vi "gyro-V4.vi"() -> ()   [LabVIEW 2017]
uses:
  plot refs -- filter related.ctl
  cursor winow.ctl
  cursor window action.ctl
  KM_file -- read-write control.ctl
  MFLI controller action.ctl
  sweep parameters.ctl
  cursor action.ctl
  four-corner circle transformation.ctl
  agregator -- action.ctl
  circle corners.ctl
  lorentzian.ctl
  filename-action.ctl
  file -- read-write control.ctl
  publisher action.ctl
  <vilib>/event_ctls.llb/eventvkey.ctl
  wavepacket.ctl
  filter method control.ctl
  peak -- parameters -- complex fit.ctl
  parameters -- scan monitor control.ctl
  pid -- parameters.ctl
panel:
  out "read freq (Hz)":dbl=43834.543279430705 format="%-#11_11f"
  in  "all":enum32{"all", "other"}(tab)
  in  "subtract bgnd !":bool=TRUE
  out "Plot: circle sweep window":cluster{"all rows":dbl[], "all rows":dbl[]}[](graph)
  in  "MFLI mode":T1(tab)=enum."read from disk"
  out "fit is fine":bool=TRUE
  in  "gamma factor":dbl=1.6
  in  "Auto-update sweep window!":bool
  in  "scan type":enum16{"linear", "arctan"}(ring)
  in  "N":i64=2357
  out "sweep time (sec)":dbl=0.07489956999779679
  in  "control sweep!":bool
  out "circle frequency (Hz)":dbl format="%#11_11f"
  out "circle gamma (Hz)":dbl format="%#11_11f"
  out "circle phase (rad)":dbl=nan format="%#11_11f"
  out "circle Q":dbl=nan format="%#11_11f"
  in  "history length":i32=5
  in  "delay-circle(msec)":i64
  out "read Voltage (V)":cdb=8.437092120710226e-06+0.006122499694529841i format="%#10_10f"
  in  "read !":bool
  out "read Voltage X (V)":dbl=8.437092120710226e-06 format="%#11_11f"
  out "read Voltage Y (V)":dbl=0.006122499694529841 format="%#11_11f"
  in  "delay-read (msec)":i64=300
  in  "reqested size":i64=30
  in  "refresh":bool=TRUE
  in  "PID parameters":T2={"P (sec)"=60.0, "I (sec)"=10.0}
  out "left freq (Hz)":dbl=1094842.7980648028
  out "right freq (Hz)":dbl=1109968.9974186728
  out "center freq (Hz)":dbl=1102405.8977417378
  out "window  (Hz)":dbl=15126.199353870004
  in  "talk to MFLI !":bool=TRUE
  in  "aggregator action":T3
  in  "Tab : everything":T4(tab)
  in  "Tab :  Fit controls":enum32{"complex plane", "complex plane 2"}(tab)
  in  "some":dbl=3225.0
  in  "Plot: fragment - filter":cluster{dbl[], dbl[]}[](graph)=[{[], []}, {[], []}, {[], []}, {[], []}]
  in  "scale gauge: Plot: complex plane - filter":dbl(slide)=0.00015000000000000001 min=0.0 max=0.3 step=1e-05 scale=0.0001..0.3 scale format="%#_5g"
  in  "Plot: complex plane - filter":cluster{dbl[], dbl[]}[](graph)=[{[], []}, {[], []}, {[0.0, 0.0, 0.0, 0.0, 0.0, 0.0, 0.0, 0.0, 0.0, 0.0, 0.0, 0.0, 0.0, 0.0, 0.0, 0.0, 0.0, 0.0, 0.0, 0.0, 0.0, 0.0, 0.0, 0.0, 0.0, 0.0, 0.0, 0.0, 0.0, 0.0, 0.0, 0.0, 0.0, 0.0, 0.0, 0.0, 0.0, 0.0, 0.0, 0.0, 0.0, 0.0, 0.0, 0.0, 0.0, 0.0, 0.0, 0.0, 0.0, 0.0, 0.0, 0.0, 0.0, 0.0, 0.0, 0.0, 0.0, 0.0, 0.0, 0.0, 0.0, 0.0, 0.0, 0.0, 0.0, 0.0, 0.0, 0.0, 0.0, 0.0, 0.0, 0.0, 0.0, 0.0, 0.0, 0.0, 0.0, 0.0, 0.0, 0.0, 0.0, 0.0, 0.0, 0.0, 0.0, 0.0, 0.0, 0.0, 0.0, 0.0, 0.0, 0.0, 0.0, 0.0, 0.0, 0.0, 0.0, 0.0, 0.0, 0.0], [0.0, 0.0, 0.0, 0.0, 0.0, 0.0, 0.0, 0.0, 0.0, 0.0, 0.0, 0.0, 0.0, 0.0, 0.0, 0.0, 0.0, 0.0, 0.0, 0.0, 0.0, 0.0, 0.0, 0.0, 0.0, 0.0, 0.0, 0.0, 0.0, 0.0, 0.0, 0.0, 0.0, 0.0, 0.0, 0.0, 0.0, 0.0, 0.0, 0.0, 0.0, 0.0, 0.0, 0.0, 0.0, 0.0, 0.0, 0.0, 0.0, 0.0, 0.0, 0.0, 0.0, 0.0, 0.0, 0.0, 0.0, 0.0, 0.0, 0.0, 0.0, 0.0, 0.0, 0.0, 0.0, 0.0, 0.0, 0.0, 0.0, 0.0, 0.0, 0.0, 0.0, 0.0, 0.0, 0.0, 0.0, 0.0, 0.0, 0.0, 0.0, 0.0, 0.0, 0.0, 0.0, 0.0, 0.0, 0.0, 0.0, 0.0, 0.0, 0.0, 0.0, 0.0, 0.0, 0.0, 0.0, 0.0, 0.0, 0.0]}, {[0.0, 0.0, 0.0], [0.0, 0.0, 0.0]}, {[nan, nan, nan, nan, nan, nan, nan, nan, nan, nan, nan, nan, nan, nan, nan, nan, nan, nan, nan, nan], [nan, nan, nan, nan, nan, nan, nan, nan, nan, nan, nan, nan, nan, nan, nan, nan, nan, nan, nan, nan]}, {[0.0, 0.0, 0.0, 0.0, 0.0, 0.0, 0.0, 0.0, 0.0, 0.0, 0.0, 0.0, 0.0, 0.0, 0.0, 0.0, 0.0, 0.0, 0.0, 0.0], [0.0, 0.0, 0.0, 0.0, 0.0, 0.0, 0.0, 0.0, 0.0, 0.0, 0.0, 0.0, 0.0, 0.0, 0.0, 0.0, 0.0, 0.0, 0.0, 0.0]}]
  out "Plot: dz/domega":cluster{"omega out":dbl[], dbl[]}(graph)
  out "Plot: win omega":T5(graph)
  out "Plot: phase":cluster{"omega out":dbl[], dbl[]}(graph)
  out "Plot: phase around center":cluster{dbl[], dbl[]}[](graph)
  out "Plot: fragment":cluster{dbl[], dbl[]}[](graph)
  out "Plot: complex plane":cluster{dbl[], dbl[]}[](graph)=[{[], []}, {[nan, nan, nan, nan, nan, nan, nan, nan, nan, nan, nan, nan, nan, nan, nan, nan, nan, nan, nan, nan, nan, nan, nan, nan, nan, nan, nan, nan, nan, nan, nan, nan, nan, nan, nan, nan, nan, nan, nan, nan, nan, nan, nan, nan, nan, nan, nan, nan, nan, nan], [nan, nan, nan, nan, nan, nan, nan, nan, nan, nan, nan, nan, nan, nan, nan, nan, nan, nan, nan, nan, nan, nan, nan, nan, nan, nan, nan, nan, nan, nan, nan, nan, nan, nan, nan, nan, nan, nan, nan, nan, nan, nan, nan, nan, nan, nan, nan, nan, nan, nan]}, {[nan, nan, nan, nan, nan, nan, nan, nan, nan, nan, nan, nan, nan, nan, nan, nan, nan, nan, nan, nan], [nan, nan, nan, nan, nan, nan, nan, nan, nan, nan, nan, nan, nan, nan, nan, nan, nan, nan, nan, nan]}, {[nan, nan, nan, nan, nan, nan, nan, nan, nan, nan, nan, nan, nan, nan, nan, nan, nan, nan, nan, nan], [nan, nan, nan, nan, nan, nan, nan, nan, nan, nan, nan, nan, nan, nan, nan, nan, nan, nan, nan, nan]}, {[nan, nan, nan, nan, nan, nan, nan, nan, nan, nan, nan, nan, nan, nan, nan, nan, nan, nan, nan, nan], [nan, nan, nan, nan, nan, nan, nan, nan, nan, nan, nan, nan, nan, nan, nan, nan, nan, nan, nan, nan]}, {[nan, nan, nan, nan, nan, nan, nan, nan, nan, nan, nan, nan, nan, nan, nan, nan, nan, nan, nan, nan], [nan, nan, nan, nan, nan, nan, nan, nan, nan, nan, nan, nan, nan, nan, nan, nan, nan, nan, nan, nan]}, {[], []}]
  in  "scale gauge: Plot: complex plane":dbl(slide)=0.00025 min=0.0 max=0.3 step=1e-05 scale=0.0001..1.0 scale format="%#_2g"
  out "window width (kHz)":dbl=76.27809365793496
  out "window center (kHz)":dbl=3399.029286744401
  out "# of points in window":dbl=953.475933538175
  in  "use fast fit?":bool
  out "pm lorentzian":T6={"Amplitude"=nan, "omega(0)"=0.0, "Gamma"=0.0, "phase"=nan, "Q"=nan, "Norm  Ampl"=nan, "z (inf)"=nan+nani, "4corners"={"z (-pi/2)"=nan+nani, "z(inf)"=nan+nani, "z (pi/2)"=nan+nani, "z center"=nan+nani, "z(0)"=nan+nani, "radius"=nan}} {"z (inf)" format="%#9_9f"; "Q" format="%#9_9f"; "phase" format="%#9_9f"; "Gamma" format="%#9_9f"; "omega(0)" format="%#9_9f"}
  in  "plot staff":enum16{"plot", "do not plot", "a"}(ring)
  in  "fit?":bool=TRUE
  out "Freq out":dbl[](array[numeric])=[17015.929848298583, 17103.637448201425, 17191.34504831743, 17279.052648433433, 17366.76024833628, 17454.46784845228, 17542.175448355123, 17629.88304847113, 17717.590648587135, 17805.298248489977, 17893.00584860598, 17980.713448721985, 18068.421048624827, 18156.128648740832, 18243.83624885684, 18331.54384875968, 18419.251448875686, 18506.959048991688, 18594.66664889453, 18682.374249010536, 18770.08184912654, 18857.789449029384, 18945.497049145386, 19033.20464926139, 19120.912249164234, 19208.61984928024, 19296.32744918308, 19384.035049299087, 19471.742649415093, 19559.45024931793, 19647.157849433937, 19734.865449549943, 19822.573049452785, 19910.28064956879, 19997.988249684793, 20085.69584958764, 20173.40344970364, 20261.111049819647, 20348.81864972249, 20436.526249838495, 20524.2338499545, 20611.94144985734, 20699.649049973345, 20787.356649876187, 20875.064249992192, 20962.771850108198, 21050.47945001104, 21138.187050127046, 21225.894650243048, 21313.60225014589, 21401.309850261896, 21489.0174503779, 21576.725050280744, 21664.432650396746, 21752.14025051275, 21839.847850415594, 21927.5554505316, 22015.263050647605, 22102.970650550447, 22190.678250666453, 22278.38585056929, 22366.093450685297, 22453.801050801303, 22541.508650704145, 22629.21625082015, 22716.923850936153, 22804.631450839, 22892.339050955, 22980.046651071007, 23067.75425097385, 23155.461851089854, 23243.16945120586, 23330.8770511087, 23418.584651224704, 23506.29225134071, 23593.999851243552, 23681.707451359558, 23769.4150512624, 23857.122651378406, 23944.830251494408, 24032.53785139725, 24120.245451513256, 24207.95305162926, 24295.660651532104, 24383.368251648106, 24471.07585176411, 24558.783451666954, 24646.49105178296, 24734.198651898965, 24821.906251801807, 24909.613851917813, 24997.321452033815, 25085.029051936657, 25172.736652052663, 25260.444251955505, 25348.15185207151, 25435.859452187513, 25523.56705209036, 25611.27465220636, 25698.982252322367, 25786.68985222521, 25874.397452341214, 25962.10505245722, 26049.81265236006, 26137.520252476064, 26225.22785259207, 26312.935452494912, 26400.643052610918, 26488.35065272692, 26576.058252629766, 26663.765852745768, 26751.473452861774, 26839.181052764616, 26926.88865288062, 27014.596252783464, 27102.303852899466, 27190.01145301547, 27277.719052918314, 27365.42665303432, 27453.134253150325, 27540.841853053167, 27628.549453169173, 27716.257053285175, 27803.964653188017, 27891.672253304023, 27979.37985342003, 28067.08745332287, 28154.795053438873, 28242.50265355488, 28330.21025345772, 28417.917853573726, 28505.62545347657, 28593.333053592574, 28681.04065370858, 28768.74825361142, 28856.455853727424, 28944.16345384343, 29031.871053746272, 29119.578653862278, 29207.28625397828, 29294.993853881126, 29382.701453997128, 29470.409054113134, 29558.116654015976, 29645.82425413198, 29733.531854247987, 29821.239454150826, 29908.94705426683, 29996.654654169673, 30084.36225428568, 30172.069854401685, 30259.777454304527, 30347.485054420533, 30435.192654536535, 30522.900254439377, 30610.607854555383, 30698.31545467139, 30786.02305457423, 30873.730654690233, 30961.43825480624, 31049.14585470908, 31136.853454825086, 31224.561054941092, 31312.268654843934, 31399.97625495994, 31487.68385486278, 31575.391454978784, 31663.09905509479, 31750.806654997632, 31838.514255113638, 31926.22185522964, 32013.929455132486, 32101.637055248488, 32189.344655364494, 32277.052255267336, 32364.75985538334, 32452.467455499347, 32540.175055402186, 32627.88265551819, 32715.590255634197, 32803.297855537036, 32891.005455653045, 32978.71305555588, 33066.42065567189, 33154.128255787895, 33241.83585569074, 33329.54345580674, 33417.251055922745, 33504.95865582559, 33592.66625594159, 33680.3738560576, 33768.08145596044, 33855.78905607645, 33943.49665619245, 34031.20425609529, 34118.9118562113, 34206.6194563273, 34294.32705623015, 34382.03465634615, 34469.74225646215, 34557.449856365, 34645.157456481, 34732.865056383846, 34820.57265649985, 34908.28025661585, 34995.987856518695, 35083.6954566347, 35171.40305675071, 35259.110656653545, 35346.818256769555, 35434.52585688556, 35522.233456788395, 35609.941056904405, 35697.64865702041, 35785.35625692325, 35873.063857039255, 35960.771457155264, 36048.4790570581, 36136.186657174105, 36223.89425707695, 36311.60185719295, 36399.30945730896, 36487.0170572118, 36574.72465732781, 36662.43225744381, 36750.13985734665, 36837.84745746266, 36925.55505757866, 37013.26265748151, 37100.97025759751, 37188.67785771351, 37276.38545761636, 37364.09305773236, 37451.80065784837, 37539.50825775121, 37627.21585786721, 37714.923457770055, 37802.63105788606, 37890.33865800207, 37978.046257904905, 38065.753858020915, 38153.46145813692, 38241.169058039755, 38328.876658155765, 38416.58425827177, 38504.29185817461, 38591.999458290615, 38679.707058406624, 38767.41465830946, 38855.122258425465, 38942.829858541474, 39030.53745844431, 39118.24505856032, 39205.95265846316, 39293.66025857917, 39381.36785869517, 39469.07545859801, 39556.78305871402, 39644.49065883002, 39732.19825873287, 39819.90585884887, 39907.61345896487, 39995.32105886772, 40083.02865898372, 40170.73625909973, 40258.44385900257, 40346.15145911857, 40433.85905923458, 40521.56665913742, 40609.27425925343, 40696.981859156265, 40784.689459272275, 40872.39705938828, 40960.104659291115, 41047.812259407125, 41135.51985952313, 41223.22745942597, 41310.935059541975, 41398.642659657984, 41486.35025956082, 41574.057859676825, 41661.765459792834, 41749.47305969567, 41837.18065981168, 41924.888259927684, 42012.59585983053, 42100.30345994653, 42188.01105984937, 42275.71865996538, 42363.42626008138, 42451.13385998423, 42538.84146010023, 42626.54906021623, 42714.25666011908, 42801.96426023508, 42889.67186035109, 42977.37946025393, 43065.08706036993, 43152.79466048594, 43240.50226038878, 43328.20986050479, 43415.91746062079, 43503.625060523635, 43591.33266063964, 43679.04026075564, 43766.747860658485, 43854.45546077449, 43942.16306067733, 44029.870660793335, 44117.578260909344, 44205.28586081218, 44292.993460928185, 44380.701061044194, 44468.40866094703, 44556.11626106304, 44643.823861179044, 44731.53146108189, 44819.23906119789, 44906.946661313894, 44994.65426121674, 45082.36186133274, 45170.069461448744, 45257.77706135159, 45345.48466146759, 45433.19226137044, 45520.89986148644, 45608.60746160245, 45696.31506150529, 45784.02266162129, 45871.7302617373, 45959.43786164014, 46047.14546175615, 46134.85306187215, 46222.560661774995, 46310.268261891, 46397.975862007, 46485.683461909844, 46573.39106202585, 46661.098662141856, 46748.806262044694, 46836.513862160704, 46924.22146206354, 47011.929062179544, 47099.636662295554, 47187.34426219839, 47275.0518623144, 47362.759462430404, 47450.46706233325, 47538.17466244925, 47625.882262565254, 47713.5898624681, 47801.2974625841, 47889.005062700104, 47976.71266260295, 48064.42026271895, 48152.12786283496, 48239.8354627378, 48327.54306285381, 48415.25066275665, 48502.95826287265, 48590.66586298866, 48678.3734628915, 48766.08106300751, 48853.78866312351, 48941.496263026354, 49029.20386314236, 49116.91146325836, 49204.619063161204, 49292.32666327721, 49380.034263393216, 49467.741863296054, 49555.449463412064, 49643.157063528066, 49730.864663430904, 49818.572263546914, 49906.27986344975, 49993.98746356576, 50081.695063681764, 50169.40266358461, 50257.11026370061, 50344.817863816614, 50432.52546371946, 50520.23306383546, 50607.940663951464, 50695.64826385431, 50783.35586397031, 50871.06346408632, 50958.77106398916, 51046.47866410517, 51134.18626422117, 51221.89386412401, 51309.60146424002, 51397.30906435602, 51485.01666425887, 51572.72426437487, 51660.431864277714, 51748.13946439372, 51835.84706450972, 51923.554664412564, 52011.26226452857, 52098.969864644576, 52186.677464547414, 52274.385064663424, 52362.092664779426, 52449.800264682264, 52537.507864798274, 52625.215464914276, 52712.92306481712, 52800.63066493312, 52888.338265049126, 52976.04586495197, 53063.75346506797, 53151.46106497082, 53239.16866508682, 53326.87626520282, 53414.58386510567, 53502.29146522167, 53589.99906533768, 53677.70666524052, 53765.41426535653, 53853.12186547253, 53940.82946537537, 54028.53706549138, 54116.24466560738, 54203.95226551023, 54291.65986562623, 54379.36746574224, 54467.07506564508, 54554.78266576108, 54642.490265663924, 54730.197865779926, 54817.905465895936, 54905.613065798774, 54993.32066591478, 55081.028266030786, 55168.735865933624, 55256.44346604963, 55344.151066165636, 55431.85866606848, 55519.56626618448, 55607.273866300486, 55694.98146620333, 55782.68906631933, 55870.39666643534, 55958.10426633818, 56045.81186645418, 56133.51946635703, 56221.22706647303, 56308.93466658904, 56396.64226649188, 56484.34986660789, 56572.05746672389, 56659.76506662673, 56747.47266674274, 56835.18026685874, 56922.887866761586, 57010.59546687759, 57098.3030669936, 57186.010666896436, 57273.71826701244, 57361.42586712845, 57449.133467031286, 57536.841067147296, 57624.548667050134, 57712.25626716614, 57799.963867282146, 57887.671467184984, 57975.37906730099, 58063.086667416996, 58150.79426731984, 58238.50186743584, 58326.209467551846, 58413.91706745469, 58501.62466757069, 58589.3322676867, 58677.03986758954, 58764.74746770554, 58852.45506782155, 58940.16266772439, 59027.8702678404, 59115.5778679564, 59203.28546785925, 59290.99306797525, 59378.70066787809, 59466.4082679941, 59554.1158681101, 59641.823468012946, 59729.53106812895, 59817.23866824496, 59904.946268147796, 59992.6538682638, 60080.36146837981, 60168.069068282646, 60255.776668398656, 60343.48426851466, 60431.1918684175, 60518.899468533506, 60606.60706864951, 60694.31466855235, 60782.022268668356, 60869.7298685712, 60957.4374686872, 61045.145068803206, 61132.85266870605, 61220.56026882205, 61308.26786893806, 61395.9754688409, 61483.6830689569, 61571.39066907291, 61659.09826897575, 61746.80586909176, 61834.51346920776, 61922.22106911061, 62009.92866922661, 62097.63626934261, 62185.34386924546, 62273.05146936146, 62360.759069264306, 62448.46666938031, 62536.17426949632, 62623.881869399156, 62711.58946951516, 62799.29706963117, 62887.004669534006, 62974.712269650016, 63062.41986976602, 63150.12746966886, 63237.835069784865, 63325.54266990087, 63413.25026980371, 63500.957869919715, 63588.66547003572, 63676.37306993856, 63764.080670054565, 63851.78826995741, 63939.49587007341, 64027.20347018942, 64114.91107009226, 64202.61867020826, 64290.32627032427, 64378.03387022711, 64465.74147034312, 64553.44907045912, 64641.15667036197, 64728.86427047797, 64816.57187059397, 64904.27947049682, 64991.98707061282, 65079.69467072883, 65167.40227063167, 65255.10987074768, 65342.817470650516, 65430.52507076652, 65518.23267088253, 65605.94027078537, 65693.64787090138, 65781.35547101738, 65869.06307092022, 65956.77067103623, 66044.47827115223, 66132.18587105507, 66219.89347117108, 66307.60107128708, 66395.30867118992, 66483.01627130593, 66570.72387142193, 66658.43147132477, 66746.13907144078, 66833.84667155679, 66921.55427145962, 67009.26187157563, 67096.96947147847, 67184.67707159447, 67272.38467171049, 67360.09227161332, 67447.79987172934, 67535.50747184534, 67623.21507174817, 67710.92267186419, 67798.63027198019, 67886.33787188304, 67974.04547199904, 68061.75307211504, 68149.46067201789, 68237.16827213389, 68324.87587224989, 68412.58347215274, 68500.29107226874, 68587.99867217158, 68675.70627228759, 68763.41387240359, 68851.12147230643, 68938.82907242244, 69026.53667253844, 69114.24427244128, 69201.95187255729, 69289.65947267329, 69377.36707257613, 69465.07467269214, 69552.78227280814, 69640.48987271098, 69728.19747282699, 69815.905072943, 69903.61267284583, 69991.32027296185, 70079.02787286468, 70166.73547298068, 70254.4430730967, 70342.15067299953, 70429.85827311555, 70517.56587323155, 70605.2734731344, 70692.9810732504, 70780.6886733664, 70868.39627326925, 70956.10387338525, 71043.81147350125, 71131.5190734041, 71219.2266735201, 71306.9342736361, 71394.64187353895, 71482.34947365495, 71570.0570735578, 71657.7646736738, 71745.4722737898, 71833.17987369264, 71920.88747380865, 72008.59507392465, 72096.3026738275, 72184.0102739435, 72271.71787405951, 72359.42547396234, 72447.13307407835, 72534.84067419436, 72622.5482740972, 72710.25587421321, 72797.96347432921, 72885.67107423206, 72973.37867434806, 73061.08627425089, 73148.79387436691, 73236.50147448291, 73324.20907438576, 73411.91667450176, 73499.62427461776, 73587.3318745206, 73675.03947463661, 73762.74707475261, 73850.45467465546, 73938.16227477146, 74025.86987488746, 74113.5774747903, 74201.2850749063, 74288.99267502231, 74376.70027492516, 74464.40787504116, 74552.11547515716, 74639.82307506, 74727.530675176, 74815.23827507885, 74902.94587519486, 74990.65347531086, 75078.3610752137, 75166.0686753297, 75253.77627544572, 75341.48387534855, 75429.19147546457, 75516.89907558057, 75604.6066754834, 75692.31427559942, 75780.02187571542, 75867.72947561827, 75955.43707573427, 76043.14467585027, 76130.85227575312, 76218.55987586912, 76306.26747577197, 76393.97507588797, 76481.68267600397, 76569.39027590682, 76657.09787602282, 76744.80547613882, 76832.51307604167, 76920.22067615767, 77007.92827627367, 77095.63587617652, 77183.34347629252, 77271.05107640852, 77358.75867631136, 77446.46627642737, 77534.17387654338, 77621.88147644621, 77709.58907656223, 77797.29667646506, 77885.00427658106, 77972.71187669708, 78060.41947659991, 78148.12707671593, 78235.83467683193, 78323.54227673478, 78411.24987685078, 78498.95747696678, 78586.66507686963, 78674.37267698563, 78762.08027710163, 78849.78787700448, 78937.49547712048, 79025.20307723648, 79112.91067713933, 79200.61827725533, 79288.32587715817, 79376.03347727418, 79463.74107739018, 79551.44867729302, 79639.15627740903, 79726.86387752503, 79814.57147742787, 79902.27907754388, 79989.98667765988, 80077.69427756272, 80165.40187767873, 80253.10947779474, 80340.81707769757, 80428.52467781358, 80516.2322779296, 80603.93987783242, 80691.64747794844, 80779.35507785127, 80867.06267796729, 80954.77027808329, 81042.47787798612, 81130.18547810214, 81217.89307821814, 81305.60067812099, 81393.30827823699, 81481.01587835299, 81568.72347825584, 81656.43107837184, 81744.13867848784, 81831.84627839069, 81919.55387850669, 82007.26147862269, 82094.96907852554, 82182.67667864154, 82270.38427854438, 82358.09187866039, 82445.79947877639, 82533.50707867923, 82621.21467879524, 82708.92227891124, 82796.62987881408, 82884.33747893009, 82972.0450790461, 83059.75267894893, 83147.46027906495, 83235.16787918095, 83322.87547908378, 83410.5830791998, 83498.2906793158, 83585.99827921865, 83673.70587933465, 83761.41347945065, 83849.1210793535, 83936.8286794695, 84024.53627937235, 84112.24387948835, 84199.95147960435, 84287.6590795072, 84375.3666796232, 84463.0742797392, 84550.78187964205, 84638.48947975805, 84726.19707987405, 84813.9046797769, 84901.6122798929, 84989.3198800089, 85077.02747991175, 85164.73508002775, 85252.44268014375, 85340.1502800466, 85427.8578801626, 85515.56548006544, 85603.27308018145, 85690.98068029746, 85778.6882802003, 85866.3958803163, 85954.10348043231, 86041.81108033514, 86129.51868045116, 86217.22628056716, 86304.93388047001, 86392.64148058601, 86480.34908070201, 86568.05668060486, 86655.76428072086, 86743.47188083686, 86831.17948073971, 86918.88708085571, 87006.59468075856, 87094.30228087456, 87182.00988099056, 87269.7174808934, 87357.42508100941, 87445.13268112541, 87532.84028102826, 87620.54788114426, 87708.25548126026, 87795.9630811631, 87883.67068127911, 87971.37828139513, 88059.08588129796, 88146.79348141396, 88234.50108152998, 88322.2086814328, 88409.91628154882, 88497.62388145165, 88585.33148156767, 88673.03908168367, 88760.7466815865, 88848.45428170252, 88936.16188181852, 89023.86948172137, 89111.57708183737, 89199.28468195337, 89286.99228185622, 89374.69988197222, 89462.40748208822, 89550.11508199107, 89637.82268210707, 89725.53028222307, 89813.23788212592, 89900.94548224192, 89988.65308214477, 90076.36068226077, 90164.06828237677, 90251.77588227962, 90339.48348239562, 90427.19108251162, 90514.89868241447, 90602.60628253047, 90690.31388264647, 90778.02148254932, 90865.72908266532, 90953.43668278134, 91041.14428268417, 91128.85188280018, 91216.55948291619, 91304.26708281902, 91391.97468293503, 91479.68228305104, 91567.38988295388, 91655.09748306988, 91742.80508297273, 91830.51268308873, 91918.22028320473, 92005.92788310758, 92093.63548322358, 92181.34308333958, 92269.05068324243, 92356.75828335843, 92444.46588347443, 92532.17348337728, 92619.88108349328, 92707.58868360928, 92795.29628351213, 92883.00388362813, 92970.71148374413, 93058.41908364698, 93146.12668376298, 93233.83428366583, 93321.54188378183, 93409.24948389785, 93496.95708380068, 93584.66468391668, 93672.3722840327, 93760.07988393553, 93847.78748405154, 93935.49508416755, 94023.20268407039, 94110.9102841864, 94198.6178843024, 94286.32548420524, 94374.03308432124, 94461.74068443725, 94549.44828434009, 94637.1558844561, 94724.86348435894, 94812.57108447494, 94900.27868459094, 94987.98628449379, 95075.69388460979, 95163.4014847258, 95251.10908462864, 95338.81668474464, 95426.52428486064, 95514.23188476349, 95601.93948487949, 95689.6470849955, 95777.35468489834, 95865.06228501434, 95952.76988513036, 96040.47748503319, 96128.18508514919, 96215.89268505204, 96303.60028516804, 96391.30788528406, 96479.01548518689, 96566.7230853029, 96654.4306854189, 96742.13828532174, 96829.84588543775, 96917.55348555376, 97005.2610854566, 97092.9686855726, 97180.6762856886, 97268.38388559145, 97356.09148570745, 97443.79908582346, 97531.5066857263, 97619.2142858423, 97706.92188574515, 97794.62948586115, 97882.33708597715, 97970.04468588, 98057.752285996, 98145.459886112, 98233.16748601485, 98320.87508613085, 98408.58268624685, 98496.2902861497, 98583.9978862657, 98671.70548638172, 98759.41308628455, 98847.12068640057, 98934.82828651657, 99022.5358864194, 99110.24348653542, 99197.95108665142, 99285.65868655426, 99373.36628667027, 99461.07388657311, 99548.78148668911, 99636.48908680512, 99724.19668670796, 99811.90428682396, 99899.61188693997, 99987.31948684281, 100075.02708695881, 100162.73468707482, 100250.44228697766, 100338.14988709366, 100425.85748720967, 100513.56508711251, 100601.27268722851, 100688.98028734452, 100776.68788724736, 100864.39548736336, 100952.10308726621, 101039.81068738221, 101127.51828749821, 101215.22588740106, 101302.93348751706, 101390.64108763308, 101478.34868753591, 101566.05628765191, 101653.76388776793, 101741.47148767076, 101829.17908778678, 101916.88668790278, 102004.59428780562, 102092.30188792163, 102180.00948803763, 102267.71708794047, 102355.42468805648, 102443.13228795932, 102530.83988807532, 102618.54748819133, 102706.25508809417, 102793.96268821017, 102881.67028832618, 102969.37788822902, 103057.08548834502, 103144.79308846103, 103232.50068836387, 103320.20828847987, 103407.91588859588, 103495.62348849872, 103583.33108861472, 103671.03868873074, 103758.74628863357, 103846.45388874957, 103934.16148865242, 104021.86908876842, 104109.57668888444, 104197.28428878727, 104284.99188890329, 104372.69948901929, 104460.40708892212, 104548.11468903814, 104635.82228915414, 104723.52988905698, 104811.23748917299, 104898.94508928899, 104986.65268919183, 105074.36028930784, 105162.06788942384, 105249.77548932668, 105337.48308944269, 105425.19068934553, 105512.89828946153, 105600.60588957753, 105688.31348948038, 105776.02108959638, 105863.72868971238, 105951.43628961523, 106039.14388973123, 106126.85148984723, 106214.55908975008, 106302.26668986608, 106389.97428998208, 106477.68188988493, 106565.38949000093, 106653.09709011695, 106740.80469001978, 106828.5122901358, 106916.2198902518, 107003.92749015463, 107091.63509027065, 107179.34269017348, 107267.0502902895, 107354.7578904055, 107442.46549030834, 107530.17309042434, 107617.88069054035, 107705.5882904432, 107793.2958905592, 107881.0034906752, 107968.71109057804, 108056.41869069404, 108144.12629081005, 108231.8338907129, 108319.5414908289, 108407.2490909449, 108494.95669084774, 108582.66429096374, 108670.37189086659, 108758.07949098259, 108845.7870910986, 108933.49469100144, 109021.20229111744, 109108.90989123346, 109196.61749113629, 109284.32509125229, 109372.03269136831, 109459.74029127114, 109547.44789138716, 109635.15549150316, 109722.863091406, 109810.570691522, 109898.27829163801, 109985.98589154085, 110073.69349165686, 110161.4010915597, 110249.1086916757, 110336.8162917917, 110424.52389169455, 110512.23149181055, 110599.93909192656, 110687.6466918294, 110775.3542919454, 110863.0618920614, 110950.76949196425, 111038.47709208025, 111126.18469219626, 111213.8922920991, 111301.5998922151, 111389.3074923311, 111477.01509223395, 111564.72269234995, 111652.4302922528, 111740.1378923688, 111827.8454924848, 111915.55309238765, 112003.26069250365, 112090.96829261967, 112178.6758925225, 112266.38349263852, 112354.09109275452, 112441.79869265735, 112529.50629277337, 112617.21389288937, 112704.92149279221, 112792.62909290822, 112880.33669302422, 112968.04429292706, 113055.75189304307, 113143.45949294591, 113231.16709306191, 113318.87469317792, 113406.58229308076, 113494.28989319676, 113581.99749331277, 113669.70509321561, 113757.41269333161, 113845.12029344762, 113932.82789335046, 114020.53549346646, 114108.24309358247, 114195.95069348531, 114283.65829360131, 114371.36589371733, 114459.07349362016, 114546.78109373618, 114634.48869385218, 114722.19629375501, 114809.90389387103, 114897.61149377386, 114985.31909388988, 115073.02669400588, 115160.73429390872, 115248.44189402473, 115336.14949414073, 115423.85709404357, 115511.56469415958, 115599.27229427558, 115686.97989417842, 115774.68749429443, 115862.39509441043, 115950.10269431327, 116037.81029442928, 116125.51789454528, 116213.22549444812, 116300.93309456413, 116388.64069446697, 116476.34829458297, 116564.05589469898, 116651.76349460182, 116739.47109471782, 116827.17869483383, 116914.88629473667, 117002.59389485267, 117090.30149496869, 117178.00909487152, 117265.71669498752, 117353.42429510354, 117441.13189500637, 117528.83949512239, 117616.54709523839, 117704.25469514124, 117791.96229525724, 117879.66989516007, 117967.37749527609, 118055.08509539209, 118142.79269529493, 118230.50029541094, 118318.20789552694, 118405.91549542978, 118493.62309554579, 118581.33069566179, 118669.03829556463, 118756.74589568064, 118844.45349579664, 118932.16109569948, 119019.86869581549, 119107.57629593149, 119195.28389583433, 119282.99149595034, 119370.69909585318, 119458.40669596918, 119546.11429608519, 119633.82189598803, 119721.52949610403, 119809.23709622005, 119896.94469612288, 119984.6522962389, 120072.3598963549, 120160.06749625773, 120247.77509637375, 120335.48269648975, 120423.1902963926, 120510.8978965086, 120598.6054966246, 120686.31309652745, 120774.02069664345, 120861.7282965463, 120949.4358966623, 121037.1434967783, 121124.85109668114, 121212.55869679715, 121300.26629691315, 121387.973896816, 121475.681496932, 121563.389097048, 121651.09669695084, 121738.80429706685, 121826.51189718285, 121914.2194970857, 122001.9270972017, 122089.6346973177, 122177.34229722054, 122265.04989733655, 122352.75749723939, 122440.4650973554, 122528.17269747141, 122615.88029737424, 122703.58789749024, 122791.29549760626, 122879.00309750909, 122966.71069762511, 123054.41829774111, 123142.12589764396, 123229.83349775996, 123317.54109787596, 123405.2486977788, 123492.95629789481, 123580.66389801081, 123668.37149791366, 123756.07909802966, 123843.78669814566, 123931.4942980485, 124019.20189816451, 124106.90949806735, 124194.61709818336, 124282.32469829936, 124370.0322982022, 124457.7398983182, 124545.44749843421, 124633.15509833705, 124720.86269845306, 124808.57029856907, 124896.2778984719, 124983.9854985879, 125071.69309870392, 125159.40069860675, 125247.10829872277, 125334.81589883877, 125422.52349874162, 125510.23109885762, 125597.93869876045, 125685.64629887647, 125773.35389899247, 125861.06149889532, 125948.76909901132, 126036.47669912732, 126124.18429903017, 126211.89189914617, 126299.59949926217, 126387.30709916502, 126475.01469928102, 126562.72229939702, 126650.42989929987, 126738.13749941587, 126825.84509953187, 126913.55269943472, 127001.26029955072, 127088.96789945356, 127176.67549956957, 127264.38309968557, 127352.09069958841, 127439.79829970442, 127527.50589982042, 127615.21349972326, 127702.92109983927, 127790.62869995528, 127878.33629985811, 127966.04389997413, 128053.75150009013, 128141.45909999296, 128229.16670010898, 128316.87430022498, 128404.58190012783, 128492.28950024383, 128579.99710014668, 128667.70470026268, 128755.41230037868, 128843.11990028153, 128930.82750039753, 129018.53510051353, 129106.24270041638, 129193.95030053238, 129281.65790064838, 129369.36550055123, 129457.07310066723, 129544.78070078323, 129632.48830068608, 129720.19590080208, 129807.90350091808, 129895.61110082093, 129983.31870093693, 130071.02630083977, 130158.73390095578, 130246.4415010718, 130334.14910097462, 130421.85670109063, 130509.56430120664, 130597.27190110947, 130684.97950122549, 130772.6871013415, 130860.39470124434, 130948.10230136034, 131035.80990147634, 131123.5175013792, 131211.2251014952, 131298.9327016112, 131386.64030151404, 131474.34790163004, 131562.05550174604, 131649.7631016489, 131737.4707017649, 131825.17830166774, 131912.88590178374, 132000.59350189974, 132088.3011018026, 132176.0087019186, 132263.7163020346, 132351.42390193744, 132439.13150205344, 132526.83910216944, 132614.5467020723, 132702.2543021883, 132789.9619023043, 132877.66950220714, 132965.37710232314, 133053.08470243914, 133140.792302342, 133228.499902458, 133316.20750236083, 133403.91510247684, 133491.62270259284, 133579.33030249568, 133667.0379026117, 133754.7455027277, 133842.45310263053, 133930.16070274654, 134017.86830286257, 134105.57590276538, 134193.2835028814, 134280.99110299742, 134368.69870290023, 134456.40630301627, 134544.11390313227, 134631.82150303508, 134719.52910315112, 134807.23670305393, 134894.94430316996, 134982.65190328597, 135070.3595031888, 135158.0671033048, 135245.77470342082, 135333.48230332366, 135421.18990343966, 135508.89750355567, 135596.6051034585, 135684.3127035745, 135772.02030369051, 135859.72790359336, 135947.43550370936, 136035.14310382536, 136122.8507037282, 136210.5583038442, 136298.26590374706, 136385.97350386306, 136473.68110397906, 136561.3887038819, 136649.0963039979, 136736.8039041139, 136824.51150401676, 136912.21910413276, 136999.92670424876, 137087.6343041516, 137175.3419042676, 137263.0495043836, 137350.75710428646, 137438.46470440246, 137526.17230451846, 137613.8799044213, 137701.5875045373, 137789.29510444016, 137877.00270455616, 137964.71030467216, 138052.417904575, 138140.125504691, 138227.833104807, 138315.54070470986, 138403.24830482586, 138490.95590494186, 138578.6635048447, 138666.3711049607, 138754.0787050767, 138841.78630497956, 138929.49390509556, 139017.20150521156, 139104.9091051144, 139192.6167052304, 139280.32430534644, 139368.03190524926, 139455.73950536526, 139543.4471052681, 139631.1547053841, 139718.86230550014, 139806.56990540295, 139894.27750551898, 139981.985105635, 140069.69270553783, 140157.40030565383, 140245.10790576984, 140332.81550567268, 140420.52310578868, 140508.2307059047, 140595.93830580753, 140683.64590592353, 140771.35350603954, 140859.06110594238, 140946.76870605838, 141034.47630596123, 141122.18390607723, 141209.89150619323, 141297.59910609608, 141385.30670621208, 141473.01430632808, 141560.72190623093, 141648.42950634693, 141736.13710646293, 141823.84470636578, 141911.55230648178, 141999.25990659778, 142086.96750650063, 142174.67510661663, 142262.38270673263, 142350.09030663548, 142437.79790675148, 142525.50550665433, 142613.21310677033, 142700.92070688633, 142788.62830678918, 142876.33590690518, 142964.04350702118, 143051.75110692403, 143139.45870704003, 143227.16630715603, 143314.87390705888, 143402.58150717488, 143490.28910729088, 143577.99670719373, 143665.70430730973, 143753.41190742573, 143841.11950732858, 143928.82710744458, 144016.53470734743, 144104.24230746343, 144191.94990757943, 144279.65750748228, 144367.36510759828, 144455.07270771428, 144542.78030761713, 144630.48790773313, 144718.19550784916, 144805.90310775198, 144893.610707868, 144981.318307984, 145069.02590788683, 145156.73350800286, 145244.44110811886, 145332.1487080217, 145419.8563081377, 145507.56390804052, 145595.27150815655, 145682.97910827256, 145770.6867081754, 145858.3943082914, 145946.1019084074, 146033.80950831025, 146121.51710842625, 146209.22470854226, 146296.9323084451, 146384.6399085611, 146472.3475086771, 146560.05510857995, 146647.76270869595, 146735.47030881196, 146823.1779087148, 146910.8855088308, 146998.5931089468, 147086.30070884965, 147174.00830896565, 147261.7159088685, 147349.4235089845, 147437.1311091005, 147524.83870900335, 147612.54630911935, 147700.25390923535, 147787.9615091382, 147875.6691092542, 147963.3767093702, 148051.08430927305, 148138.79190938905, 148226.49950950505, 148314.2071094079, 148401.9147095239, 148489.6223096399, 148577.32990954275, 148665.03750965875, 148752.7451095616, 148840.4527096776, 148928.1603097936, 149015.86790969645, 149103.57550981245, 149191.28310992845, 149278.9907098313, 149366.6983099473, 149454.4059100633, 149542.11350996615, 149629.82111008215, 149717.52871019818, 149805.236310101, 149892.943910217, 149980.65151033303, 150068.35911023585, 150156.06671035188, 150243.7743102547, 150331.4819103707, 150419.18951048673, 150506.89711038955, 150594.60471050558, 150682.31231062158, 150770.01991052442, 150857.72751064043, 150945.43511075643, 151033.14271065927, 151120.85031077528, 151208.55791089128, 151296.26551079412, 151383.97311091013, 151471.68071102613, 151559.38831092897, 151647.09591104498, 151734.80351094782, 151822.51111106382, 151910.21871117983, 151997.92631108267, 152085.63391119867, 152173.34151131468, 152261.04911121752, 152348.75671133352, 152436.46431144953, 152524.17191135237, 152611.87951146837, 152699.58711158438, 152787.29471148722, 152875.00231160322, 152962.70991171923, 153050.41751162207, 153138.12511173807, 153225.83271164092, 153313.54031175692, 153401.24791187292, 153488.95551177577, 153576.66311189177, 153664.37071200777, 153752.07831191062, 153839.78591202662, 153927.49351214262, 154015.20111204547, 154102.90871216147, 154190.61631227747, 154278.32391218032, 154366.03151229632, 154453.73911241232, 154541.44671231517, 154629.15431243117, 154716.86191254717, 154804.56951245002, 154892.27711256602, 154979.98471246887, 155067.69231258487, 155155.39991270087, 155243.10751260372, 155330.81511271972, 155418.52271283575, 155506.23031273857, 155593.9379128546, 155681.6455129706, 155769.35311287345, 155857.06071298945, 155944.76831310545, 156032.4759130083, 156120.1835131243, 156207.8911132403, 156295.59871314315, 156383.30631325915, 156471.013913162, 156558.721513278, 156646.429113394, 156734.13671329684, 156821.84431341285, 156909.55191352885, 156997.2595134317, 157084.9671135477, 157172.6747136637, 157260.38231356654, 157348.08991368255, 157435.79751379855, 157523.5051137014, 157611.2127138174, 157698.9203139334, 157786.62791383624, 157874.33551395225, 157962.0431138551, 158049.7507139711, 158137.4583140871, 158225.16591398994, 158312.87351410594, 158400.58111422195, 158488.2887141248, 158575.9963142408, 158663.7039143568, 158751.41151425964, 158839.11911437564, 158926.82671449165, 159014.5343143945, 159102.2419145105, 159189.9495146265, 159277.65711452934, 159365.36471464534, 159453.0723145482, 159540.7799146642, 159628.4875147802, 159716.19511468304, 159803.90271479904, 159891.61031491504, 159979.3179148179, 160067.0255149339, 160154.7331150499, 160242.44071495274, 160330.14831506874, 160417.85591518477, 160505.5635150876, 160593.27111520362, 160680.97871531962, 160768.68631522244, 160856.39391533847, 160944.1015152413, 161031.80911535732, 161119.51671547332, 161207.22431537614, 161294.93191549217, 161382.63951560817, 161470.34711551102, 161558.05471562702, 161645.76231574302, 161733.46991564587, 161821.17751576187, 161908.88511587787, 161996.59271578072, 162084.30031589672, 162172.00791601272, 162259.71551591557, 162347.42311603157, 162435.1307159344, 162522.83831605042, 162610.54591616642, 162698.25351606926, 162785.96111618527, 162873.66871630127, 162961.3763162041, 163049.08391632012, 163136.79151643612, 163224.49911633896, 163312.20671645497, 163399.91431657097, 163487.6219164738, 163575.32951658982, 163663.03711670582, 163750.74471660866, 163838.45231672467, 163926.15991684067, 164013.8675167435, 164101.57511685952, 164189.28271676236, 164276.99031687836, 164364.69791699437, 164452.4055168972, 164540.1131170132, 164627.82071712922, 164715.52831703206, 164803.23591714806, 164890.94351726407, 164978.6511171669, 165066.3587172829, 165154.06631739892, 165241.77391730176, 165329.48151741776, 165417.1891175338, 165504.8967174366, 165592.6043175526, 165680.31191745546, 165768.01951757146, 165855.7271176875, 165943.4347175903, 166031.1423177063, 166118.84991782234, 166206.55751772516, 166294.2651178412, 166381.9727179572, 166469.68031786004, 166557.38791797604, 166645.09551809204, 166732.8031179949, 166820.5107181109, 166908.2183182269, 166995.92591812974, 167083.63351824574, 167171.3411181486, 167259.0487182646, 167346.7563183806, 167434.46391828344, 167522.17151839944, 167609.87911851544, 167697.5867184183, 167785.2943185343, 167873.0019186503, 167960.70951855314, 168048.41711866914, 168136.12471878514, 168223.832318688, 168311.539918804, 168399.24751892, 168486.95511882284, 168574.66271893884, 168662.37031884168, 168750.0779189577, 168837.7855190737, 168925.49311897653, 169013.20071909254, 169100.90831920854, 169188.61591911138, 169276.3235192274, 169364.0311193434, 169451.73871924623, 169539.44631936224, 169627.15391947824, 169714.86151938108, 169802.5691194971, 169890.2767196131, 169977.98431951593, 170065.69191963194, 170153.39951953478, 170241.10711965078, 170328.8147197668, 170416.52231966963, 170504.22991978563, 170591.93751990164, 170679.64511980448, 170767.35271992048, 170855.0603200365, 170942.76791993933, 171030.47552005533, 171118.18312017136, 171205.89072007418, 171293.5983201902, 171381.30592030621, 171469.01352020906, 171556.72112032506, 171644.42872044106, 171732.1363203439, 171819.8439204599, 171907.55152036276, 171995.25912047876, 172082.96672059476, 172170.6743204976, 172258.3819206136, 172346.0895207296, 172433.79712063246, 172521.50472074846, 172609.21232086446, 172696.9199207673, 172784.6275208833, 172872.3351209993, 172960.04272090216, 173047.75032101816, 173135.45792113416, 173223.165521037, 173310.873121153, 173398.58072105586, 173486.28832117186, 173573.99592128786, 173661.7035211907, 173749.4111213067, 173837.1187214227, 173924.82632132556, 174012.53392144156, 174100.24152155756, 174187.9491214604, 174275.6567215764, 174363.3643216924, 174451.07192159526, 174538.77952171126, 174626.48712182726, 174714.1947217301, 174801.9023218461, 174889.60992174895, 174977.31752186496, 175065.02512198096, 175152.7327218838, 175240.4403219998, 175328.1479221158, 175415.85552201865, 175503.56312213466, 175591.27072225066, 175678.9783221535, 175766.6859222695, 175854.3935223855, 175942.10112228835, 176029.80872240436, 176117.5163225204, 176205.2239224232, 176292.93152253923, 176380.63912244205, 176468.34672255805, 176556.05432267408, 176643.7619225769, 176731.46952269293, 176819.17712280893, 176906.88472271175, 176994.59232282778, 177082.29992294378, 177170.00752284663, 177257.71512296263, 177345.42272307863, 177433.13032298148, 177520.83792309748, 177608.54552321348, 177696.25312311633, 177783.96072323233, 177871.66832313518, 177959.37592325118, 178047.08352336718, 178134.79112327003, 178222.49872338603, 178310.20632350203, 178397.91392340488, 178485.62152352088, 178573.32912363688, 178661.03672353973, 178748.74432365573, 178836.45192377173, 178924.15952367458, 179011.86712379058, 179099.57472390658, 179187.28232380943, 179274.98992392543, 179362.69752404143, 179450.40512394428, 179538.11272406028, 179625.82032396313, 179713.52792407913, 179801.23552419513, 179888.94312409798, 179976.65072421398, 180064.35832432998, 180152.06592423283, 180239.77352434883, 180327.48112446483, 180415.18872436768, 180502.89632448368, 180590.60392459968, 180678.31152450253, 180766.01912461853, 180853.72672473453, 180941.43432463738, 181029.14192475338, 181116.84952465622, 181204.55712477223, 181292.26472488823, 181379.97232479107, 181467.67992490708, 181555.3875250231, 181643.09512492592, 181730.80272504193, 181818.51032515796, 181906.21792506077, 181993.9255251768, 182081.6331252928, 182169.34072519565, 182257.04832531165, 182344.75592542766, 182432.4635253305, 182520.1711254465, 182607.87872534935, 182695.58632546535, 182783.29392558135, 182871.0015254842, 182958.7091256002, 183046.4167257162, 183134.12432561905, 183221.83192573505, 183309.53952585105, 183397.2471257539, 183484.9547258699, 183572.6623259859, 183660.36992588875, 183748.07752600475, 183835.78512612075, 183923.4927260236, 184011.2003261396, 184098.90792604245, 184186.61552615845, 184274.32312627445, 184362.0307261773, 184449.7383262933, 184537.4459264093, 184625.15352631215, 184712.86112642815, 184800.56872654415, 184888.276326447, 184975.983926563, 185063.691526679, 185151.39912658185, 185239.10672669785, 185326.81432681385, 185414.5219267167, 185502.2295268327, 185589.93712673555, 185677.64472685155, 185765.35232696755, 185853.0599268704, 185940.7675269864, 186028.4751271024, 186116.18272700525, 186203.89032712125, 186291.59792723725, 186379.3055271401, 186467.0131272561, 186554.7207273721, 186642.42832727495, 186730.13592739095, 186817.84352750698, 186905.5511274098, 186993.25872752583, 187080.96632764183, 187168.67392754467, 187256.38152766068, 187344.0891275635, 187431.79672767952, 187519.50432779553, 187607.21192769837, 187694.91952781437, 187782.62712793038, 187870.33472783322, 187958.04232794922, 188045.74992806523, 188133.45752796807, 188221.16512808407, 188308.87272820008, 188396.58032810292, 188484.28792821892, 188571.99552833493, 188659.70312823777, 188747.41072835377, 188835.11832825662, 188922.82592837262, 189010.53352848862, 189098.24112839147, 189185.94872850747, 189273.65632862347, 189361.36392852632, 189449.07152864232, 189536.77912875832, 189624.48672866117, 189712.19432877717, 189799.90192889317, 189887.60952879602, 189975.31712891202, 190063.02472902802, 190150.73232893087, 190238.43992904687, 190326.14752894972, 190413.85512906572, 190501.56272918172, 190589.27032908457, 190676.97792920057, 190764.68552931657, 190852.39312921942, 190940.10072933542, 191027.80832945142, 191115.51592935427, 191203.22352947027, 191290.93112958627, 191378.63872948912, 191466.34632960512, 191554.05392972112, 191641.76152962397, 191729.46912973997, 191817.17672964282, 191904.88432975882, 191992.59192987485, 192080.29952977767, 192168.00712989367, 192255.7147300097, 192343.42232991252, 192431.12993002855, 192518.83753014455, 192606.54513004737, 192694.2527301634, 192781.9603302794, 192869.66793018224, 192957.37553029825, 193045.08313041425, 193132.7907303171, 193220.4983304331, 193308.20593033594, 193395.91353045194, 193483.62113056795, 193571.3287304708, 193659.0363305868, 193746.7439307028, 193834.45153060564, 193922.15913072164, 194009.86673083765, 194097.5743307405, 194185.2819308565, 194272.9895309725, 194360.69713087534, 194448.40473099134, 194536.11233110735, 194623.8199310102, 194711.5275311262, 194799.2351312422, 194886.94273114504, 194974.65033126104, 195062.3579311639, 195150.0655312799, 195237.7731313959, 195325.48073129874, 195413.18833141474, 195500.89593153074, 195588.6035314336, 195676.3111315496, 195764.0187316656, 195851.72633156844, 195939.43393168444, 196027.14153180044, 196114.8491317033, 196202.5567318193, 196290.2643319353, 196377.97193183814, 196465.67953195414, 196553.387131857, 196641.094731973, 196728.802332089, 196816.50993199184, 196904.21753210784, 196991.92513222384, 197079.6327321267, 197167.3403322427, 197255.04793235872, 197342.75553226154, 197430.46313237754, 197518.17073249357, 197605.8783323964, 197693.58593251242, 197781.29353262842, 197869.00113253127, 197956.70873264727, 198044.4163325501, 198132.12393266612, 198219.83153278212, 198307.53913268496, 198395.24673280097, 198482.95433291697, 198570.6619328198, 198658.36953293582, 198746.07713305182, 198833.78473295466, 198921.49233307067, 199009.19993318667, 199096.9075330895, 199184.61513320552, 199272.32273332152, 199360.03033322436, 199447.73793334037, 199535.4455332432, 199623.1531333592, 199710.86073347522, 199798.56833337806, 199886.27593349406, 199973.98353361007, 200061.6911335129, 200149.3987336289, 200237.10633374492, 200324.81393364776, 200412.52153376376, 200500.22913387977, 200587.9367337826, 200675.6443338986, 200763.35193401462, 200851.05953391746, 200938.76713403346, 201026.4747339363, 201114.1823340523, 201201.8899341683, 201289.59753407116, 201377.30513418716, 201465.01273430316, 201552.720334206, 201640.427934322, 201728.135534438, 201815.84313434086, 201903.55073445686, 201991.25833457286, 202078.9659344757, 202166.6735345917, 202254.3811347077, 202342.08873461056, 202429.79633472656, 202517.5039346294, 202605.2115347454, 202692.91913486144, 202780.62673476426, 202868.3343348803, 202956.0419349963, 203043.7495348991, 203131.45713501514, 203219.16473513114, 203306.872335034, 203394.57993515, 203482.287535266, 203569.99513516884, 203657.70273528484, 203745.41033540084, 203833.1179353037, 203920.8255354197, 204008.5331355357, 204096.24073543854, 204183.94833555454, 204271.65593545738, 204359.3635355734, 204447.0711356894, 204534.77873559223, 204622.48633570824, 204710.19393582424, 204797.90153572708, 204885.6091358431, 204973.3167359591, 205061.02433586193, 205148.73193597794, 205236.43953609394, 205324.14713599678, 205411.8547361128, 205499.5623362288, 205587.26993613163, 205674.97753624764, 205762.68513615048, 205850.39273626648, 205938.1003363825, 206025.80793628533, 206113.51553640133, 206201.22313651734, 206288.93073642018, 206376.63833653618, 206464.3459366522, 206552.05353655503, 206639.76113667103, 206727.46873678704, 206815.17633668988, 206902.88393680588, 206990.5915369219, 207078.29913682473, 207166.00673694073, 207253.71433684358, 207341.42193695958, 207429.12953707558, 207516.83713697843, 207604.54473709443, 207692.25233721046, 207779.95993711328, 207867.66753722928, 207955.3751373453, 208043.08273724813, 208130.79033736416, 208218.49793748016, 208306.20553738298, 208393.913137499, 208481.620737615, 208569.32833751786, 208657.03593763386, 208744.7435375367, 208832.4511376527, 208920.1587377687, 209007.86633767156, 209095.57393778756, 209183.28153790356, 209270.9891378064, 209358.6967379224, 209446.4043380384, 209534.11193794126, 209621.81953805726, 209709.52713817326, 209797.2347380761, 209884.9423381921, 209972.6499383081, 210060.35753821096, 210148.06513832696, 210235.7727382298, 210323.4803383458, 210411.1879384618, 210498.89553836465, 210586.60313848066, 210674.31073859666, 210762.0183384995, 210849.7259386155, 210937.4335387315, 211025.14113863435, 211112.84873875036, 211200.55633886636, 211288.2639387692, 211375.9715388852, 211463.6791390012, 211551.38673890405, 211639.09433902006, 211726.80193913606, 211814.5095390389, 211902.2171391549, 211989.92473905775, 212077.63233917375, 212165.33993928976, 212253.0475391926, 212340.7551393086, 212428.4627394246, 212516.17033932745, 212603.87793944345, 212691.58553955946, 212779.2931394623, 212867.0007395783, 212954.70833969433, 213042.41593959715, 213130.12353971315, 213217.83113982918, 213305.538739732, 213393.24633984803, 213480.95393975085, 213568.66153986688, 213656.36913998288, 213744.07673988573, 213831.78434000173, 213919.49194011773, 214007.19954002058, 214094.90714013658, 214182.61474025258, 214270.32234015543, 214358.02994027143, 214445.73754038743, 214533.44514029028, 214621.15274040628, 214708.86034052228, 214796.56794042513, 214884.27554054113, 214971.98314044398, 215059.69074055998, 215147.39834067598, 215235.10594057883, 215322.81354069483, 215410.52114081083, 215498.22874071368, 215585.93634082968, 215673.64394094568, 215761.35154084853, 215849.05914096453, 215936.76674108053, 216024.47434098338, 216112.18194109938, 216199.88954121538, 216287.59714111823, 216375.30474123423, 216463.01234113707, 216550.71994125308, 216638.42754136908, 216726.13514127192, 216813.84274138793, 216901.55034150393, 216989.25794140677, 217076.96554152278, 217164.67314163878, 217252.38074154162, 217340.08834165763, 217427.79594177363, 217515.50354167647, 217603.21114179248, 217690.91874190848, 217778.62634181132, 217866.33394192733, 217954.04154183017, 218041.74914194617, 218129.45674206218, 218217.16434196502, 218304.87194208102, 218392.57954219705, 218480.28714209987, 218567.9947422159, 218655.7023423319, 218743.40994223472, 218831.11754235075, 218918.82514246675, 219006.5327423696, 219094.2403424856, 219181.9479426016, 219269.65554250445, 219357.36314262045, 219445.07074273645, 219532.7783426393, 219620.4859427553, 219708.19354265815, 219795.90114277415, 219883.60874289015, 219971.316342793, 220059.023942909, 220146.731543025, 220234.43914292785, 220322.14674304385, 220409.85434315985, 220497.5619430627, 220585.2695431787, 220672.9771432947, 220760.68474319755, 220848.39234331355, 220936.09994342955, 221023.8075433324, 221111.5151434484, 221199.22274335125, 221286.93034346725, 221374.63794358325, 221462.3455434861, 221550.0531436021, 221637.7607437181, 221725.46834362095, 221813.17594373695, 221900.88354385295, 221988.5911437558, 222076.2987438718, 222164.0063439878, 222251.71394389065, 222339.42154400665, 222427.12914412265, 222514.8367440255, 222602.5443441415, 222690.25194404434, 222777.95954416035, 222865.66714427635, 222953.3747441792, 223041.0823442952, 223128.7899444112, 223216.49754431404, 223304.20514443005, 223391.91274454608, 223479.6203444489, 223567.3279445649, 223655.03554468093, 223742.74314458374, 223830.45074469977, 223918.15834481578, 224005.8659447186, 224093.57354483462, 224181.28114473744, 224268.98874485347, 224356.69634496947, 224444.40394487232, 224532.11154498832, 224619.81914510432, 224707.52674500717, 224795.23434512317, 224882.94194523917, 224970.64954514202, 225058.35714525802, 225146.06474537402, 225233.77234527687, 225321.47994539287, 225409.18754550887, 225496.89514541172, 225584.60274552772, 225672.31034543057, 225760.01794554657, 225847.72554566257, 225935.43314556542, 226023.14074568142, 226110.84834579742, 226198.55594570027, 226286.26354581627, 226373.97114593227, 226461.67874583512, 226549.38634595112, 226637.09394606712, 226724.80154596997, 226812.50914608597, 226900.21674620197, 226987.92434610482, 227075.63194622082, 227163.33954633682, 227251.04714623967, 227338.75474635567, 227426.46234625852, 227514.16994637452, 227601.87754649052, 227689.58514639336, 227777.29274650937, 227865.00034662537, 227952.70794652821, 228040.41554664422, 228128.12314676022, 228215.83074666306, 228303.53834677907, 228391.24594689507, 228478.95354679791, 228566.66114691392, 228654.36874702995, 228742.07634693276, 228829.78394704877, 228917.4915469516, 229005.19914706761, 229092.90674718365, 229180.61434708646, 229268.3219472025, 229356.0295473185, 229443.73714722134, 229531.44474733734, 229619.15234745335, 229706.8599473562, 229794.5675474722, 229882.2751475882, 229969.98274749104, 230057.69034760704, 230145.39794772305, 230233.1055476259, 230320.8131477419, 230408.52074764474, 230496.22834776074, 230583.93594787674, 230671.6435477796, 230759.3511478956, 230847.0587480116, 230934.76634791444, 231022.47394803044, 231110.18154814644, 231197.8891480493, 231285.5967481653, 231373.3043482813, 231461.01194818414, 231548.71954830014, 231636.42714841614, 231724.134748319, 231811.842348435, 231899.54994833784, 231987.25754845384, 232074.96514856984, 232162.6727484727, 232250.3803485887, 232338.0879487047, 232425.79554860754, 232513.50314872354, 232601.21074883954, 232688.9183487424, 232776.6259488584, 232864.3335489744, 232952.04114887724, 233039.74874899324, 233127.45634910924, 233215.1639490121, 233302.8715491281, 233390.57914903093, 233478.28674914694, 233565.99434926294, 233653.70194916578, 233741.4095492818, 233829.1171493978, 233916.82474930063, 234004.53234941664, 234092.23994953267, 234179.94754943548, 234267.65514955152, 234355.36274966752, 234443.07034957033, 234530.77794968637, 234618.48554980237, 234706.1931497052, 234793.90074982122, 234881.60834993722, 234969.31594984006, 235057.02354995607, 235144.7311498589, 235232.4387499749, 235320.14635009092, 235407.85394999376, 235495.56155010976, 235583.26915022577, 235670.9767501286, 235758.6843502446, 235846.39195036062, 235934.09955026346, 236021.80715037946, 236109.51475049547, 236197.2223503983, 236284.9299505143, 236372.63755063032, 236460.34515053316, 236548.05275064916, 236635.760350552, 236723.467950668, 236811.175550784, 236898.88315068686, 236986.59075080286, 237074.29835091886, 237162.0059508217, 237249.7135509377, 237337.4211510537, 237425.12875095656, 237512.83635107256, 237600.54395118856, 237688.2515510914, 237775.9591512074, 237863.6667513234, 237951.37435122626, 238039.08195134226, 238126.7895512451, 238214.4971513611, 238302.2047514771, 238389.91235137996, 238477.61995149596, 238565.32755161196, 238653.0351515148, 238740.7427516308, 238828.4503517468, 238916.15795164966, 239003.86555176566, 239091.5731518817, 239179.2807517845, 239266.9883519005, 239354.69595201654, 239442.40355191936, 239530.1111520354, 239617.8187519382, 239705.5263520542, 239793.23395217024, 239880.94155207305, 239968.6491521891, 240056.3567523051, 240144.06435220793, 240231.77195232394, 240319.47955243994, 240407.18715234278, 240494.8947524588, 240582.6023525748, 240670.30995247763, 240758.01755259364, 240845.72515270964, 240933.43275261248, 241021.1403527285, 241108.84795263133, 241196.55555274733, 241284.26315286334, 241371.97075276618, 241459.67835288218, 241547.3859529982, 241635.09355290103, 241722.80115301703, 241810.50875313304, 241898.21635303588, 241985.92395315188, 242073.6315532679, 242161.33915317073, 242249.04675328673, 242336.75435340274, 242424.46195330558, 242512.16955342158, 242599.87715332443, 242687.58475344043, 242775.29235355643, 242862.99995345928, 242950.70755357528, 243038.41515369128, 243126.12275359413, 243213.83035371013, 243301.53795382613, 243389.24555372898, 243476.95315384498, 243564.66075396098, 243652.36835386383, 243740.07595397983, 243827.78355409583, 243915.49115399868, 244003.19875411468, 244090.90635423068, 244178.61395413353, 244266.32155424953, 244354.02915415238, 244441.73675426838, 244529.44435438438, 244617.15195428723, 244704.85955440323, 244792.56715451926, 244880.27475442208, 244967.9823545381, 245055.6899546541, 245143.39755455696, 245231.10515467296, 245318.81275478896, 245406.5203546918, 245494.2279548078, 245581.9355549238, 245669.64315482666, 245757.35075494266, 245845.0583548455, 245932.7659549615, 246020.4735550775, 246108.18115498035, 246195.88875509636, 246283.59635521236, 246371.3039551152, 246459.0115552312, 246546.7191553472, 246634.42675525005, 246722.13435536606, 246809.84195548206, 246897.5495553849, 246985.2571555009, 247072.9647556169, 247160.67235551975, 247248.37995563576, 247336.0875555386, 247423.7951556546, 247511.5027557706, 247599.21035567345, 247686.91795578945, 247774.62555590546, 247862.3331558083, 247950.0407559243, 248037.7483560403, 248125.45595594315, 248213.16355605915, 248300.87115617516, 248388.578756078, 248476.286356194, 248563.99395631, 248651.70155621285, 248739.40915632885, 248827.1167562317, 248914.8243563477, 249002.5319564637, 249090.23955636655, 249177.94715648255, 249265.65475659855, 249353.3623565014, 249441.0699566174, 249528.7775567334, 249616.48515663625, 249704.19275675225, 249791.90035686828, 249879.6079567711, 249967.31555688713, 250055.02315700313, 250142.73075690595, 250230.43835702198, 250318.1459569248, 250405.85355704083, 250493.56115715683, 250581.26875705965, 250668.97635717568, 250756.68395729168, 250844.39155719453, 250932.09915731053, 251019.80675742653, 251107.51435732938, 251195.22195744538, 251282.92955756138, 251370.63715746423, 251458.34475758023, 251546.05235769623, 251633.75995759908, 251721.46755771508, 251809.17515783108, 251896.88275773393, 251984.59035784993, 252072.29795775277, 252160.00555786878, 252247.71315798478, 252335.42075788762, 252423.12835800363, 252510.83595811963, 252598.54355802247, 252686.25115813848, 252773.95875825448, 252861.66635815732, 252949.37395827333, 253037.08155838933, 253124.78915829217, 253212.49675840818, 253300.20435852418, 253387.91195842702, 253475.61955854303, 253563.32715844587, 253651.03475856187, 253738.74235867788, 253826.44995858072, 253914.15755869672, 254001.86515881272, 254089.57275871557, 254177.28035883157, 254264.98795894757, 254352.69555885042, 254440.40315896642, 254528.11075908242, 254615.81835898527, 254703.52595910127, 254791.2335592173, 254878.94115912012, 254966.64875923612, 255054.35635913897, 255142.06395925497, 255229.771559371, 255317.47915927382, 255405.18675938982, 255492.89435950585, 255580.60195940867, 255668.3095595247, 255756.0171596407, 255843.72475954355, 255931.43235965955, 256019.13995977555, 256106.8475596784, 256194.5551597944, 256282.2627599104, 256369.97035981325, 256457.67795992925, 256545.3855598321, 256633.0931599481, 256720.8007600641, 256808.50835996695, 256896.21596008295, 256983.92356019895, 257071.6311601018, 257159.3387602178, 257247.0463603338, 257334.75396023665, 257422.46156035265, 257510.16916046865, 257597.8767603715, 257685.5843604875, 257773.2919606035, 257860.99956050635, 257948.70716062235, 258036.4147605252, 258124.1223606412, 258211.8299607572, 258299.53756066004, 258387.24516077604, 258474.95276089205, 258562.6603607949, 258650.3679609109, 258738.0755610269, 258825.78316092974, 258913.49076104574, 259001.19836116175, 259088.9059610646, 259176.6135611806, 259264.3211612966, 259352.02876119944, 259439.73636131544, 259527.44396143145, 259615.1515613343, 259702.8591614503, 259790.56676135314, 259878.27436146914, 259965.98196158514, 260053.689561488, 260141.397161604, 260229.10476172, 260316.81236162284, 260404.51996173884, 260492.22756185487, 260579.9351617577, 260667.64276187372, 260755.35036198972, 260843.05796189257, 260930.76556200857, 261018.47316212457, 261106.18076202742, 261193.88836214342, 261281.59596204627, 261369.30356216227, 261457.01116227827, 261544.71876218112, 261632.42636229712, 261720.13396241312, 261807.84156231597, 261895.54916243197, 261983.25676254797, 262070.96436245082, 262158.6719625668, 262246.3795626828, 262334.08716258564, 262421.79476270167, 262509.50236281764, 262597.2099627205, 262684.9175628365, 262772.62516273936, 262860.33276285534, 262948.04036297137, 263035.7479628742, 263123.4555629902, 263211.16316310625, 263298.87076300906, 263386.5783631251, 263474.28596324107, 263561.9935631439, 263649.7011632599, 263737.40876337595, 263825.11636327876, 263912.8239633948, 264000.53156351077, 264088.23916341364, 264175.9467635296, 264263.6543634325, 264351.36196354846, 264439.0695636645, 264526.7771635673, 264614.48476368334, 264702.1923637993, 264789.8999637022, 264877.60756381816, 264965.3151639342, 265053.022763837, 265140.73036395304, 265228.437964069, 265316.1455639719, 265403.85316408786, 265491.5607642039, 265579.2683641067, 265666.97596422274, 265754.68356412556, 265842.3911642416, 265930.09876435756, 266017.80636426044, 266105.5139643764, 266193.22156449244, 266280.92916439526, 266368.6367645113, 266456.34436462726, 266544.05196453014, 266631.7595646461, 266719.46716476214, 266807.17476466496, 266894.882364781, 266982.58996489696, 267070.29756479984, 267158.0051649158, 267245.71276503184, 267333.42036493466, 267421.1279650507, 267508.8355649535, 267596.54316506954, 267684.2507651855, 267771.9583650884, 267859.66596520436, 267947.3735653204, 268035.0811652232, 268122.78876533924, 268210.49636545527, 268298.2039653581, 268385.9115654741, 268473.6191655901, 268561.3267654929, 268649.03436560894, 268736.74196572497, 268824.4495656278, 268912.1571657438, 268999.86476564663, 269087.57236576267, 269175.27996587864, 269262.9875657815, 269350.6951658975, 269438.4027660135, 269526.11036591633, 269613.81796603237, 269701.52556614834, 269789.2331660512, 269876.9407661672, 269964.6483662832, 270052.35596618603, 270140.06356630207, 270227.77116641804, 270315.4787663209, 270403.1863664369, 270490.89396633976, 270578.60156645573, 270666.30916657177, 270754.0167664746, 270841.7243665906, 270929.4319667066, 271017.13956660946, 271104.84716672543, 271192.55476684147, 271280.2623667443, 271367.9699668603, 271455.6775669763, 271543.38516687916, 271631.09276699513, 271718.80036711117, 271806.507967014, 271894.21556713, 271981.92316703283, 272069.63076714886, 272157.33836726483, 272245.0459671677, 272332.7535672837, 272420.4611673997, 272508.16876730253, 272595.87636741856, 272683.58396753453, 272771.2915674374, 272858.9991675534, 272946.7067676694, 273034.41436757223, 273122.12196768826, 273209.82956780423, 273297.5371677071, 273385.2447678231, 273472.95236772596, 273560.65996784193, 273648.36756795796, 273736.0751678608, 273823.7827679768, 273911.49036809284, 273999.19796799566, 274086.9055681117, 274174.61316822766, 274262.32076813054, 274350.0283682465, 274437.73596836254, 274525.44356826536, 274613.1511683814, 274700.85876849736, 274788.56636840024, 274876.2739685162, 274963.98156863224, 275051.68916853506, 275139.3967686511, 275227.1043685539, 275314.81196866994, 275402.5195687859, 275490.2271686888, 275577.93476880476, 275665.6423689208, 275753.3499688236, 275841.05756893964, 275928.7651690556, 276016.4727689585, 276104.18036907446, 276191.8879691905, 276279.5955690933, 276367.30316920934, 276455.0107693253, 276542.7183692282, 276630.42596934416, 276718.13356924703, 276805.841169363, 276893.54876947904, 276981.25636938185, 277068.9639694979, 277156.67156961386, 277244.37916951673, 277332.0867696327, 277419.79436974874, 277507.50196965155, 277595.2095697676, 277682.91716988356, 277770.62476978643, 277858.3323699024, 277946.03997001844, 278033.74756992125, 278121.4551700373, 278209.1627699401, 278296.87037005613, 278384.5779701721, 278472.285570075, 278559.99317019095, 278647.700770307, 278735.4083702098, 278823.11597032583, 278910.82357044186, 278998.5311703447, 279086.2387704607, 279173.9463705767, 279261.6539704795, 279349.36157059553, 279437.06917071156, 279524.7767706144, 279612.4843707304, 279700.1919706332, 279787.89957074926, 279875.60717086523, 279963.3147707681, 280051.0223708841, 280138.7299710001, 280226.4375709029, 280314.14517101896, 280401.85277113493, 280489.5603710378, 280577.2679711538, 280664.9755712698, 280752.6831711726, 280840.39077128866, 280928.09837140463, 281015.8059713075, 281103.5135714235, 281191.22117132635, 281278.9287714423, 281366.63637155836, 281454.3439714612, 281542.0515715772, 281629.7591716932, 281717.46677159605, 281805.174371712, 281892.88197182806, 281980.5895717309, 282068.2971718469, 282156.0047719629, 282243.71237186575, 282331.4199719817, 282419.12757209776, 282506.8351720006, 282594.5427721166, 282682.2503720194, 282769.95797213545, 282857.6655722514, 282945.3731721543, 283033.0807722703, 283120.7883723863, 283208.4959722891, 283296.20357240515, 283383.9111725211, 283471.618772424, 283559.32637254, 283647.033972656, 283734.7415725588, 283822.44917267485, 283910.1567727909, 283997.8643726937, 284085.57197280973, 284173.2795729257, 284260.9871728285, 284348.69477294455, 284436.40237284737, 284524.1099729634, 284611.81757307943, 284699.52517298225, 284787.2327730983, 284874.94037321425, 284962.6479731171, 285050.3555732331, 285138.06317334913, 285225.77077325195, 285313.478373368, 285401.18597348395, 285488.8935733868, 285576.6011735028, 285664.30877361883, 285752.01637352165, 285839.7239736377, 285927.4315735405, 286015.1391736565, 286102.8467737725, 286190.5543736754, 286278.26197379135, 286365.9695739074, 286453.6771738102, 286541.3847739262, 286629.0923740422, 286716.7999739451, 286804.50757406105, 286892.2151741771, 286979.9227740799, 287067.6303741959, 287155.3379743119, 287243.0455742148, 287330.75317433075, 287418.4607742336, 287506.1683743496, 287593.8759744656, 287681.58357436844, 287769.2911744845, 287856.99877460045, 287944.7063745033, 288032.4139746193, 288120.1215747353, 288207.82917463814, 288295.5367747542, 288383.24437487015, 288470.951974773, 288558.659574889, 288646.367175005, 288734.07477490784, 288821.7823750239, 288909.4899749267, 288997.1975750427, 289084.9051751587, 289172.61277506157, 289260.32037517754, 289348.0279752936, 289435.7355751964, 289523.4431753124, 289611.15077542845, 289698.85837533127, 289786.5659754473, 289874.2735755633, 289961.98117546615, 290049.6887755821, 290137.39637569815, 290225.10397560097, 290312.811575717, 290400.5191756198, 290488.22677573585, 290575.9343758518, 290663.6419757547, 290751.34957587067, 290839.0571759867, 290926.7647758895, 291014.47237600555, 291102.1799761215, 291189.8875760244, 291277.59517614037, 291365.3027762564, 291453.0103761592, 291540.71797627525, 291628.4255763912, 291716.1331762941, 291803.84077641007, 291891.5483765261, 291979.2559764289, 292066.96357654495, 292154.67117644777, 292242.3787765638, 292330.08637667977, 292417.79397658264, 292505.5015766986, 292593.20917681465, 292680.91677671747, 292768.6243768335, 292856.33197694947, 292944.03957685234, 293031.7471769683, 293119.45477708435, 293207.16237698717, 293294.8699771032, 293382.57757721917, 293470.28517712204, 293557.992777238, 293645.7003771409, 293733.40797725687, 293821.1155773729, 293908.8231772757, 293996.53077739174, 294084.2383775077, 294171.9459774106, 294259.65357752657, 294347.3611776426, 294435.0687775454, 294522.77637766144, 294610.4839777775, 294698.1915776803, 294785.8991777963, 294873.6067779123, 294961.3143778151, 295049.02197793114, 295136.72957783396, 295224.43717795, 295312.144778066, 295399.85237796884, 295487.5599780849, 295575.26757820084, 295662.9751781037, 295750.6827782197, 295838.3903783357, 295926.09797823854, 296013.8055783546, 296101.51317847054, 296189.2207783734, 296276.9283784894, 296364.6359786054, 296452.34357850824, 296540.0511786243, 296627.7587785271, 296715.4663786431, 296803.1739787591, 296890.88157866197, 296978.58917877794, 297066.296778894, 297154.0043787968, 297241.7119789128, 297329.4195790288, 297417.12717893167, 297504.83477904764, 297592.5423791637, 297680.2499790665, 297767.9575791825, 297855.6651792985, 297943.37277920137, 298031.08037931734, 298118.7879792202, 298206.4955793362, 298294.2031794522, 298381.91077935504, 298469.61837947107, 298557.32597958704, 298645.0335794899, 298732.7411796059, 298820.4487797219, 298908.15637962474, 298995.86397974077, 299083.57157985674, 299171.2791797596, 299258.9867798756, 299346.6943799916, 299434.40197989444, 299522.10958001047, 299609.8171801265, 299697.5247800293, 299785.23238014535, 299872.93998004816, 299960.64758016414, 300048.35518028017, 300136.062780183, 300223.770380299, 300311.47798041505, 300399.18558031786, 300486.8931804339, 300574.60078054987, 300662.30838045274, 300750.0159805687, 300837.72358068475, 300925.43118058756, 301013.1387807036, 301100.84638081957, 301188.55398072244, 301276.2615808384, 301363.9691807413, 301451.67678085726, 301539.3843809733, 301627.0919808761, 301714.79958099214, 301802.5071811081, 301890.214781011, 301977.92238112696, 302065.629981243, 302153.3375811458, 302241.04518126184, 302328.7527813778, 302416.4603812807, 302504.16798139666, 302591.8755815127, 302679.5831814155, 302767.29078153154, 302854.99838143436, 302942.7059815504, 303030.41358166636, 303118.12118156924, 303205.8287816852, 303293.53638180124, 303381.24398170406, 303468.9515818201, 303556.65918193606, 303644.36678183894, 303732.0743819549, 303819.78198207094, 303907.48958197376, 303995.1971820898, 304082.90478220576, 304170.61238210864, 304258.3199822246, 304346.0275821275, 304433.73518224346, 304521.4427823595, 304609.1503822623, 304696.85798237834, 304784.5655824943, 304872.2731823972, 304959.98078251316, 305047.6883826292, 305135.395982532, 305223.10358264804, 305310.81118276407, 305398.5187826669, 305486.2263827829, 305573.9339828989, 305661.64158280176, 305749.34918291774, 305837.0567828206, 305924.7643829366, 306012.4719830526, 306100.17958295543, 306187.88718307146, 306275.59478318744, 306363.3023830903, 306451.0099832063, 306538.7175833223, 306626.42518322513, 306714.13278334116, 306801.84038345714, 306889.54798336, 306977.255583476, 307064.963183592, 307152.67078349483, 307240.37838361086, 307328.08598372684, 307415.7935836297, 307503.5011837457, 307591.20878364856, 307678.91638376453, 307766.62398388056, 307854.3315837834, 307942.0391838994, 308029.7467840154, 308117.45438391826, 308205.16198403423, 308292.86958415026, 308380.5771840531, 308468.2847841691, 308555.9923842851, 308643.69998418796, 308731.40758430393, 308819.11518441996, 308906.8227843228, 308994.5303844388, 309082.2379843416, 309169.94558445766, 309257.65318457363, 309345.3607844765, 309433.0683845925, 309520.7759847085, 309608.4835846113, 309696.19118472736, 309783.89878484333, 309871.6063847462, 309959.3139848622, 310047.0215849782, 310134.729184881, 310222.43678499706, 310310.1443851131, 310397.8519850159, 310485.55958513194, 310573.26718503475, 310660.9747851507, 310748.68238526676, 310836.3899851696, 310924.0975852856, 311011.80518540164, 311099.51278530445, 311187.2203854205, 311274.92798553646]
  out "Voltage out":cdb[](array[numeric])=[-8.966799e-06+0.004480194399i, -8.984636e-06+0.004479888585i, -9.010906e-06+0.0044800451i, -9.079564e-06+0.004480017873i, -9.182582e-06+0.004480175189i, -9.251079e-06+0.004480020904i, -9.271532e-06+0.004479934139i, -9.33771e-06+0.00447989056i, -9.35572e-06+0.00447976438i, -9.561729e-06+0.004479820275i, -9.510702e-06+0.00447971017i, -9.556176e-06+0.004479718025i, -9.577398e-06+0.0044795658i, -9.691955e-06+0.00447949231i, -9.785414e-06+0.004479379435i, -9.796209e-06+0.004479515312i, -9.968656e-06+0.004479403299i, -9.873545e-06+0.004479355815i, -9.89327e-06+0.004479407433i, -9.946952e-06+0.004479484271i, -1.0035937e-05+0.004479404113i, -1.0191257e-05+0.004479203683i, -1.0133458e-05+0.004479241971i, -1.022755e-05+0.004479310162i, -1.0300602e-05+0.004479179065i, -1.0258761e-05+0.004479266929i, -1.0351337e-05+0.004479232686i, -1.0455988e-05+0.00447890507i, -1.0527037e-05+0.004479132265i, -1.0533332e-05+0.004478851678i, -1.0639185e-05+0.004478790613i, -1.0718559e-05+0.004478693584i, -1.0588594e-05+0.00447879762i, -1.0624504e-05+0.004478777801i, -1.0737725e-05+0.004478679817i, -1.0882058e-05+0.004478805164i, -1.0887405e-05+0.004478860517i, -1.0863331e-05+0.004478660644i, -1.0921448e-05+0.004478578913i, -1.1024594e-05+0.004478676086i, -1.1010073e-05+0.004478666107i, -1.1132317e-05+0.00447865018i, -1.1164806e-05+0.004478432931i, -1.1099974e-05+0.004478601084i, -1.1289486e-05+0.004478483634i, -1.1329773e-05+0.004478385821i, -1.1347803e-05+0.00447837472i, -1.1367551e-05+0.004478360819i, -1.1445326e-05+0.004478491762i, -1.1538355e-05+0.004478438291i, -1.1557718e-05+0.004478248753i, -1.1579967e-05+0.004478355132i, -1.1649823e-05+0.004478261335i, -1.1665054e-05+0.004478086165i, -1.1727719e-05+0.004478207169i, -1.1741186e-05+0.004478162412i, -1.1704725e-05+0.004478099967i, -1.1822345e-05+0.00447804735i, -1.1954624e-05+0.00447783873i, -1.196149e-05+0.004478103923i, -1.1945245e-05+0.004478027913i, -1.2085918e-05+0.004477975742i, -1.1974872e-05+0.004477998265i, -1.2068495e-05+0.004478055522i, -1.2233779e-05+0.00447788034i, -1.2306594e-05+0.004477661354i, -1.2213147e-05+0.004477941359i, -1.2389775e-05+0.004477864421i, -1.2250403e-05+0.004477845157i, -1.2428922e-05+0.004477886381i, -1.2362574e-05+0.00447788297i, -1.2424584e-05+0.004477560771i, -1.2506777e-05+0.004477696213i, -1.2436457e-05+0.004477617037i, -1.2611628e-05+0.004477574614i, -1.2614173e-05+0.004477558984i, -1.2618078e-05+0.004477655541i, -1.2765231e-05+0.004477597958i, -1.272894e-05+0.004477582224i, -1.2845125e-05+0.004477662634i, -1.2769407e-05+0.004477669165i, -1.2941277e-05+0.004477641736i, -1.285681e-05+0.004477526994i, -1.294486e-05+0.004477580773i, -1.2981017e-05+0.00447746836i, -1.3092489e-05+0.004477401462i, -1.3048177e-05+0.004477297542i, -1.3092824e-05+0.004477331298i, -1.3182105e-05+0.004477225459i, -1.3278989e-05+0.004477025784i, -1.3219435e-05+0.004477184494i, -1.3245843e-05+0.004477184061i, -1.3348896e-05+0.004477053525i, -1.3289214e-05+0.004477049327i, -1.33461e-05+0.004476985879i, -1.3440788e-05+0.004476988409i, -1.3575e-05+0.004476908285i, -1.3462325e-05+0.004476901311i, -1.3477439e-05+0.004476890708i, -1.3645425e-05+0.004476890824i, -1.3643343e-05+0.004476834479i, -1.3646712e-05+0.004476646632i, -1.3661874e-05+0.004476885454i, -1.3723886e-05+0.004476786432i, -1.3750465e-05+0.004476689156i, -1.3793428e-05+0.004476853127i, -1.385432e-05+0.004476907943i, -1.3903518e-05+0.004476654874i, -1.388966e-05+0.00447676701i, -1.3959502e-05+0.004476741408i, -1.411256e-05+0.004476594512i, -1.4088119e-05+0.004476622063i, -1.421084e-05+0.004476707548i, -1.4106925e-05+0.004476773009i, -1.4218199e-05+0.004476607898i, -1.4248257e-05+0.004476735198i, -1.4219706e-05+0.004476769505i, -1.4253458e-05+0.004476672103i, -1.4259608e-05+0.004476642418i, -1.4335991e-05+0.004476531711i, -1.4389132e-05+0.004476436417i, -1.4438074e-05+0.004476564678i, -1.4504362e-05+0.004476544114i, -1.4530707e-05+0.004476817084i, -1.4548849e-05+0.004476595459i, -1.4623088e-05+0.004476379205i, -1.4688326e-05+0.004476605363i, -1.4620146e-05+0.004476381137i, -1.4712922e-05+0.004476414319i, -1.4737318e-05+0.004476510072i, -1.4857308e-05+0.004476374223i, -1.4888813e-05+0.004476403532i, -1.4978844e-05+0.004476112528i, -1.4982118e-05+0.004476083952i, -1.5003746e-05+0.004476178611i, -1.4976343e-05+0.004476050869i, -1.4994755e-05+0.004476210091i, -1.5035436e-05+0.004476068076i, -1.5036017e-05+0.004476126512i, -1.5144628e-05+0.004476003754i, -1.513503e-05+0.004476155491i, -1.527043e-05+0.004476068009i, -1.511558e-05+0.004476137474i, -1.5087651e-05+0.004476022086i, -1.5198804e-05+0.004475998477i, -1.5304956e-05+0.004476183912i, -1.5246673e-05+0.004476146961i, -1.5465755e-05+0.004476085254i, -1.5448016e-05+0.004475867801i, -1.5510073e-05+0.004475960245i, -1.550454e-05+0.004476021955i, -1.5544801e-05+0.004476015017i, -1.558873e-05+0.004476045373i, -1.5802435e-05+0.004475645889i, -1.5586001e-05+0.004475866405i, -1.5681936e-05+0.004475735127i, -1.5678313e-05+0.004475806187i, -1.5649693e-05+0.00447581095i, -1.5723564e-05+0.004475724077i, -1.5827848e-05+0.00447567906i, -1.5784133e-05+0.004475656383i, -1.5796623e-05+0.004475784804i, -1.5812578e-05+0.004475626221i, -1.5994355e-05+0.004475416081i, -1.5944695e-05+0.004475461179i, -1.5893443e-05+0.004475534923i, -1.5927087e-05+0.004475558662i, -1.6119688e-05+0.004475470845i, -1.6198032e-05+0.004475582758i, -1.6109918e-05+0.004475422804i, -1.6159895e-05+0.004475379358i, -1.6192038e-05+0.004475489509i, -1.6206041e-05+0.004475404296i, -1.6259613e-05+0.004475460002i, -1.6291134e-05+0.004475387053i, -1.6303983e-05+0.004475352766i, -1.631002e-05+0.004475279122i, -1.6398241e-05+0.004475393842i, -1.6429082e-05+0.004475357221i, -1.6434544e-05+0.004475268115i, -1.6496015e-05+0.00447545256i, -1.6577908e-05+0.004475307546i, -1.6569232e-05+0.004475241162i, -1.6582666e-05+0.004475366638i, -1.6598804e-05+0.004475363799i, -1.66588e-05+0.004475310566i, -1.664766e-05+0.004475344167i, -1.6812123e-05+0.004475469136i, -1.6763209e-05+0.004475413263i, -1.6892509e-05+0.004475447962i, -1.6827981e-05+0.004475463509i, -1.6866226e-05+0.004475378512i, -1.6919499e-05+0.00447514655i, -1.694114e-05+0.004475302027i, -1.7048399e-05+0.004475184521i, -1.7009461e-05+0.00447528221i, -1.7060535e-05+0.004475120439i, -1.7053169e-05+0.004475286249i, -1.711269e-05+0.004475289186i, -1.7131279e-05+0.004475223489i, -1.708768e-05+0.004475196976i, -1.73061e-05+0.00447533876i, -1.7229657e-05+0.0044752481i, -1.7248566e-05+0.004475296471i, -1.7291037e-05+0.004475202943i, -1.7343164e-05+0.004475257703i, -1.7392896e-05+0.004475017252i, -1.7315678e-05+0.004475145104i, -1.7462212e-05+0.004474959924i, -1.7426562e-05+0.004475069072i, -1.753547e-05+0.004475186781i, -1.7493809e-05+0.00447510138i, -1.7508857e-05+0.004475191213i, -1.7653292e-05+0.004475084618i, -1.7629526e-05+0.004474946593i, -1.7592512e-05+0.004474930572i, -1.769785e-05+0.004475094715i, -1.7760556e-05+0.004474995604i, -1.7712906e-05+0.00447501561i, -1.7701961e-05+0.004474957271i, -1.7896094e-05+0.004474978825i, -1.7789693e-05+0.004474960039i, -1.7928559e-05+0.004474981988i, -1.807916e-05+0.004474950102i, -1.800708e-05+0.004475078083i, -1.7949322e-05+0.004475061308i, -1.811568e-05+0.004475052416i, -1.8093777e-05+0.004474962887i, -1.8029858e-05+0.004475033208i, -1.8124002e-05+0.004475059465i, -1.8238525e-05+0.004474906465i, -1.8250836e-05+0.004475052508i, -1.8203265e-05+0.00447515322i, -1.8233916e-05+0.004475045308i, -1.8289562e-05+0.004475052641i, -1.8341615e-05+0.004474965813i, -1.8378223e-05+0.004475098414i, -1.8431962e-05+0.004475096557i, -1.8277172e-05+0.004475010462i, -1.8417278e-05+0.004474942418i, -1.8502614e-05+0.004474837152i, -1.8437738e-05+0.004474866317i, -1.8604934e-05+0.004475030524i, -1.8504162e-05+0.004475065364i, -1.863301e-05+0.004475012173i, -1.8570364e-05+0.004474784561i, -1.868682e-05+0.004474945907i, -1.8620012e-05+0.004474860404i, -1.874209e-05+0.004475000989i, -1.8771967e-05+0.004474934489i, -1.8892125e-05+0.004474948739i, -1.8841473e-05+0.004474975518i, -1.8905335e-05+0.004474997018i, -1.8945275e-05+0.004475169271i, -1.8888909e-05+0.004474967211i, -1.8919022e-05+0.004475238002i, -1.8989933e-05+0.004475056257i, -1.9147596e-05+0.004475022215i, -1.9118575e-05+0.004474999942i, -1.9100188e-05+0.004475072361i, -1.9137301e-05+0.004475060088i, -1.914666e-05+0.004475164336i, -1.9187967e-05+0.004475171582i, -1.9287356e-05+0.004475132573i, -1.9306032e-05+0.004475218181i, -1.9285996e-05+0.00447511068i, -1.9350183e-05+0.00447507056i, -1.939923e-05+0.004475370595i, -1.9377482e-05+0.004475299535i, -1.9512175e-05+0.004475178147i, -1.9469547e-05+0.004475254906i, -1.9467655e-05+0.004475307889i, -1.9572266e-05+0.004475295077i, -1.9478769e-05+0.004475449641i, -1.9608792e-05+0.004475438443i, -1.9582169e-05+0.004475505423i, -1.9687354e-05+0.004475399702i, -1.9641278e-05+0.004475533019i, -1.9721414e-05+0.004475583405i, -1.9694875e-05+0.004475575908i, -1.9805677e-05+0.004475854224i, -1.9735932e-05+0.004475646155i, -1.977325e-05+0.004475912323i, -1.9854581e-05+0.004476089206i, -1.9985651e-05+0.004476142668i, -1.9899279e-05+0.004476278465i, -2.0020488e-05+0.004476263182i, -1.9990365e-05+0.004476415007i, -2.0085058e-05+0.004476709643i, -2.0190022000000002e-05+0.004476712401i, -2.0160184e-05+0.004476841163i, -2.0181084e-05+0.004477160181i, -2.018836e-05+0.004477770818i, -2.0196067e-05+0.004477924582i, -2.0364584e-05+0.004478522246i, -2.0329473e-05+0.004479042421i, -2.0377874e-05+0.004479923494i, -2.0507384e-05+0.004481125672i, -2.0655584e-05+0.004482528763i, -2.0845924e-05+0.004485130532i, -2.1117077e-05+0.004489215754i, -2.2689813e-05+0.004499146947i, -3.4145946e-05+0.004535042099i, -6.2123794e-05+0.004384410573i, -2.4590016e-05+0.004446877975i, -2.1178842e-05+0.004456808002i, -2.1060116e-05+0.00446184279i, -2.0939261e-05+0.004464336486i, -2.0763597e-05+0.00446604474i, -2.084032e-05+0.004467203603i, -2.0936136e-05+0.004468180651i, -2.1171975e-05+0.004468883549i, -2.0770071e-05+0.004468571154i, -2.2099376e-05+0.004469281076i, -2.10174e-05+0.004468637298i, -2.0020737e-05+0.004470477664i, -2.0648848e-05+0.004470362884i, -2.1004877e-05+0.004470926211i, -2.068775e-05+0.004470811017i, -2.1022024e-05+0.004470635507i, -2.1290141e-05+0.004471176493i, -2.1192154e-05+0.00447117503i, -2.1118092e-05+0.004471256671i, -2.111728e-05+0.004471367678i, -2.1150959e-05+0.004471530513i, -2.1207481e-05+0.004471489514i, -2.1265926e-05+0.004471743271i, -2.1231556e-05+0.004471698513i, -2.1378171e-05+0.004471669251i, -2.129692e-05+0.004471895338i, -2.140575e-05+0.004471877735i, -2.1383617e-05+0.004471996748i, -2.1464277e-05+0.004471956439i, -2.1424916e-05+0.004472089104i, -2.1461442e-05+0.004471941938i, -2.1584059e-05+0.004471837199i, -2.1562452e-05+0.004471924426i, -2.155762e-05+0.004472255343i, -2.1654606e-05+0.004472167432i, -2.1675874e-05+0.004472262777i, -2.1688132e-05+0.004472200074i, -2.1716537e-05+0.00447222406i, -2.1759237e-05+0.004472371621i, -2.1770712e-05+0.004472124125i, -2.1817448e-05+0.004472237737i, -2.1769186e-05+0.004472109549i, -2.1909997e-05+0.004472236032i, -2.1896633e-05+0.004472252867i, -2.1936162e-05+0.004472423014i, -2.1922552e-05+0.004472553486i, -2.2058104e-05+0.004472294985i, -2.2059914e-05+0.00447241728i, -2.2012336e-05+0.004472413983i, -2.2071106e-05+0.0044724075i, -2.2065353e-05+0.004472258241i, -2.2092681e-05+0.004472209176i, -2.2200573e-05+0.004472356739i, -2.2181775e-05+0.004472273286i, -2.230587e-05+0.004472545638i, -2.2224389e-05+0.004472396746i, -2.2277544e-05+0.004472429987i, -2.2308277e-05+0.004472355699i, -2.2355035e-05+0.00447231818i, -2.2447392e-05+0.004472334146i, -2.2455462e-05+0.004472510702i, -2.2455507e-05+0.004472263852i, -2.2478387e-05+0.004472129021i, -2.2556452e-05+0.004472339594i, -2.2582579e-05+0.004472339938i, -2.2578635e-05+0.004472326205i, -2.2660834e-05+0.004472386089i, -2.2672291e-05+0.004472320682i, -2.2679559e-05+0.004472439568i, -2.2753178e-05+0.004472432642i, -2.2650349e-05+0.004472406204i, -2.2774551e-05+0.004472257618i, -2.2916413e-05+0.004472488221i, -2.2775171e-05+0.004472594219i, -2.2831891e-05+0.004472443496i, -2.2859754e-05+0.004472249993i, -2.2959541e-05+0.004472252193i, -2.293186e-05+0.004472173835i, -2.2968644e-05+0.004472141505i, -2.3094517e-05+0.004472315591i, -2.3072506e-05+0.004472169059i, -2.314754e-05+0.004472216032i, -2.3065225e-05+0.004472379187i, -2.3175129e-05+0.00447218538i, -2.3142233e-05+0.004472341175i, -2.3266136e-05+0.004472184325i, -2.3185275e-05+0.00447226508i, -2.3300552e-05+0.004471930514i, -2.3291525e-05+0.004472053386i, -2.3741864e-05+0.00447241301i, -2.3475038e-05+0.004471677513i, -2.2558367e-05+0.004472943133i, -2.2483949e-05+0.004471879148i, -2.29785e-05+0.004472453304i, -2.3500584e-05+0.004471831752i, -2.3450299e-05+0.00447219418i, -2.3490508e-05+0.004471927589i, -2.3608608e-05+0.004472397724i, -2.3517642e-05+0.004472219312i, -2.3604082e-05+0.004472251501i, -2.3697039e-05+0.004472272664i, -2.3730562e-05+0.00447226216i, -2.3748972e-05+0.004472148086i, -2.3677931e-05+0.004472264224i, -2.3743694e-05+0.004472147424i, -2.3800546e-05+0.004472126214i, -2.3881307e-05+0.004472175466i, -2.3915295e-05+0.004472063858i, -2.3904137e-05+0.004472119797i, -2.393692e-05+0.004472134393i, -2.4022192e-05+0.004472077855i, -2.4041529e-05+0.004472247421i, -2.3951148e-05+0.004471932234i, -2.4048308e-05+0.004472325605i, -2.4069952e-05+0.004472297843i, -2.4026815e-05+0.00447232341i, -2.4118341e-05+0.004472291651i, -2.4126911e-05+0.004472054361i, -2.4230641e-05+0.004472082662i, -2.430981e-05+0.004471890486i, -2.4226504e-05+0.004472253711i, -2.434609e-05+0.004472117329i, -2.4325048e-05+0.004472192234i, -2.4410852e-05+0.004472109834i, -2.4465402e-05+0.0044721209i, -2.4475434e-05+0.004472291019i, -2.4525389e-05+0.004472144181i, -2.4547854e-05+0.004472066964i, -2.4542919e-05+0.004471968705i, -2.4544494e-05+0.004471886419i, -2.4581e-05+0.004471931502i, -2.4708468e-05+0.004471945356i, -2.4651088e-05+0.004471959081i, -2.4675236e-05+0.004471978859i, -2.4816005e-05+0.004472178148i, -2.4776549e-05+0.004472153548i, -2.4886153e-05+0.004472107633i, -2.4850595e-05+0.004472064885i, -2.4822075e-05+0.004472049182i, -2.4891687e-05+0.004471995146i, -2.5005276e-05+0.004472029012i, -2.4928739e-05+0.00447202595i, -2.5172755e-05+0.004471794983i, -2.5069656e-05+0.004472094332i, -2.5107844e-05+0.004471905374i, -2.5048629e-05+0.004471901293i, -2.5187385e-05+0.004471953953i, -2.5135865e-05+0.004471988175i, -2.5244765e-05+0.004471861634i, -2.5197143e-05+0.004472161606i, -2.5245603e-05+0.004472113463i, -2.5297308e-05+0.004472071729i, -2.5375279e-05+0.004472037914i, -2.5294327e-05+0.004471871463i, -2.5362854e-05+0.004471886307i, -2.5388537e-05+0.004472015309i, -2.5436577e-05+0.004471949446i, -2.5565792e-05+0.004471910093i, -2.5527629e-05+0.004471849101i, -2.5407953e-05+0.004471747734i, -2.54689e-05+0.004472092017i, -2.5627371e-05+0.004472107012i, -2.5646483e-05+0.00447214557i, -2.5674245e-05+0.004471972862i, -2.5676776e-05+0.004472025633i, -2.5784526e-05+0.004471863523i, -2.568849e-05+0.004472034829i, -2.5745752e-05+0.004472052877i, -2.5847626e-05+0.004471914616i, -2.5923214e-05+0.004471969856i, -2.5954551e-05+0.004472145382i, -2.5834241e-05+0.004472064866i, -2.5938262e-05+0.004471942751i, -2.5993528e-05+0.004471893649i, -2.6046858e-05+0.004472021589i, -2.6026813e-05+0.004471831357i, -2.6169629e-05+0.00447180291i, -2.6077981e-05+0.004471922804i, -2.6123557e-05+0.004471916924i, -2.6150624e-05+0.004471971378i, -2.6218429e-05+0.004472089859i, -2.6148556e-05+0.0044718811i, -2.6183415e-05+0.00447184277i, -2.6322869e-05+0.004471796509i, -2.6345362e-05+0.004471868202i, -2.6318073e-05+0.004472026995i, -2.6402743e-05+0.004471959557i, -2.6404646e-05+0.004471813954i, -2.6415092e-05+0.004471973102i, -2.6391569e-05+0.004472046961i, -2.6505564e-05+0.004471967263i, -2.6544806e-05+0.004471826949i, -2.6588381e-05+0.004471902196i, -2.6561992e-05+0.004471876851i, -2.6664554e-05+0.004471962339i, -2.6679799e-05+0.004471661813i, -2.6669842e-05+0.004471813834i, -2.6685902e-05+0.004471537666i, -2.674616e-05+0.004471810462i, -2.6868162e-05+0.004472024257i, -2.6807177e-05+0.004471847046i, -2.6844461e-05+0.004471728285i, -2.6812535e-05+0.004471672639i, -2.6949554e-05+0.004471541679i, -2.7059436e-05+0.004471534952i, -2.696911e-05+0.004471766674i, -2.699557e-05+0.004471733188i, -2.7103951e-05+0.004471850377i, -2.7065971e-05+0.00447201511i, -2.7150372e-05+0.004471879663i, -2.7131941e-05+0.004471864483i, -2.7245157e-05+0.004472034176i, -2.7235776e-05+0.004471939743i, -2.7184489e-05+0.004471804253i, -2.7235257e-05+0.004471870091i, -2.7309956e-05+0.004471906492i, -2.7333829e-05+0.004471830209i, -2.7352459e-05+0.004471979905i, -2.7394444e-05+0.004472093382i, -2.7451874e-05+0.004471826193i, -2.7483767e-05+0.004471755442i, -2.7492736e-05+0.004471775011i, -2.7625317e-05+0.004471841524i, -2.7495035e-05+0.004471708273i, -2.7642866e-05+0.004471825456i, -2.7555315e-05+0.00447182179i, -2.7682349e-05+0.004471637578i, -2.769072e-05+0.004471694077i, -2.7715923e-05+0.00447158716i, -2.774418e-05+0.004471556661i, -2.7783751e-05+0.004471532939i, -2.7803156e-05+0.004471519976i, -2.7863084e-05+0.004471763614i, -2.7903683e-05+0.004471869166i, -2.791698e-05+0.00447174035i, -2.7991047e-05+0.004471661641i, -2.7956086e-05+0.004471629787i, -2.7951055e-05+0.00447176581i, -2.8071256e-05+0.00447177617i, -2.8011746e-05+0.004471842355i, -2.8112451e-05+0.004471651309i, -2.7991603e-05+0.004471462567i, -2.8110133e-05+0.004471610785i, -2.8211998e-05+0.004471662869i, -2.8158828e-05+0.004471687146i, -2.8215274e-05+0.004471620592i, -2.8264478e-05+0.004471501111i, -2.8352539e-05+0.004471362605i, -2.8295759e-05+0.004471581705i, -2.8419792e-05+0.004471479441i, -2.8460227e-05+0.004471471158i, -2.8382726e-05+0.004471461318i, -2.8457222e-05+0.004471599945i, -2.8457966e-05+0.004471509449i, -2.8614231e-05+0.004471527115i, -2.854441e-05+0.004471540627i, -2.8579647e-05+0.004471520157i, -2.8632579e-05+0.004471614532i, -2.8701559e-05+0.004471392368i, -2.863819e-05+0.004471404595i, -2.8724902e-05+0.004471346991i, -2.8693372e-05+0.004471357526i, -2.8807851e-05+0.004471441235i, -2.8821913e-05+0.004471295172i, -2.879602e-05+0.004471429396i, -2.8853722e-05+0.004471369319i, -2.8900597e-05+0.004471420847i, -2.8923643e-05+0.004471464019i, -2.8980996e-05+0.00447133847i, -2.8960391e-05+0.004471546576i, -2.8980999e-05+0.004471530955i, -2.9029681e-05+0.004471631753i, -2.9011222e-05+0.004471624115i, -2.9090919e-05+0.004471369307i, -2.9205897e-05+0.004471525174i, -2.9165118e-05+0.00447156918i, -2.9077601e-05+0.00447136773i, -2.9266066e-05+0.004471284272i, -2.9276031e-05+0.004471512032i, -2.920511e-05+0.004471399191i, -2.9352302e-05+0.004471576085i, -2.9376646e-05+0.004471547758i, -2.9476219e-05+0.004471391442i, -2.9437859e-05+0.004471447874i, -2.9468754e-05+0.004471478333i, -2.9552563e-05+0.004471242877i, -2.9509274e-05+0.004471370567i, -2.9576326e-05+0.004471289244i, -2.9654548e-05+0.004471152724i, -2.962252e-05+0.004471309716i, -2.9637967e-05+0.004471229124i, -2.9740468e-05+0.00447118749i, -2.9715718e-05+0.004471215574i, -2.9737883e-05+0.004471304635i, -2.9896864e-05+0.004471159582i, -2.9788222e-05+0.004471157203i, -2.9857197e-05+0.004471351641i, -2.9889227e-05+0.004471234701i, -2.9840478e-05+0.004471396564i, -2.9987208e-05+0.004471299664i, -2.9888544e-05+0.004471337104i, -2.9965114e-05+0.004471212286i, -2.999055e-05+0.004471437346i, -3.0026859e-05+0.004471421707i, -3.0113331e-05+0.004471410464i, -3.0107743e-05+0.00447143013i, -3.0161731e-05+0.004471353188i, -3.0156348e-05+0.004471359892i, -3.0242611e-05+0.004471467192i, -3.0183377e-05+0.004471471452i, -3.0354137e-05+0.00447127453i, -3.0328221e-05+0.004471242725i, -3.0281706e-05+0.004471315415i, -3.0326463e-05+0.004471275448i, -3.0495283e-05+0.004471181595i, -3.0429458e-05+0.004471329907i, -3.053843e-05+0.004471258044i, -3.0501102e-05+0.004471186854i, -3.0500457e-05+0.004471292269i, -3.0604079e-05+0.004471281866i, -3.0664558e-05+0.004471167677i, -3.0615693e-05+0.004471043023i, -3.0633697e-05+0.004470987859i, -3.053516e-05+0.004471073119i, -3.0835595e-05+0.004470842072i, -3.0940505e-05+0.004471089785i, -3.0687952e-05+0.004470996575i, -3.0858557e-05+0.004471117616i, -3.0886476e-05+0.004471026142i, -3.091725e-05+0.004470963287i, -3.0870617e-05+0.004471171589i, -3.1006078e-05+0.004471295126i, -3.1004256e-05+0.004471271022i, -3.0946356e-05+0.004471279053i, -3.1048755e-05+0.004471118696i, -3.1102547e-05+0.004471238306i, -3.0966396e-05+0.004471075714i, -3.110856e-05+0.004471065951i, -3.1237118e-05+0.004471080966i, -3.1226726e-05+0.004470993745i, -3.1280631e-05+0.004471171168i, -3.1269247e-05+0.004470990875i, -3.1289013e-05+0.004471178432i, -3.1359966e-05+0.004471388478i, -3.1349541e-05+0.004471278514i, -3.1362414e-05+0.004471105569i, -3.1418881e-05+0.004471123723i, -3.1440978e-05+0.004471204131i, -3.146433e-05+0.004471084521i, -3.1542116e-05+0.004471115736i, -3.1411114e-05+0.004471219718i, -3.1598157e-05+0.004471105976i, -3.1642527e-05+0.004471072289i, -3.1604255e-05+0.004471162657i, -3.1608125e-05+0.004471198345i, -3.1675961e-05+0.004471138183i, -3.1774554e-05+0.004471237726i, -3.1689409e-05+0.00447130541i, -3.1819295e-05+0.004471204318i, -3.1795275e-05+0.004471088653i, -3.1924919e-05+0.00447116981i, -3.1898088e-05+0.004471146383i, -3.2010766e-05+0.004471164444i, -3.2004974e-05+0.004470963046i, -3.2024987e-05+0.004470925805i, -3.2057099e-05+0.004471094826i, -3.1991305e-05+0.004471003565i, -3.2176823e-05+0.004471239852i, -3.2063398e-05+0.004471242401i, -3.2247245e-05+0.004471255932i, -3.2171436e-05+0.004471124934i, -3.2192983e-05+0.004471254899i, -3.2252076e-05+0.004471335403i, -3.2310675e-05+0.004471294579i, -3.2337841e-05+0.004471193582i, -3.2419415e-05+0.004471156556i, -3.242824e-05+0.00447118364i, -3.2456498e-05+0.004471172901i, -3.2461039e-05+0.004471184544i, -3.2568401e-05+0.0044711665i, -3.254846e-05+0.00447102299i, -3.2586166e-05+0.004471254924i, -3.2617717e-05+0.004471168299i, -3.272359e-05+0.004471277844i, -3.2633766e-05+0.004471086114i, -3.2664581e-05+0.004471004611i, -3.2700495e-05+0.004471296507i, -3.2711594e-05+0.004471209133i, -3.2738896e-05+0.004471009315i, -3.2849839e-05+0.004470990083i, -3.2861031e-05+0.004470802484i, -3.2882069e-05+0.004470797911i, -3.2840325e-05+0.004470883005i, -3.2898601e-05+0.004470997273i, -3.2852805e-05+0.004470958718i, -3.2971096e-05+0.004470858177i, -3.3038371e-05+0.004470983009i, -3.3007683e-05+0.004470899604i, -3.2982894e-05+0.004470998231i, -3.3105088e-05+0.004471019076i, -3.3119641e-05+0.004471087562i, -3.3170019e-05+0.004470870058i, -3.3212498e-05+0.004470785404i, -3.3154644e-05+0.004470958184i, -3.3288654e-05+0.004471046062i, -3.3296436e-05+0.004470645191i, -3.3331052e-05+0.004470793622i, -3.3249908e-05+0.004470773354i, -3.3306857e-05+0.004470893754i, -3.3394525e-05+0.004470830559i, -3.3469231e-05+0.004470991151i, -3.3422822e-05+0.004470654975i, -3.3424296e-05+0.004470786585i, -3.3519699e-05+0.004470759893i, -3.3589666e-05+0.00447067064i, -3.3624815e-05+0.004470628063i, -3.3596019e-05+0.004470511026i, -3.3664202e-05+0.004470525555i, -3.371442e-05+0.004470578269i, -3.371245e-05+0.004470518238i, -3.3713146e-05+0.004470579168i, -3.3883065e-05+0.004470679526i, -3.378525e-05+0.00447053188i, -3.3817069e-05+0.004470523642i, -3.3859804e-05+0.004470675136i, -3.3894589e-05+0.00447066633i, -3.3973916e-05+0.004470643217i, -3.4013292e-05+0.004470732061i, -3.4005709e-05+0.004470769019i, -3.4093489e-05+0.004470720717i, -3.4020538e-05+0.00447055694i, -3.408235e-05+0.004470701624i, -3.4170322e-05+0.004470820293i, -3.4283285e-05+0.004470688767i, -3.4151612e-05+0.004470744156i, -3.4246819e-05+0.004470546659i, -3.4237747e-05+0.004470657576i, -3.4363473e-05+0.004470729697i, -3.4302252e-05+0.004470591007i, -3.4326008e-05+0.004470702635i, -3.439949e-05+0.004470525013i, -3.4398464e-05+0.004470626502i, -3.4454261e-05+0.00447064382i, -3.4566872e-05+0.004470737972i, -3.4532865e-05+0.004470486532i, -3.452964e-05+0.004470368668i, -3.4620052e-05+0.004470580421i, -3.4636336e-05+0.004470567396i, -3.473838e-05+0.004470557532i, -3.4713676e-05+0.004470553997i, -3.4734312e-05+0.004470724405i, -3.4818289e-05+0.004470594894i, -3.4669513e-05+0.004470701544i, -3.4884692e-05+0.004470397115i, -3.4767631e-05+0.004470478132i, -3.4855324e-05+0.004470425494i, -3.4927621e-05+0.004470218242i, -3.4935265e-05+0.004470218406i, -3.4889275e-05+0.004470438581i, -3.5049435e-05+0.004470337343i, -3.5031333e-05+0.004470309276i, -3.4979353e-05+0.00447030087i, -3.4990122e-05+0.004470308155i, -3.5086792e-05+0.004470207892i, -3.5231144e-05+0.004470357214i, -3.5138536e-05+0.004470140601i, -3.5194119e-05+0.004470192987i, -3.5194023e-05+0.004470142623i, -3.5236035e-05+0.004470224772i, -3.5285809e-05+0.004470235822i, -3.5296946e-05+0.004470172099i, -3.5315284e-05+0.00447011956i, -3.5504452e-05+0.004470143719i, -3.5427786e-05+0.004470248065i, -3.5416655e-05+0.004470066989i, -3.5415566e-05+0.004470120975i, -3.5508026e-05+0.004470099424i, -3.5567954e-05+0.004470016735i, -3.56086e-05+0.004470177919i, -3.5506246e-05+0.004470215258i, -3.5655221e-05+0.00447024995i, -3.5668004e-05+0.004470291663i, -3.5701787e-05+0.00447045686i, -3.5797075e-05+0.004470305764i, -3.5742616e-05+0.004470140113i, -3.5793088e-05+0.004470406103i, -3.5778082e-05+0.00447015162i, -3.5831172e-05+0.004470301829i, -3.5883695e-05+0.004470224001i, -3.5939143e-05+0.00447028329i, -3.5851994e-05+0.004470170958i, -3.6003124e-05+0.004470266632i, -3.6056769e-05+0.004470178042i, -3.6008666e-05+0.004470083613i, -3.6111217e-05+0.004470139644i, -3.6133351e-05+0.00447005326i, -3.6224007e-05+0.004470258806i, -3.6160631e-05+0.004470045311i, -3.6180215e-05+0.004470082362i, -3.6213835e-05+0.004470113082i, -3.6259945e-05+0.004470063877i, -3.6261165e-05+0.004469987422i, -3.6301781e-05+0.004470152018i, -3.6342719e-05+0.004470081548i, -3.6397197e-05+0.004470044511i, -3.6483266e-05+0.004470055136i, -3.6495886e-05+0.004470003613i, -3.6441548e-05+0.004470293804i, -3.6489669e-05+0.00447025668i, -3.6516266e-05+0.004470254873i, -3.6564905e-05+0.004470185947i, -3.6689046e-05+0.004470523831i, -3.6649416e-05+0.004470372359i, -3.6642126e-05+0.004470264333i, -3.6678627e-05+0.004470245417i, -3.6778083e-05+0.004470268756i, -3.6763155e-05+0.004470301427i, -3.6804318e-05+0.004470090284i, -3.6815876e-05+0.004470147937i, -3.6861366e-05+0.004470207277i, -3.6926013e-05+0.004469991582i, -3.6996815e-05+0.004470165619i, -3.6948545e-05+0.004470067834i, -3.7038288e-05+0.004470153635i, -3.7045345e-05+0.004470139397i, -3.6978368e-05+0.004470193136i, -3.7137076e-05+0.00447009723i, -3.7171905e-05+0.004470158139i, -3.7168881e-05+0.004470154787i, -3.7195271e-05+0.004470127629i, -3.7268175e-05+0.004469978096i, -3.71972e-05+0.004470192074i, -3.7241761e-05+0.004470259107i, -3.7337845e-05+0.004470058031i, -3.7292362e-05+0.004470004714i, -3.7431963e-05+0.004470140762i, -3.7357555e-05+0.004470162567i, -3.7444038e-05+0.004470021749i, -3.7471901e-05+0.00447001743i, -3.7491176e-05+0.004470137894i, -3.746873e-05+0.004470131099i, -3.7540635e-05+0.004470117009i, -3.7581748e-05+0.004470105671i, -3.7613827e-05+0.004469979221i, -3.7653632e-05+0.00447006992i, -3.7615836e-05+0.004470095108i, -3.7702148e-05+0.004469904011i, -3.7838997e-05+0.004470066357i, -3.7791064e-05+0.004469833437i, -3.7713944e-05+0.004470039939i, -3.7752486e-05+0.004470084995i, -3.7882333e-05+0.004470092973i, -3.7866102e-05+0.004470003118i, -3.7907984e-05+0.004469840265i, -3.794834e-05+0.00447006313i, -3.7998004e-05+0.004469946675i, -3.8033399e-05+0.00447001287i, -3.8049083e-05+0.004469942833i, -3.8114494e-05+0.00446993863i, -3.8095097e-05+0.004469826291i, -3.8087222e-05+0.004470000371i, -3.8148694e-05+0.004469777878i, -3.8223896e-05+0.004469889789i, -3.8229447e-05+0.004469769683i, -3.8283885e-05+0.004470042285i, -3.8308813e-05+0.004469855215i, -3.8217602e-05+0.004469761178i, -3.8422964e-05+0.004469750103i, -3.8399434e-05+0.004469864743i, -3.8463335e-05+0.004469829785i, -3.8444865e-05+0.004469746543i, -3.8495097e-05+0.004470022767i, -3.84659e-05+0.004469963154i, -3.8470827e-05+0.004469880373i, -3.853806e-05+0.004469678262i, -3.8659514e-05+0.00446988938i, -3.8633829e-05+0.004469930462i, -3.867269e-05+0.004470019134i, -3.8733809e-05+0.004469949928i, -3.8730247e-05+0.004469881063i, -3.8731173e-05+0.004470007609i, -3.8823674e-05+0.004470111667i, -3.8871871e-05+0.004469921052i, -3.8921067e-05+0.004469926739i, -3.8905054e-05+0.004469875285i, -3.9026286e-05+0.004469944754i, -3.9022298e-05+0.004470091295i, -3.8870239e-05+0.004469925632i, -3.8931649e-05+0.004469987725i, -3.9056611e-05+0.004469914194i, -3.9082399e-05+0.004469892531i, -3.9160828e-05+0.004469997601i, -3.9144305e-05+0.004469967212i, -3.9210854e-05+0.004469959856i, -3.9206875e-05+0.00446987181i, -3.9221634e-05+0.004469896355i, -3.9275469e-05+0.004470099841i, -3.9309553e-05+0.004469629144i, -3.9353609e-05+0.004470116964i, -3.9415642e-05+0.004469839351i, -3.9399283e-05+0.004469891207i, -3.9409776e-05+0.004469992437i, -3.952659e-05+0.004469821309i, -3.9534812e-05+0.004469849231i, -3.9439883e-05+0.004469753504i, -3.9526736e-05+0.004470003725i, -3.9640837e-05+0.004469881917i, -3.9655835e-05+0.004469951485i, -3.969084e-05+0.00446977013i, -3.9729002e-05+0.00446974995i, -3.977056e-05+0.004469706244i, -3.9760723e-05+0.004470020943i, -3.9759757e-05+0.004469859598i, -3.9897142e-05+0.004469644046i, -3.9754223e-05+0.004469711573i, -3.9882045e-05+0.004469659412i, -3.9944755e-05+0.004469726451i, -3.9916189e-05+0.004469553883i, -3.9924654e-05+0.004469794295i, -4.0003819e-05+0.004469797419i, -4.0118801e-05+0.004469620679i, -4.0082017e-05+0.004469699832i, -4.0085787e-05+0.004469562149i, -4.004295e-05+0.004469575469i, -4.0161531e-05+0.004469624954i, -4.0242684e-05+0.004469537131i, -4.0159429e-05+0.004469720854i, -4.024577e-05+0.00446963343i, -4.0242622e-05+0.004469458537i, -4.0238938e-05+0.004469403146i, -4.0349029e-05+0.004469533322i, -4.0415418e-05+0.004469409618i, -4.0409758e-05+0.004469583694i, -4.044823e-05+0.004469550439i, -4.0505531e-05+0.004469593856i, -4.0445546e-05+0.004469704069i, -4.0460023e-05+0.004469683425i, -4.0571005e-05+0.004469574333i, -4.0651105e-05+0.004469657938i, -4.0570196e-05+0.004469751463i, -4.0621936e-05+0.004469771092i, -4.0699666e-05+0.004469565831i, -4.0773125e-05+0.004469629136i, -4.0793639e-05+0.004469647705i, -4.0759146e-05+0.004469644861i, -4.0932317e-05+0.004469621254i, -4.0890082e-05+0.004469724812i, -4.0766082e-05+0.004469680259i, -4.0902676e-05+0.004469623264i, -4.091319e-05+0.004469636466i, -4.0968008e-05+0.00446972175i, -4.1046956e-05+0.004469633545i, -4.102214e-05+0.004469466203i, -4.1014206e-05+0.004469727448i, -4.1171605e-05+0.004469459017i, -4.1173708e-05+0.004469692229i, -4.1180055e-05+0.004469710889i, -4.1126313e-05+0.004469555496i, -4.1219499e-05+0.004469724876i, -4.1233259e-05+0.004469686937i, -4.1337319e-05+0.004469654319i, -4.1315789e-05+0.00446961637i, -4.1441137e-05+0.004469623012i, -4.1386869e-05+0.004469583569i, -4.1418793e-05+0.00446970418i, -4.1472813e-05+0.004469463716i, -4.1481674e-05+0.004469453706i, -4.1487876e-05+0.004469654301i, -4.1632132e-05+0.004469528741i, -4.1635603e-05+0.004469387087i, -4.1597418e-05+0.004469540633i, -4.154688e-05+0.004469498663i, -4.164993e-05+0.004469332895i, -4.1668241e-05+0.004469412068i, -4.1711737e-05+0.004469575542i, -4.1715309e-05+0.004469558011i, -4.1759061e-05+0.004469441181i, -4.183418e-05+0.004469505244i, -4.1861072e-05+0.004469510769i, -4.1935358e-05+0.004469430939i, -4.1854602e-05+0.00446944177i, -4.1911967e-05+0.00446946156i, -4.1930398e-05+0.004469349243i, -4.2014295e-05+0.004469369586i, -4.1994677e-05+0.004469236537i, -4.2015397e-05+0.004469287207i, -4.2012662e-05+0.00446914879i, -4.2013186e-05+0.004469499539i, -4.2155071e-05+0.004469342707i, -4.216643e-05+0.004469320202i, -4.219605e-05+0.00446925924i, -4.2200556e-05+0.004469193412i, -4.2337236e-05+0.004469270877i, -4.2331404e-05+0.004469309566i, -4.2335563e-05+0.004469364831i, -4.2366335e-05+0.004469347004i, -4.2356141e-05+0.00446926802i, -4.2424348e-05+0.004469164549i, -4.2427681e-05+0.00446927655i, -4.2472072e-05+0.004469187336i, -4.2549613e-05+0.004469158883i, -4.2550368e-05+0.004469219547i, -4.2630944e-05+0.004469221369i, -4.2504063e-05+0.004469287348i, -4.2638954e-05+0.004469309927i, -4.2629669e-05+0.004469316596i, -4.2711776e-05+0.004469267029i, -4.2702874e-05+0.004469286566i, -4.2785629e-05+0.004469224052i, -4.2782081e-05+0.004469385642i, -4.2762915e-05+0.004469110607i, -4.2859927e-05+0.004469205926i, -4.2820708e-05+0.004469082363i, -4.2912256e-05+0.004469016107i, -4.2907665e-05+0.004469175929i, -4.2942868e-05+0.004469049832i, -4.3041659e-05+0.004469085702i, -4.3084281e-05+0.004469134951i, -4.3139323e-05+0.00446893499i, -4.3077779e-05+0.004468921156i, -4.3158184e-05+0.004469015524i, -4.3160517e-05+0.004469120593i, -4.3310844e-05+0.004469214173i, -4.3298961e-05+0.004469091673i, -4.3304708e-05+0.004469220626i, -4.3227349e-05+0.004469296576i, -4.3274327e-05+0.004469174566i, -4.3308641e-05+0.004469125545i, -4.3420899e-05+0.004469170133i, -4.3437976e-05+0.004469227703i, -4.3457789e-05+0.004469275003i, -4.3509149e-05+0.004469213856i, -4.3547506e-05+0.004469227035i, -4.3594701e-05+0.004469262644i, -4.3613498e-05+0.004469307539i, -4.360674e-05+0.004469243737i, -4.3700705e-05+0.004469149524i, -4.370535e-05+0.004469289922i, -4.3785168e-05+0.004469301691i, -4.3777373e-05+0.004469208359i, -4.3859706e-05+0.004469118256i, -4.3804286e-05+0.004468990116i, -4.3875013e-05+0.004468918435i, -4.3873852e-05+0.004469057092i, -4.3889801e-05+0.004469012317i, -4.3983287e-05+0.004469139149i, -4.3911913e-05+0.004469186543i, -4.3992114e-05+0.004469040559i, -4.3955592e-05+0.004468947076i, -4.4015722e-05+0.004469195284i, -4.4097894e-05+0.004469430567i, -4.4187219e-05+0.004469096987i, -4.4174664e-05+0.004469241015i, -4.4334225e-05+0.00446907626i, -4.4234313e-05+0.004469037928i, -4.4214052e-05+0.004469048315i, -4.4337899e-05+0.004469204745i, -4.4311127e-05+0.004469069869i, -4.4314834e-05+0.004469174766i, -4.4396725e-05+0.004469139887i, -4.4410219e-05+0.004468992847i, -4.4350344e-05+0.004468974732i, -4.4437038e-05+0.004469130957i, -4.4514085e-05+0.00446898926i, -4.4511731e-05+0.004469210499i, -4.4573005e-05+0.004469114416i, -4.4538203e-05+0.004469204907i, -4.4635918e-05+0.004469111472i, -4.4626026e-05+0.004469002487i, -4.4681472e-05+0.00446912072i, -4.4679612e-05+0.004468988771i, -4.4750557e-05+0.004468967541i, -4.4779613e-05+0.00446905068i, -4.4772884e-05+0.004469177559i, -4.4824058e-05+0.004468963326i, -4.488591e-05+0.004469095876i, -4.4803021e-05+0.004469055697i, -4.4965363e-05+0.004469125174i, -4.4952579e-05+0.004468902073i, -4.4882163e-05+0.004469003088i, -4.5010837e-05+0.004468985446i, -4.5058275e-05+0.004468907182i, -4.5013256e-05+0.00446889241i, -4.5133582e-05+0.004468952579i, -4.5191844e-05+0.004469027605i, -4.5177363e-05+0.004468806426i, -4.5189977e-05+0.004468884012i, -4.5204376e-05+0.004468748315i, -4.5218781e-05+0.004468935414i, -4.5355595e-05+0.004468803738i, -4.5309659e-05+0.004468764265i, -4.5377352e-05+0.004468703833i, -4.5409716e-05+0.004468748423i, -4.543204e-05+0.004468651892i, -4.5466713e-05+0.004468600619i, -4.5482411e-05+0.004468689402i, -4.5455625e-05+0.004468782975i, -4.55458e-05+0.004469008371i, -4.5598851e-05+0.004468777964i, -4.5577055e-05+0.004468928783i, -4.5566465e-05+0.004468994114i, -4.5645475e-05+0.004468840345i, -4.5676748e-05+0.004468728013i, -4.5783476e-05+0.004468909664i, -4.5831839e-05+0.004468952722i, -4.5836508e-05+0.004469089209i, -4.5838706e-05+0.004468814353i, -4.5872007e-05+0.0044688145i, -4.5884317e-05+0.004468619734i, -4.5966019e-05+0.004468740252i, -4.5935042e-05+0.004468766185i, -4.5988139e-05+0.004468668996i, -4.6005961e-05+0.004468673434i, -4.6031318e-05+0.004468675278i, -4.6055014e-05+0.004468611859i, -4.6107296e-05+0.004468618444i, -4.6153816e-05+0.004468595677i, -4.6154023e-05+0.004468809409i, -4.6143541e-05+0.004468587583i, -4.6217072e-05+0.004468674035i, -4.6331319e-05+0.004468579143i, -4.6328213e-05+0.004468836587i, -4.6318327e-05+0.004468797446i, -4.6353639e-05+0.004468850221i, -4.6450002e-05+0.004468903027i, -4.6397451e-05+0.004468531729i, -4.6416068e-05+0.004468510366i, -4.6459249e-05+0.004468516525i, -4.6502559e-05+0.004468593129i, -4.6612288e-05+0.004468486079i, -4.6623507e-05+0.004468694796i, -4.6631311e-05+0.004468636534i, -4.6683535e-05+0.00446868174i, -4.6655223e-05+0.004468635619i, -4.6750401e-05+0.004468326446i, -4.6670095e-05+0.004468619727i, -4.6706897e-05+0.004468373982i, -4.6742214e-05+0.004468424485i, -4.6899142e-05+0.004468454259i, -4.6884369e-05+0.004468469523i, -4.6984161e-05+0.004468707998i, -4.6925518e-05+0.004468496262i, -4.6945851e-05+0.004468453186i, -4.7023559e-05+0.004468458361i, -4.7013624e-05+0.004468537157i, -4.7099194e-05+0.004468573619i, -4.699474e-05+0.004468547497i, -4.7128198e-05+0.004468431208i, -4.7120914e-05+0.004468523646i, -4.7165553e-05+0.004468627903i, -4.7193085e-05+0.004468443487i, -4.7242614e-05+0.004468402792i, -4.7213445e-05+0.004468311577i, -4.7357005e-05+0.004468302733i, -4.7296643e-05+0.00446837507i, -4.7400255e-05+0.004468380942i, -4.7394655e-05+0.004468410288i, -4.7404448e-05+0.004468459876i, -4.7418036e-05+0.004468311717i, -4.7497046e-05+0.004468532077i, -4.7486108e-05+0.004468410587i, -4.7590774e-05+0.00446842277i, -4.7614498e-05+0.004468396032i, -4.7588584e-05+0.004468417608i, -4.7592232e-05+0.004468572723i, -4.7685624e-05+0.004468589304i, -4.7701519e-05+0.00446842432i, -4.7709984e-05+0.004468578637i, -4.7793457e-05+0.004468314969i, -4.7855575e-05+0.004468481401i, -4.7734811e-05+0.004468476325i, -4.7816511e-05+0.004468604795i, -4.8003769e-05+0.004468494261i, -4.7921422e-05+0.004468400161i, -4.7986881e-05+0.00446845887i, -4.7973484e-05+0.004468411588i, -4.8007434e-05+0.004468662817i, -4.8077355e-05+0.004468444713i, -4.8004369e-05+0.004468530762i, -4.8114113e-05+0.004468382203i, -4.8166661e-05+0.00446842514i, -4.8090033e-05+0.004468546029i, -4.8151153e-05+0.00446844034i, -4.8218573e-05+0.00446838693i, -4.8273866e-05+0.004468462835i, -4.8247238e-05+0.004468363413i, -4.8273799e-05+0.004468209551i, -4.8293473e-05+0.004468240254i, -4.8390791e-05+0.004468116526i, -4.836375e-05+0.004468119883i, -4.853261e-05+0.004468311768i, -4.8461172e-05+0.004468182548i, -4.8558411e-05+0.004468197657i, -4.8595469e-05+0.004468263596i, -4.8510485e-05+0.004468160739i, -4.8615841e-05+0.004468180985i, -4.8676982e-05+0.004468175333i, -4.876049e-05+0.004468083475i, -4.8716641e-05+0.004468269615i, -4.8718498e-05+0.004468337309i, -4.8795645e-05+0.004468234497i, -4.8880627e-05+0.004468315221i, -4.8921239e-05+0.004468173046i, -4.8880722e-05+0.004468242835i, -4.8866442e-05+0.004468161946i, -4.8897154e-05+0.004468301497i, -4.8946592e-05+0.004468273677i, -4.8949298e-05+0.004468328775i, -4.9084194e-05+0.004468203626i, -4.9021072e-05+0.004468174086i, -4.9085515e-05+0.004468017192i, -4.9035314e-05+0.004468333101i, -4.9138187e-05+0.004468046886i, -4.9223008e-05+0.004468135196i, -4.9191606e-05+0.004468264186i, -4.9243132e-05+0.004468000774i, -4.9232882e-05+0.004467899067i, -4.9320587e-05+0.00446809935i, -4.930736e-05+0.004468193566i, -4.938536e-05+0.004468152209i, -4.9342458e-05+0.004468110248i, -4.9394543e-05+0.004467947152i, -4.947677e-05+0.004468097327i, -4.9478119e-05+0.004468230914i, -4.9573553e-05+0.004468272213i, -4.9541645e-05+0.004468062947i, -4.9526329e-05+0.004468072323i, -4.9615748e-05+0.004468204362i, -4.9541255e-05+0.004468218345i, -4.9656587e-05+0.00446810851i, -4.9676457e-05+0.004468051541i, -4.9681257e-05+0.004468013539i, -4.9688302e-05+0.00446789339i, -4.9786088e-05+0.0044680188i, -4.9745335e-05+0.004468037661i, -4.9847389e-05+0.004467989498i, -4.9806676e-05+0.004468129783i, -4.9894886e-05+0.004467929551i, -4.9946983e-05+0.004467994269i, -5.0007826e-05+0.004468187989i, -5.0054905e-05+0.004468018378i, -5.0131087e-05+0.004468002978i, -5.0025451e-05+0.004467999084i, -5.0043045e-05+0.004468037447i, -5.013341e-05+0.004467993845i, -5.0126537e-05+0.004467966583i, -5.0142255e-05+0.004468195444i, -5.0241131e-05+0.004467998881i, -5.0274637e-05+0.004467989034i, -5.0354702e-05+0.004468007635i, -5.0266931e-05+0.004468045573i, -5.0365842e-05+0.004467684803i, -5.0395633e-05+0.00446793805i, -5.0454377e-05+0.00446784718i, -5.0475526e-05+0.004468044449i, -5.0537136e-05+0.00446793702i, -5.054242e-05+0.004468046336i, -5.0608082e-05+0.004468080226i, -5.0613823e-05+0.004468052073i, -5.0596732e-05+0.004468079711i, -5.0575663e-05+0.004468066942i, -5.0726353e-05+0.004468152653i, -5.0659036e-05+0.004467955736i, -5.0755259e-05+0.004468058223i, -5.0973454e-05+0.004467938601i, -5.0768784e-05+0.004468006962i, -5.0856428e-05+0.004468149281i, -5.0849267e-05+0.004468011896i, -5.0908828e-05+0.004468035577i, -5.0937618e-05+0.004468157107i, -5.1016219e-05+0.004468023633i, -5.0960905e-05+0.004467925298i, -5.1061672e-05+0.00446806967i, -5.104136e-05+0.004467995942i, -5.1149103e-05+0.004467901418i, -5.1158278e-05+0.004468000569i, -5.093409e-05+0.004467876501i, -5.1177328e-05+0.004467799239i, -5.1191844e-05+0.004467844369i, -5.1233584e-05+0.004467915589i, -5.1290253e-05+0.004467878888i, -5.1303569e-05+0.004468019658i, -5.1357849e-05+0.004467984947i, -5.133173e-05+0.004467974992i, -5.1460467e-05+0.004467998113i, -5.1447782e-05+0.004468076991i, -5.1466608e-05+0.004468025617i, -5.1562015e-05+0.004467881284i, -5.1526321e-05+0.004467758108i, -5.1540968e-05+0.004467805254i, -5.1660091e-05+0.004467879663i, -5.1592717e-05+0.004467841785i, -5.1616197e-05+0.004467947015i, -5.1612073e-05+0.004467982895i, -5.1708762e-05+0.00446805513i, -5.1739335e-05+0.004468152455i, -5.1787576e-05+0.004467964786i, -5.1825292e-05+0.004467948187i, -5.1791934e-05+0.004467903963i, -5.1809038e-05+0.004467947019i, -5.1846947e-05+0.004468046432i, -5.1894774e-05+0.004467980158i, -5.197284e-05+0.004467870126i, -5.1917877e-05+0.004467896725i, -5.2075765e-05+0.004467989983i, -5.2087922e-05+0.004467931095i, -5.2123551e-05+0.004467936334i, -5.2136292e-05+0.00446792597i, -5.2191561e-05+0.004467902588i, -5.2121775e-05+0.004467865668i, -5.2145884e-05+0.004467822322i, -5.2304744e-05+0.004468120869i, -5.2327339e-05+0.004467842703i, -5.2350835e-05+0.004467907293i, -5.2268265e-05+0.004467841187i, -5.2369646e-05+0.00446785963i, -5.2353952e-05+0.004467699517i, -5.237042e-05+0.004467955213i, -5.2505857e-05+0.004467792377i, -5.2501052e-05+0.004467862558i, -5.2457828e-05+0.004467787761i, -5.2421193e-05+0.004467759611i, -5.2630389e-05+0.004467742135i, -5.2558972e-05+0.004467705324i, -5.2643667e-05+0.004467719533i, -5.2705677e-05+0.004467743729i, -5.2584025e-05+0.004467711867i, -5.2814288e-05+0.004467843776i, -5.2671909e-05+0.004467884259i, -5.2977048e-05+0.004467785407i, -5.282509e-05+0.004467578091i, -5.28554e-05+0.004467535961i, -5.2955652e-05+0.004467668365i, -5.2924259e-05+0.004467658639i, -5.2872247e-05+0.004467628108i, -5.2968949e-05+0.00446756576i, -5.2997665e-05+0.004467780463i, -5.2995668e-05+0.004467675868i, -5.3025208e-05+0.004467668095i, -5.3053741e-05+0.004467654293i, -5.3151149e-05+0.004467793025i, -5.3179148e-05+0.004467898735i, -5.3182383e-05+0.004467860573i, -5.3178135e-05+0.00446768017i, -5.3230482e-05+0.004467638871i, -5.3371994e-05+0.004467475993i, -5.3335715e-05+0.004467646995i, -5.3353386e-05+0.004467723856i, -5.3403043e-05+0.004467597475i, -5.3466833e-05+0.004467656562i, -5.340223e-05+0.004467743967i, -5.3474451e-05+0.00446749209i, -5.3494433e-05+0.004467728107i, -5.3611526e-05+0.004467738582i, -5.3610174e-05+0.004467578943i, -5.3566025e-05+0.004467587353i, -5.3633441e-05+0.004467736057i, -5.361029e-05+0.004467614817i, -5.3722075e-05+0.004467600156i, -5.3707107e-05+0.004467597813i, -5.3827988e-05+0.004467613863i, -5.3740196e-05+0.004467682595i, -5.3848572e-05+0.004467572449i, -5.3850229e-05+0.004467666565i, -5.3901124e-05+0.004467637488i, -5.3976867e-05+0.004467665495i, -5.3912026e-05+0.004467575883i, -5.3968099e-05+0.004467484051i, -5.4057191e-05+0.004467595669i, -5.4041775e-05+0.004467454683i, -5.4039943e-05+0.004467520896i, -5.4149967e-05+0.004467322545i, -5.4126469e-05+0.004467258945i, -5.4138094e-05+0.004467595807i, -5.4195629e-05+0.00446751954i, -5.4159129e-05+0.004467443013i, -5.4279412e-05+0.004467526138i, -5.4327716e-05+0.004467558479i, -5.4241263e-05+0.00446740005i, -5.4314664e-05+0.004467406353i, -5.4329995e-05+0.004467444025i, -5.432726e-05+0.004467263073i, -5.4423961e-05+0.004467319797i, -5.4574735e-05+0.004467308214i, -5.4457607e-05+0.004467232544i, -5.4489789e-05+0.004467413065i, -5.45335e-05+0.004467499779i, -5.4550878e-05+0.004467502018i, -5.4633644e-05+0.004467403344i, -5.4583028e-05+0.004467406343i, -5.4664244e-05+0.004467284792i, -5.4703824e-05+0.004467438953i, -5.4705515e-05+0.004467492981i, -5.471695e-05+0.004467438019i, -5.4770635e-05+0.00446724667i, -5.4804141e-05+0.004467244173i, -5.483673e-05+0.004467489089i, -5.4908156e-05+0.004467360693i, -5.4955906e-05+0.004467224519i, -5.4912975e-05+0.00446737892i, -5.4985964e-05+0.004467306725i, -5.5071043e-05+0.004467248497i, -5.4973198e-05+0.004467524654i, -5.5064601e-05+0.00446748105i, -5.5041855e-05+0.004467340833i, -5.5129745e-05+0.004467381143i, -5.5226637e-05+0.004467296125i, -5.5283052e-05+0.00446732438i, -5.5181938e-05+0.004467428443i, -5.5258353e-05+0.004467142581i, -5.5281886e-05+0.004467441532i, -5.5328597e-05+0.004467474357i, -5.5426216e-05+0.004467431514i, -5.531612e-05+0.004467258228i, -5.5404156e-05+0.004467315203i, -5.5449875e-05+0.00446723571i, -5.5496064e-05+0.004467262712i, -5.5494988e-05+0.004467500435i, -5.5515694e-05+0.004467425428i, -5.5526659e-05+0.004467334671i, -5.5574421e-05+0.004467397766i, -5.5623942e-05+0.004467494612i, -5.5705619e-05+0.004467330783i, -5.5735565e-05+0.00446738022i, -5.5784027e-05+0.004467273789i, -5.5799593e-05+0.00446720712i, -5.5769699e-05+0.004467193934i, -5.5809331e-05+0.004467396489i, -5.5856731e-05+0.004467381159i, -5.5918598e-05+0.004467383342i, -5.5943623e-05+0.004467492577i, -5.5982816e-05+0.004467299795i, -5.5923061e-05+0.004467329594i, -5.6021779e-05+0.004467293389i, -5.6052196e-05+0.004467193341i, -5.5982932e-05+0.004467195583i, -5.6131563e-05+0.004467432624i, -5.6131463e-05+0.004467020688i, -5.6239143e-05+0.004467097201i, -5.6189046e-05+0.004467109332i, -5.6273374e-05+0.004467383013i, -5.6290465e-05+0.004467271293i, -5.6338687e-05+0.004467295426i, -5.6394581e-05+0.004467365498i, -5.6325218e-05+0.004467296506i, -5.6395903e-05+0.004467330453i, -5.6450473e-05+0.00446712156i, -5.6465083e-05+0.004467048011i, -5.6499203e-05+0.004467297297i, -5.6554646e-05+0.00446726264i, -5.6562596e-05+0.004467103709i, -5.6619906e-05+0.004466853416i, -5.6625538e-05+0.004467163146i, -5.6664111e-05+0.004467099921i, -5.6568977e-05+0.004467323696i, -5.6688776e-05+0.004467254125i, -5.6724243e-05+0.004467085193i, -5.6692874e-05+0.004467045732i, -5.6798625e-05+0.004466967829i, -5.6895365e-05+0.004466985568i, -5.6843114e-05+0.004467104359i, -5.6886127e-05+0.004466846857i, -5.6804365e-05+0.004466914844i, -5.6922962e-05+0.004466916858i, -5.6958676e-05+0.004466947203i, -5.7009033e-05+0.004466765554i, -5.6989363e-05+0.004466886065i, -5.7061818e-05+0.004466769773i, -5.7059341e-05+0.004466845162i, -5.7095928e-05+0.004466941418i, -5.7166078e-05+0.004466827389i, -5.7164798e-05+0.004466867627i, -5.7172354e-05+0.004466820734i, -5.7274337e-05+0.004466876469i, -5.7272252e-05+0.004466960572i, -5.7298887e-05+0.004466866344i, -5.7415214e-05+0.00446690351i, -5.7402905e-05+0.004467130646i, -5.7412652e-05+0.004466843238i, -5.7444639e-05+0.004466898322i, -5.7495846e-05+0.004466862764i, -5.747254e-05+0.004466962551i, -5.74823e-05+0.004467072598i, -5.7606125e-05+0.00446698324i, -5.758408e-05+0.00446695407i, -5.7629909e-05+0.004466834578i, -5.7733583e-05+0.004467039811i, -5.7620567e-05+0.004467006495i, -5.7641878e-05+0.004467088801i, -5.7648723e-05+0.004466897188i, -5.7811082e-05+0.004466898988i, -5.7721079e-05+0.004466936681i, -5.7823486e-05+0.004467072574i, -5.7853732e-05+0.004466841664i, -5.7850832e-05+0.004467035162i, -5.790631e-05+0.004466797483i, -5.793306e-05+0.004466885919i, -5.7992561e-05+0.004466902137i, -5.797725e-05+0.00446682516i, -5.8049344e-05+0.004467058838i, -5.8093679e-05+0.004466920363i, -5.8183846e-05+0.004466832214i, -5.8150794e-05+0.004466732066i, -5.8137581e-05+0.00446665725i, -5.8131315e-05+0.004466796874i, -5.8220046e-05+0.004466687212i, -5.8294264e-05+0.004466822566i, -5.8299367e-05+0.004466886175i, -5.8335329e-05+0.004466937406i, -5.8408587e-05+0.004467044856i, -5.8384832e-05+0.004466969881i, -5.8485695e-05+0.004466775606i, -5.8420124e-05+0.004466940213i, -5.8510371e-05+0.004467019166i, -5.8576065e-05+0.004466978639i, -5.8597483e-05+0.004466778921i, -5.8595415e-05+0.004466922762i, -5.8689473e-05+0.004467039287i, -5.8532034e-05+0.004466942055i, -5.8712365e-05+0.004466784908i, -5.8715099e-05+0.004466893381i, -5.8704046e-05+0.004466864726i, -5.8809797e-05+0.004466926509i, -5.8756399e-05+0.004466877536i, -5.8922826e-05+0.004466813625i, -5.8912314e-05+0.0044667159i, -5.8826474e-05+0.004466770181i, -5.8899562e-05+0.004466931375i, -5.8977556e-05+0.004466977535i, -5.8960478e-05+0.004466906226i, -5.8969322e-05+0.004467046056i, -5.9017645e-05+0.004466966134i, -5.9107299e-05+0.004466791534i, -5.9093643e-05+0.004466743989i, -5.9136581e-05+0.004466847434i, -5.9152994e-05+0.00446680386i, -5.9219437e-05+0.004466859497i, -5.9260506e-05+0.004466904067i, -5.9233261e-05+0.004466926491i, -5.9284839e-05+0.004466850631i, -5.9323523e-05+0.004466816265i, -5.9308815e-05+0.004466743877i, -5.9438558e-05+0.004466661084i, -5.9394837e-05+0.004466853195i, -5.9483734e-05+0.004466869107i, -5.9473045e-05+0.004466784397i, -5.9560637e-05+0.004466645911i, -5.9551553e-05+0.004466558131i, -5.9575403e-05+0.004466753636i, -5.964229e-05+0.004466617228i, -5.9643102e-05+0.004466467587i, -5.971309e-05+0.004466540619i, -5.9694611e-05+0.004466483953i, -5.9752893e-05+0.004466677685i, -5.9768926e-05+0.004466422355i, -5.9793016e-05+0.004466390899i, -5.9807065e-05+0.004466589475i, -5.9816865e-05+0.00446645834i, -5.9847695e-05+0.0044664228i, -5.9901041e-05+0.004466415278i, -5.9917042e-05+0.004466638922i, -5.9961816e-05+0.004466508992i, -5.9939206e-05+0.004466555669i, -6.0058513e-05+0.00446654846i, -6.0034535e-05+0.004466491354i, -6.0119914e-05+0.004466715726i, -6.011417e-05+0.004466754775i, -6.0116241e-05+0.004466536213i, -6.0163061e-05+0.004466477041i, -6.018868e-05+0.004466680839i, -6.0297065e-05+0.004466479476i, -6.0311858e-05+0.004466536519i, -6.0323942e-05+0.004466641918i, -6.0364537e-05+0.004466671987i, -6.0317939e-05+0.004466656251i, -6.0431331e-05+0.004466478387i, -6.0431704e-05+0.00446654047i, -6.0397212e-05+0.004466414168i, -6.0491388e-05+0.004466452091i, -6.0492098e-05+0.004466495351i, -6.0513429e-05+0.004466529808i, -6.0598471e-05+0.004466425946i, -6.0598613e-05+0.004466666729i, -6.0661304e-05+0.004466605641i, -6.0609808e-05+0.004466551628i, -6.0650949e-05+0.004466434353i, -6.0716111e-05+0.004466356882i, -6.0792832e-05+0.004466613054i, -6.0759543e-05+0.004466380925i, -6.0811782e-05+0.004466403993i, -6.080647e-05+0.004466537614i, -6.0825545e-05+0.004466598142i, -6.087612e-05+0.004466481492i, -6.0857293e-05+0.004466309949i, -6.1110761e-05+0.004466571359i, -6.1002565e-05+0.004466415882i, -6.1099274e-05+0.004466356137i, -6.1124302e-05+0.004466360961i, -6.1113117e-05+0.004466444504i, -6.1141808e-05+0.004466359133i, -6.1171526e-05+0.004466430367i, -6.1210136e-05+0.004466619461i, -6.1257247e-05+0.004466432133i, -6.1236668e-05+0.004466538584i, -6.1329447e-05+0.004466405982i, -6.1336074e-05+0.004466477499i, -6.138679e-05+0.004466383564i, -6.1363936e-05+0.004466497062i, -6.1513809e-05+0.004466434213i, -6.1458353e-05+0.004466433592i, -6.1513065e-05+0.004466457925i, -6.1497665e-05+0.004466350779i, -6.1570294e-05+0.004466446864i, -6.1575758e-05+0.004466509623i, -6.1656434e-05+0.004466390555i, -6.1631857e-05+0.004466614086i, -6.1686072e-05+0.004466517548i, -6.1686603e-05+0.004466381953i, -6.1730788e-05+0.004466376586i, -6.1833918e-05+0.004466474204i, -6.1797147e-05+0.004466366562i, -6.1834033e-05+0.004466297449i, -6.1839558e-05+0.004466399783i, -6.1947903e-05+0.004466353923i, -6.1862143e-05+0.004466353073i, -6.1894128e-05+0.004466341215i, -6.1965283e-05+0.004466271436i, -6.2004587e-05+0.004466339791i, -6.1967787e-05+0.0044664327i, -6.2100355e-05+0.004466376489i, -6.2123125e-05+0.004466341063i, -6.2077408e-05+0.004466322616i, -6.2134101e-05+0.0044662366i, -6.2198535e-05+0.004466347066i, -6.2228539e-05+0.004466491606i, -6.2257117e-05+0.004466401659i, -6.2250624e-05+0.004466234629i, -6.2305979e-05+0.00446625758i, -6.2312276e-05+0.004466205459i, -6.2357831e-05+0.004466224099i, -6.242204e-05+0.004466163183i, -6.2472805e-05+0.004466121026i, -6.2494247e-05+0.004466297639i, -6.2500449e-05+0.004466333609i, -6.253013e-05+0.004466241653i, -6.2565578e-05+0.004466163358i, -6.252344e-05+0.004466236927i, -6.2536783e-05+0.004466281587i, -6.2636311e-05+0.004466278237i, -6.2705127e-05+0.004466240176i, -6.2721172e-05+0.004466207976i, -6.2717309e-05+0.004466203481i, -6.2834845e-05+0.004466369683i, -6.2712457e-05+0.004465926363i, -6.2860721e-05+0.004466057819i, -6.2839681e-05+0.004466158637i, -6.2898015e-05+0.004466211535i, -6.2892135e-05+0.004466187868i, -6.2988629e-05+0.004466182862i, -6.296721e-05+0.004466285997i, -6.3138819e-05+0.004466291226i, -6.3065241e-05+0.004466083827i, -6.3029628e-05+0.004466232621i, -6.3195644e-05+0.004466145834i, -6.3127048e-05+0.004466301929i, -6.3177254e-05+0.004466215334i, -6.3203743e-05+0.004466024393i, -6.3232738e-05+0.004466016013i, -6.3273373e-05+0.004466073641i, -6.3245266e-05+0.004466246584i, -6.3321473e-05+0.004466406128i, -6.3417657e-05+0.004466272118i, -6.3359653e-05+0.004466023569i, -6.3479695e-05+0.004466222466i, -6.3454405e-05+0.004466164519i, -6.3494354e-05+0.00446623019i, -6.3477246e-05+0.004466195321i, -6.3488079e-05+0.004466182152i, -6.3608254e-05+0.004466205167i, -6.3735494e-05+0.00446615598i, -6.3641605e-05+0.004466154781i, -6.3607559e-05+0.004466049509i, -6.372426e-05+0.004466301631i, -6.3707844e-05+0.004466167577i, -6.3775454e-05+0.004466198618i, -6.384677e-05+0.004466048001i, -6.3867053e-05+0.004466128804i, -6.3944667e-05+0.004466135923i, -6.3897036e-05+0.004466167209i, -6.3856363e-05+0.00446587713i, -6.3965172e-05+0.00446613005i, -6.4001017e-05+0.004466063018i, -6.3982513e-05+0.00446607653i, -6.410249e-05+0.004466106372i, -6.4086308e-05+0.004466246684i, -6.4080956e-05+0.004466062073i, -6.4150937e-05+0.004465975291i, -6.4163715e-05+0.004466016354i, -6.416576e-05+0.00446603068i, -6.4204543e-05+0.004465932722i, -6.4245722e-05+0.00446594579i, -6.4317388e-05+0.00446608878i, -6.4360044e-05+0.004466078837i, -6.4380138e-05+0.004465919967i, -6.4322762e-05+0.004465981022i, -6.4459485e-05+0.004465920462i, -6.4354582e-05+0.004465978277i, -6.4502522e-05+0.004465802563i, -6.4490306e-05+0.004465956694i, -6.4508648e-05+0.004466158422i, -6.4567011e-05+0.00446586346i, -6.4610572e-05+0.004465856689i, -6.4596931e-05+0.004465924342i, -6.4617555e-05+0.004465924918i, -6.4709348e-05+0.004465922665i, -6.4654543e-05+0.0044658239i, -6.4701224e-05+0.004465898766i, -6.4789231e-05+0.004465923867i, -6.4792708e-05+0.004465874629i, -6.4748763e-05+0.004465908028i, -6.4892545e-05+0.004465962677i, -6.4808652e-05+0.004465896808i, -6.5018474e-05+0.004466022085i, -6.4959639e-05+0.004465810574i, -6.5035022e-05+0.004465934696i, -6.4982219e-05+0.004465949556i, -6.4979515e-05+0.004465767057i, -6.5093893e-05+0.004465939992i, -6.5118706e-05+0.004465845691i, -6.5134019e-05+0.004465758412i, -6.5184888e-05+0.004465998679i, -6.5207703e-05+0.004465829975i, -6.5158048e-05+0.004465868717i, -6.5149469e-05+0.004465838622i, -6.5323523e-05+0.004465833752i, -6.5246927e-05+0.004465944374i, -6.5390326e-05+0.00446586829i, -6.5324085e-05+0.004465962083i, -6.5469609e-05+0.004465921595i, -6.5455143e-05+0.004465752341i, -6.5519345e-05+0.004465734878i, -6.5504414e-05+0.004465890793i, -6.5534907e-05+0.004465768956i, -6.5667e-05+0.004465789622i, -6.558723e-05+0.004465720219i, -6.5660773e-05+0.004465792822i, -6.5649841e-05+0.004465811221i, -6.5703696e-05+0.004465941575i, -6.5679047e-05+0.004465744368i, -6.5814566e-05+0.004465905537i, -6.5773615e-05+0.004465739918i, -6.582409e-05+0.004465675935i, -6.5862092e-05+0.004465970562i, -6.5859635e-05+0.004465832536i, -6.5923361e-05+0.004465745887i, -6.5948711e-05+0.004465810305i, -6.6018586e-05+0.004465836024i, -6.6019281e-05+0.004465691611i, -6.6082849e-05+0.00446570754i, -6.6086701e-05+0.004465734486i, -6.6086381e-05+0.004465792091i, -6.6151293e-05+0.004465848591i, -6.6191151e-05+0.0044658133i, -6.6190912e-05+0.004465926988i, -6.628056e-05+0.004465731586i, -6.6298101e-05+0.004465940346i, -6.6290871e-05+0.00446580989i, -6.6338275e-05+0.004465701059i, -6.6406544e-05+0.00446588464i, -6.6379584e-05+0.004465774019i, -6.6395689e-05+0.004465873373i, -6.6554091e-05+0.004465802113i, -6.6472791e-05+0.004465651019i, -6.6491156e-05+0.004465843131i, -6.6545367e-05+0.004465893121i, -6.6624895e-05+0.004465869785i, -6.6623981e-05+0.004465802926i, -6.6620337e-05+0.004465803468i, -6.6646427e-05+0.004465650477i, -6.6729606e-05+0.004465685152i, -6.6728332e-05+0.004465624866i, -6.6787715e-05+0.00446576141i, -6.6748846e-05+0.004465671463i, -6.6860404e-05+0.004465800767i, -6.6898906e-05+0.004465577691i, -6.6892452e-05+0.004465660167i, -6.6917067e-05+0.004465751886i, -6.6937316e-05+0.00446572862i, -6.6914487e-05+0.004465734769i, -6.7016904e-05+0.00446576243i, -6.6993824e-05+0.004465480406i, -6.701173e-05+0.004465606856i, -6.7008297e-05+0.004465566969i, -6.7104766e-05+0.004465700972i, -6.7171963e-05+0.004465587141i, -6.7129381e-05+0.00446556706i, -6.7240301e-05+0.004465756653i, -6.7220901e-05+0.00446539716i, -6.723732e-05+0.004465640675i, -6.7332366e-05+0.004465591336i, -6.7254744e-05+0.004465573965i, -6.7380372e-05+0.004465741639i, -6.7381752e-05+0.004465462148i, -6.7413796e-05+0.004465526325i, -6.7432221e-05+0.00446568038i, -6.7461069e-05+0.004465648298i, -6.746872e-05+0.004465426448i, -6.7579157e-05+0.004465444404i, -6.7574027e-05+0.00446549191i, -6.761239e-05+0.004465570803i, -6.7602423e-05+0.004465540694i, -6.7686993e-05+0.004465682203i, -6.7713024e-05+0.004465500513i, -6.7772442e-05+0.004465624304i, -6.7734723e-05+0.004465530508i, -6.77858e-05+0.004465417533i, -6.7817953e-05+0.004465516916i, -6.7844528e-05+0.004465703345i, -6.7852714e-05+0.004465666788i, -6.7846012e-05+0.00446570353i, -6.7985175e-05+0.004465511468i, -6.8018372e-05+0.004465529507i, -6.8030573e-05+0.004465555122i, -6.811413e-05+0.004465581103i, -6.8079509e-05+0.004465545122i, -6.8014683e-05+0.004465456815i, -6.8202927e-05+0.004465460537i, -6.8141817e-05+0.004465376681i, -6.8223146e-05+0.004465333053i, -6.820623e-05+0.004465593071i, -6.8219497e-05+0.004465508954i, -6.8279546e-05+0.004465319828i, -6.8309791e-05+0.004465635386i, -6.8357536e-05+0.004465424068i, -6.835724e-05+0.004465550257i, -6.8394595e-05+0.004465543095i, -6.8460283e-05+0.004465491651i, -6.8499431e-05+0.004465376476i, -6.8502149e-05+0.004465507034i, -6.8538101e-05+0.004465464065i, -6.8483282e-05+0.004465344276i, -6.8608942e-05+0.004465434189i, -6.8615553e-05+0.004465636533i, -6.8591773e-05+0.004465505377i, -6.870402e-05+0.004465475916i, -6.8734727e-05+0.004465520161i, -6.8823083e-05+0.004465480597i, -6.8822124e-05+0.004465680022i, -6.8734893e-05+0.004465674685i, -6.8799701e-05+0.004465621042i, -6.8912198e-05+0.004465625185i, -6.8898708e-05+0.004465482418i, -6.9018873e-05+0.004465572735i, -6.8916585e-05+0.004465530724i, -6.8989589e-05+0.004465401201i, -6.9064798e-05+0.004465644516i, -6.9067766e-05+0.004465572264i, -6.9193853e-05+0.004465523384i, -6.9095005e-05+0.004465602004i, -6.9239366e-05+0.004465577431i, -6.9208258e-05+0.004465550477i, -6.9189957e-05+0.004465672868i, -6.9228181e-05+0.004465687971i, -6.9282054e-05+0.004465637272i, -6.9321635e-05+0.004465724523i, -6.9360112e-05+0.004465669202i, -6.9323694e-05+0.004465474029i, -6.9394524e-05+0.004465618638i, -6.9388459e-05+0.004465591062i, -6.9530615e-05+0.004465591999i, -6.9479569e-05+0.004465470127i, -6.9504453e-05+0.0044656023i, -6.9556324e-05+0.004465621182i, -6.962416e-05+0.004465491215i, -6.9608345e-05+0.004465686996i, -6.9643366e-05+0.004465610657i, -6.9539657e-05+0.004465303873i, -6.971187e-05+0.004465289203i, -6.9691232e-05+0.004465217185i, -6.9789454e-05+0.004465509212i, -6.9757283e-05+0.004465413776i, -6.9943313e-05+0.004465464808i, -6.9828829e-05+0.004465348567i, -6.9938654e-05+0.004465410586i, -6.995509e-05+0.00446534617i, -6.9908248e-05+0.004465133619i, -7.0010254e-05+0.004465353935i, -6.9935744e-05+0.004465400717i, -6.999025e-05+0.004465331314i, -7.00604e-05+0.004465357083i, -7.0161926e-05+0.004465195936i, -7.0182108e-05+0.004465178929i, -7.0152013e-05+0.004465184551i, -7.0173711e-05+0.004465139803i, -7.0267303e-05+0.004465399234i, -7.0216172e-05+0.004465306251i, -7.0282106e-05+0.004465292354i, -7.0347204e-05+0.004465202177i, -7.0323705e-05+0.004465198781i, -7.0373152e-05+0.0044651965i, -7.0382004e-05+0.004465227172i, -7.0459037e-05+0.004465359203i, -7.0504212e-05+0.004465284048i, -7.0487193e-05+0.004465169616i, -7.0469095e-05+0.004465225952i, -7.0585384e-05+0.004465181887i, -7.054157e-05+0.004465247597i, -7.0597561e-05+0.004465237375i, -7.067261e-05+0.004465452788i, -7.0680727e-05+0.004465432745i, -7.0612972e-05+0.004465521445i, -7.0744193e-05+0.004465416469i, -7.0748031e-05+0.004465239608i, -7.078772e-05+0.004465357895i, -7.0789778e-05+0.004465400957i, -7.0868313e-05+0.004465383528i, -7.0949095e-05+0.004465313041i, -7.0908265e-05+0.004465222015i, -7.0995866e-05+0.004465216744i, -7.0977679e-05+0.004465280441i, -7.1050137e-05+0.004465355751i, -7.1065265e-05+0.004465407267i, -7.1092211e-05+0.004465414789i, -7.1081011e-05+0.004465286246i, -7.1211211e-05+0.004465455941i, -7.10798e-05+0.004465371805i, -7.1177067e-05+0.004465286802i, -7.1269014e-05+0.004465352027i, -7.1302323e-05+0.004465219255i, -7.1321952e-05+0.004465263652i, -7.1380058e-05+0.00446534041i, -7.1432688e-05+0.004465311539i, -7.1385306e-05+0.004465489833i, -7.1422388e-05+0.004465426836i, -7.1535885e-05+0.004465431458i, -7.1420219e-05+0.004465310556i, -7.1539003e-05+0.004465266159i, -7.1581083e-05+0.004465405052i, -7.1643209e-05+0.004465442281i, -7.1656734e-05+0.004465317566i, -7.162625e-05+0.004465296743i, -7.1711158e-05+0.004465366039i, -7.1739401e-05+0.004465310658i, -7.1771144e-05+0.004465340018i, -7.1807391e-05+0.004465390472i, -7.179477e-05+0.004465365965i, -7.1810199e-05+0.004465310069i, -7.1778417e-05+0.004465154299i, -7.1886417e-05+0.004465438177i, -7.1963186e-05+0.004465419059i, -7.19113e-05+0.004465462151i, -7.1963737e-05+0.004465403075i, -7.1984297e-05+0.004465476202i, -7.2037287e-05+0.004465195636i, -7.1995717e-05+0.004465227975i, -7.2119324e-05+0.004465375597i, -7.2113317e-05+0.004465323777i, -7.2134157e-05+0.004465546482i, -7.2238557e-05+0.004465468415i, -7.2174818e-05+0.004465260148i, -7.2270373e-05+0.004465621558i, -7.2271701e-05+0.004465555262i, -7.2352267e-05+0.00446568774i, -7.2217375e-05+0.004465268454i, -7.235449e-05+0.004465465426i, -7.2401117e-05+0.004465379136i, -7.2407455e-05+0.004465266592i, -7.244351e-05+0.004465244838i, -7.2484637e-05+0.004465131982i, -7.2510056e-05+0.004465133147i, -7.2568118e-05+0.004465312529i, -7.2642337e-05+0.004465436965i, -7.2557893e-05+0.0044653486i, -7.2540278e-05+0.0044652064i, -7.2653713e-05+0.004465392479i, -7.265933e-05+0.004465304874i, -7.2699212e-05+0.004465277833i, -7.2751236e-05+0.004465057532i, -7.2819528e-05+0.004465232328i, -7.2816839e-05+0.004465252945i, -7.2791167e-05+0.004465329729i, -7.2903092e-05+0.004465433188i, -7.2960288e-05+0.004465299225i, -7.3002921e-05+0.004465255867i, -7.3007053e-05+0.004465313073i, -7.3071813e-05+0.004465411128i, -7.311378e-05+0.004465390953i, -7.2997988e-05+0.004465410828i, -7.3137334e-05+0.004465470685i, -7.3160525e-05+0.004465372524i, -7.3174919e-05+0.004465259991i, -7.3258236e-05+0.004465282253i, -7.330083e-05+0.004465513052i, -7.3321821e-05+0.004465608882i, -7.3289961e-05+0.004465579493i, -7.3330977e-05+0.004465826257i, -7.3383894e-05+0.004465650881i, -7.3338754e-05+0.004465820429i, -7.3513741e-05+0.004465724769i, -7.3500553e-05+0.004465790416i, -7.3488255e-05+0.00446589047i, -7.3544284e-05+0.004466037021i, -7.3559923e-05+0.004465930306i, -7.3607591e-05+0.004466019741i, -7.367282e-05+0.004465948551i, -7.3720749e-05+0.004466114376i, -7.3780928e-05+0.00446615233i, -7.3738546e-05+0.004466223937i, -7.3835424e-05+0.00446654088i, -7.3880297e-05+0.004466375574i, -7.3835929e-05+0.004466537534i, -7.3892112e-05+0.004466754504i, -7.4029323e-05+0.00446694306i, -7.4083956e-05+0.004467329721i, -7.416138e-05+0.00446774674i, -7.4155388e-05+0.004468301013i, -7.4253099e-05+0.004469003408i, -7.4449789e-05+0.00446979221i, -7.4659471e-05+0.004471125679i, -7.5267461e-05+0.004473736105i, -7.7024892e-05+0.004479427145i, -9.2152283e-05+0.004499570826i, -9.3490464e-05+0.004425926959i, -7.6383961e-05+0.00444951792i, -7.4804245e-05+0.00445529795i, -7.4526225e-05+0.00445796447i, -7.4366575e-05+0.004459600066i, -7.4364738e-05+0.004460582162i, -7.4345304e-05+0.004461206979i, -7.4449982e-05+0.004461694077i, -7.4325954e-05+0.004461994738i, -7.4380576e-05+0.004462140478i, -7.437292e-05+0.004462579659i, -7.4461046e-05+0.004462699863i, -7.4473051e-05+0.004462813307i, -7.4429685e-05+0.004462967542i, -7.4560489e-05+0.004463163834i, -7.4622834e-05+0.004463062312i, -7.4553607e-05+0.00446332604i, -7.4599544e-05+0.004463215564i, -7.4622979e-05+0.004463555178i, -7.4684519e-05+0.004463507665i, -7.4660427e-05+0.004463582175i, -7.4689309e-05+0.004463614089i, -7.4757841e-05+0.004463734444i, -7.4761604e-05+0.004463681245i, -7.4807549e-05+0.00446358509i, -7.4936963e-05+0.004463671795i, -7.4805506e-05+0.004463649863i, -7.4881967e-05+0.004463529041i, -7.4953051e-05+0.004463736207i, -7.4957866e-05+0.00446372145i, -7.5068795e-05+0.004463691534i, -7.5013587e-05+0.00446370677i, -7.5110293e-05+0.004463717113i, -7.5074362e-05+0.004463812367i, -7.5159058e-05+0.004463885545i, -7.5129405e-05+0.004463783928i, -7.5149308e-05+0.004463836119i, -7.5268892e-05+0.004463618104i, -7.5276753e-05+0.004463805636i, -7.5275777e-05+0.00446396323i, -7.5360939e-05+0.004463711878i, -7.5363021e-05+0.004463834989i, -7.5399993e-05+0.004464132797i, -7.5435147e-05+0.004463948877i, -7.547693e-05+0.004463804715i, -7.5462805e-05+0.004464044266i, -7.5460792e-05+0.004463919877i, -7.5597002e-05+0.004464032484i, -7.5561338e-05+0.004463929527i, -7.5592396e-05+0.004464084176i, -7.5659794e-05+0.004464214248i, -7.5725031e-05+0.004464092466i, -7.5691478e-05+0.004464224262i, -7.5832627e-05+0.004464166637i, -7.5869519e-05+0.004464100435i, -7.5742905e-05+0.004464207598i, -7.5865856e-05+0.004464246908i, -7.5897569e-05+0.00446404123i, -7.58818e-05+0.00446410052i, -7.6000737e-05+0.004464011825i, -7.5919207e-05+0.004464172915i, -7.5958424e-05+0.004464196757i, -7.6024531e-05+0.004464126278i, -7.6054587e-05+0.004464226181i, -7.6128678e-05+0.004464127809i, -7.615169e-05+0.004464076478i, -7.6107678e-05+0.004463968896i, -7.6206287e-05+0.004464019762i, -7.6274526e-05+0.004464015587i, -7.6305602e-05+0.004464063625i, -7.6297149e-05+0.004463954311i, -7.6358427e-05+0.004463932207i, -7.6417125e-05+0.004464185609i, -7.6348828e-05+0.0044641267i, -7.6385559e-05+0.004464061193i, -7.6458429e-05+0.004464147466i, -7.6491092e-05+0.004463847901i, -7.6467838e-05+0.004464209595i, -7.6467597e-05+0.004464055281i, -7.6512837e-05+0.004464241536i, -7.6516761e-05+0.004464205221i, -7.6599478e-05+0.004464013782i, -7.6676014e-05+0.004463785869i, -7.6595872e-05+0.004463780043i, -7.6602411e-05+0.004463852028i, -7.6696507e-05+0.004463999745i, -7.6764871e-05+0.004464018742i, -7.6855738e-05+0.004464066696i, -7.6796714e-05+0.004463970697i, -7.690283e-05+0.004464116324i, -7.6851655e-05+0.004463991131i, -7.6909103e-05+0.004464177868i, -7.6880324e-05+0.00446396808i, -7.6962875e-05+0.004463927328i, -7.7025848e-05+0.004463922287i, -7.6997769e-05+0.004463910721i, -7.6938297e-05+0.004463875309i, -7.703308e-05+0.004464019603i, -7.7127019e-05+0.004463946539i, -7.7088047e-05+0.004463962282i, -7.7145966e-05+0.004463845597i, -7.7138321e-05+0.004463823142i, -7.7225365e-05+0.004463753272i, -7.729974e-05+0.004463928808i, -7.7335162e-05+0.00446384212i, -7.730464e-05+0.004463930595i, -7.7345271e-05+0.004463909792i, -7.7416185e-05+0.004463924819i, -7.739847e-05+0.004463913493i, -7.7480111e-05+0.004463887437i, -7.7404229e-05+0.004463733821i, -7.7520918e-05+0.00446404495i, -7.7506492e-05+0.00446390299i, -7.7595714e-05+0.004463926907i, -7.754052e-05+0.004463879943i, -7.7686647e-05+0.004463778122i, -7.7597215e-05+0.004463848948i, -7.7685688e-05+0.004463771756i, -7.769511e-05+0.004463771302i, -7.7773913e-05+0.004463829126i, -7.7781239e-05+0.004463733618i, -7.774811e-05+0.004463849309i, -7.7842881e-05+0.004463916087i, -7.7865529e-05+0.004463816244i, -7.7951461e-05+0.004463634272i, -7.7905483e-05+0.004463876024i, -7.8035821e-05+0.004463746844i, -7.810125e-05+0.004463752342i, -7.8016753e-05+0.004463727366i, -7.8096737e-05+0.004463700838i, -7.806878e-05+0.004463869146i, -7.8103586e-05+0.004463680867i, -7.8140811e-05+0.004463859248i, -7.8233451e-05+0.004463906156i, -7.8195941e-05+0.004463915049i, -7.8264694e-05+0.004464006566i, -7.8290001e-05+0.004463842226i, -7.8286317e-05+0.004463906534i, -7.835234e-05+0.004463910876i, -7.8398188e-05+0.004463788733i, -7.8432175e-05+0.004463909474i, -7.8427156e-05+0.004463921312i, -7.8486314e-05+0.004463982866i, -7.8500424e-05+0.004463798762i, -7.8565666e-05+0.004463749293i, -7.8562627e-05+0.004463833224i, -7.8734403e-05+0.004463928448i, -7.8644767e-05+0.004463885356i, -7.8685889e-05+0.004463789294i, -7.8711589e-05+0.0044637123i, -7.8675939e-05+0.004463724504i, -7.8756658e-05+0.00446402495i, -7.8691703e-05+0.004463901942i, -7.8749901e-05+0.004463770655i, -7.8841244e-05+0.004463712882i, -7.8906649e-05+0.004463778032i, -7.8785444e-05+0.004463783266i, -7.8970431e-05+0.004463653126i, -7.8966389e-05+0.004463649024i, -7.891517e-05+0.00446379514i, -7.9057091e-05+0.0044637381i, -7.8961271e-05+0.004463654974i, -7.9064092e-05+0.004463786685i, -7.9160866e-05+0.004463892322i, -7.9123498e-05+0.004463954049i, -7.9154348e-05+0.004463891774i, -7.9159091e-05+0.004463825766i, -7.9235165e-05+0.004463810038i, -7.9243168e-05+0.004463871719i, -7.9254906e-05+0.004463818374i, -7.9324569e-05+0.004463795917i, -7.9308252e-05+0.004463760178i, -7.9436891e-05+0.004463767366i, -7.9407069e-05+0.004463764825i, -7.939796e-05+0.004463685793i, -7.9474144e-05+0.004463675117i, -7.9555116e-05+0.004463861244i, -7.9471167e-05+0.004463627158i, -7.9584218e-05+0.004463724593i, -7.9513475e-05+0.004463787624i, -7.9592333e-05+0.004463756492i, -7.9605868e-05+0.004463871918i, -7.9564015e-05+0.004463761319i, -7.9623096e-05+0.004463781852i, -7.9758927e-05+0.00446386187i, -7.9756216e-05+0.004463634376i, -7.9701911e-05+0.004463787089i, -7.981681e-05+0.004463762272i, -7.9794066e-05+0.004463585463i, -7.9855047e-05+0.004463672514i, -7.9876938e-05+0.004463809603i, -7.9887997e-05+0.004463585078i, -8.0024302e-05+0.004463663772i, -8.0018403e-05+0.004463525248i, -7.9990224e-05+0.004463653078i, -8.0028399e-05+0.00446369689i, -8.0011688e-05+0.004463796699i, -8.0096177e-05+0.004463712092i, -8.0084544e-05+0.004463593407i, -8.0127789e-05+0.004463710118i, -8.0239557e-05+0.004463543924i, -8.0245138e-05+0.004463624653i, -8.0305456e-05+0.004463822371i, -8.035868e-05+0.004463665903i, -8.0434022e-05+0.004463551413i, -8.0300339e-05+0.004463776112i, -8.0368509e-05+0.004463565208i, -8.043805e-05+0.004463687412i, -8.0409655e-05+0.004463599406i, -8.0432683e-05+0.00446365036i, -8.0556187e-05+0.004463659295i, -8.0554201e-05+0.004463692741i, -8.0566436e-05+0.004463624689i, -8.0710662e-05+0.004463719538i, -8.060156e-05+0.004463500296i, -8.0696038e-05+0.004463481156i, -8.0701542e-05+0.004463544689i, -8.0797151e-05+0.004463602079i, -8.0814958e-05+0.004463607754i, -8.0823481e-05+0.004463652542i, -8.0803056e-05+0.004463691166i, -8.0858113e-05+0.004463579702i, -8.0847776e-05+0.004463452325i, -8.0898043e-05+0.004463624305i, -8.1035252e-05+0.004463583157i, -8.099802e-05+0.004463385889i, -8.0985015e-05+0.004463504325i, -8.0991544e-05+0.004463489103i, -8.1044306e-05+0.00446353472i, -8.1075249e-05+0.004463548059i, -8.1084601e-05+0.004463526692i, -8.1168837e-05+0.004463406411i, -8.1267851e-05+0.004463473994i, -8.1314978e-05+0.004463563656i, -8.1271731e-05+0.004463498269i, -8.1209716e-05+0.004463600608i, -8.1373339e-05+0.004463242977i, -8.1307005e-05+0.004463514709i, -8.135192e-05+0.004463561324i, -8.142428e-05+0.004463324185i, -8.1471992e-05+0.004463450852i, -8.1457984e-05+0.004463300594i, -8.1550058e-05+0.004463376439i, -8.1402662e-05+0.004463298662i, -8.1455362e-05+0.004463273413i, -8.1582598e-05+0.004463271852i, -8.1597232e-05+0.004463210244i, -8.1605107e-05+0.004463362858i, -8.1616253e-05+0.004463335973i, -8.1670704e-05+0.004463427397i, -8.1705761e-05+0.004463392755i, -8.1785911e-05+0.004463366531i, -8.1696778e-05+0.004463171011i, -8.1743459e-05+0.004463309473i, -8.179414e-05+0.004463498221i, -8.1821047e-05+0.004463365513i, -8.1863624e-05+0.004463383622i, -8.1962267e-05+0.004463347511i, -8.1964923e-05+0.004463317392i, -8.194827e-05+0.004463567288i, -8.2030929e-05+0.004463382981i, -8.205171e-05+0.004463472375i, -8.2066374e-05+0.004463341992i, -8.2053193e-05+0.004463364596i, -8.2105662e-05+0.004463251876i, -8.2184013e-05+0.004463280142i, -8.2219827e-05+0.004463079182i, -8.2217173e-05+0.004463140473i, -8.2237039e-05+0.004463312008i, -8.2279439e-05+0.004463341739i, -8.2292689e-05+0.004463374532i, -8.2406156e-05+0.004463601508i, -8.2444075e-05+0.004463538712i, -8.2413791e-05+0.004463592754i, -8.2368533e-05+0.004463322718i, -8.2360022e-05+0.004463297927i, -8.252311e-05+0.004463180359i, -8.2576372e-05+0.00446354963i, -8.2608933e-05+0.00446345977i, -8.2611084e-05+0.004463369791i, -8.2608224e-05+0.004463271331i, -8.2685813e-05+0.0044631561i, -8.2694577e-05+0.004463209882i, -8.272539e-05+0.004463449771i, -8.2759007e-05+0.004463377132i, -8.2788444e-05+0.004463408341i, -8.2833499e-05+0.004463422068i, -8.2779649e-05+0.004463187551i, -8.295985e-05+0.004463343773i, -8.2902742e-05+0.004463420248i, -8.2944446e-05+0.004463408505i, -8.2976766e-05+0.004463400202i, -8.3078825e-05+0.004463278579i, -8.3069732e-05+0.004463245131i, -8.3099744e-05+0.004463231177i, -8.3092124e-05+0.004463405601i, -8.3145632e-05+0.004463255125i, -8.3173941e-05+0.004463264149i, -8.3252757e-05+0.004463293978i, -8.3208765e-05+0.00446317868i, -8.3191474e-05+0.004463122928i, -8.3300718e-05+0.004463132368i, -8.3209024e-05+0.004463241414i, -8.3353643e-05+0.004463301052i, -8.3406387e-05+0.004463192985i, -8.3440855e-05+0.004463363114i, -8.3459813e-05+0.004463218702i, -8.3494608e-05+0.00446311825i, -8.3529707e-05+0.004463174851i, -8.3576595e-05+0.004463020088i, -8.3553933e-05+0.004463012289i, -8.3580867e-05+0.004463002164i, -8.3617896e-05+0.00446301221i, -8.3587918e-05+0.004463006032i, -8.3581623e-05+0.004463078055i, -8.3693338e-05+0.0044630347i, -8.3697924e-05+0.004463111063i, -8.3699843e-05+0.004463088521i, -8.3746561e-05+0.004463160267i, -8.3814353e-05+0.004463224779i, -8.3775763e-05+0.004463141042i, -8.3792254e-05+0.004463251728i, -8.3953902e-05+0.004463071608i, -8.3877169e-05+0.004463018779i, -8.3961058e-05+0.004463048969i, -8.3957086e-05+0.004463153401i, -8.3999596e-05+0.004463254199i, -8.3984216e-05+0.004463069112i, -8.4178908e-05+0.004463042182i, -8.4123425e-05+0.004462976609i, -8.4073369e-05+0.004462970248i, -8.4154444e-05+0.004462959922i, -8.4209817e-05+0.004463044296i, -8.4217093e-05+0.004463039876i, -8.421046e-05+0.004462902708i, -8.425334e-05+0.004463058563i, -8.4265342e-05+0.00446297602i, -8.4280106e-05+0.00446301302i, -8.4361266e-05+0.004463238593i, -8.4497715e-05+0.004462920167i, -8.4353656e-05+0.004463038714i, -8.441192e-05+0.004462862731i, -8.4520632e-05+0.004462886525i, -8.4548946e-05+0.004462923052i, -8.4555212e-05+0.004462852351i, -8.4524956e-05+0.004462803418i, -8.4657541e-05+0.004463203693i, -8.4638783e-05+0.004463099226i, -8.4677254e-05+0.004463098151i, -8.4698321e-05+0.004463049038i, -8.4787949e-05+0.004463259516i, -8.4783739e-05+0.004463033861i, -8.4818673e-05+0.004463119857i, -8.4873023e-05+0.004463183294i, -8.4861773e-05+0.004462992988i, -8.4876974e-05+0.004463124497i, -8.4926022e-05+0.00446293611i, -8.50031e-05+0.004462881161i, -8.5002048e-05+0.004462935923i, -8.505045e-05+0.004462916867i, -8.5089561e-05+0.00446312008i, -8.5118086e-05+0.004462979036i, -8.5186381e-05+0.004462911885i, -8.5109214e-05+0.00446305687i, -8.5229334e-05+0.004462979576i, -8.5184644e-05+0.004463018617i, -8.5295135e-05+0.004463067685i, -8.5320033e-05+0.004463138666i, -8.5327381e-05+0.004463065677i, -8.5396573e-05+0.004462990619i, -8.5400074e-05+0.004462948106i, -8.5408032e-05+0.004462913919i, -8.5505645e-05+0.004462912034i, -8.548345e-05+0.004462939956i, -8.5478593e-05+0.004462985175i, -8.5538747e-05+0.004462935442i, -8.5524706e-05+0.004462870273i, -8.5611387e-05+0.004462999167i, -8.5629617e-05+0.004463057961i, -8.5606333e-05+0.004463044449i, -8.5674697e-05+0.004463041184i, -8.5673886e-05+0.004462857655i, -8.5719935e-05+0.00446290722i, -8.5809015e-05+0.004462681841i, -8.5720632e-05+0.004462847365i, -8.5860257e-05+0.004462784273i, -8.5807248e-05+0.004462738252i, -8.5908533e-05+0.004462946399i, -8.6000542e-05+0.004462871008i, -8.5959887e-05+0.004462722881i, -8.6015496e-05+0.004462720653i, -8.5975982e-05+0.004462722325i, -8.6032165e-05+0.004462731315i, -8.6011108e-05+0.0044626663i, -8.6144074e-05+0.004462720145i, -8.6091614e-05+0.004462676873i, -8.6053183e-05+0.004462795667i, -8.6226524e-05+0.004462781192i, -8.620274e-05+0.00446286361i, -8.6271197e-05+0.004462768966i, -8.61989e-05+0.004462799306i, -8.638655e-05+0.004462568208i, -8.6289402e-05+0.004462749924i, -8.6224193e-05+0.004462925035i, -8.6334712e-05+0.004462750391i, -8.6365191e-05+0.004462894333i, -8.6420625e-05+0.004462567039i, -8.6336062e-05+0.004462772429i, -8.6424604e-05+0.004462740324i, -8.6492921e-05+0.004462709915i, -8.6466371e-05+0.004462873177i, -8.6543376e-05+0.004462805335i, -8.6617036e-05+0.004462719391i, -8.6602113e-05+0.004462678768i, -8.6697931e-05+0.004462771823i, -8.6698106e-05+0.004462626538i, -8.6723524e-05+0.004462620942i, -8.6758872e-05+0.004462605934i, -8.6726462e-05+0.004462788036i, -8.6789471e-05+0.004462524927i, -8.6795475e-05+0.004462692141i, -8.6890767e-05+0.004462766804i, -8.6900566e-05+0.004462826014i, -8.6949655e-05+0.004462717206i, -8.6992256e-05+0.004462714315i, -8.7014172e-05+0.004462659283i, -8.7047491e-05+0.004462660073i, -8.7064938e-05+0.004462729519i, -8.7138318e-05+0.004462646457i, -8.7105723e-05+0.004462707609i, -8.7155607e-05+0.004462567148i, -8.7146997e-05+0.004462918993i, -8.7193242e-05+0.004462689895i, -8.7243746e-05+0.004462740287i, -8.7250798e-05+0.004462678571i, -8.734729e-05+0.004462713669i, -8.738104e-05+0.004462540667i, -8.7295096e-05+0.004462264951i, -8.7369279e-05+0.004462478516i, -8.7475672e-05+0.004462566638i, -8.7483123e-05+0.004462707639i, -8.758429e-05+0.004462659098i, -8.7525261e-05+0.004462504898i, -8.75887e-05+0.00446253107i, -8.7654339e-05+0.004462611546i, -8.7675383e-05+0.004462456829i, -8.7658323e-05+0.004462421128i, -8.7694016e-05+0.004462611397i, -8.7703066e-05+0.004462495618i, -8.7748948e-05+0.004462446638i, -8.780926e-05+0.004462512016i, -8.7874841e-05+0.004462541831i, -8.7815531e-05+0.004462569241i, -8.7939954e-05+0.004462465806i, -8.7920597e-05+0.004462574495i, -8.7929813e-05+0.00446266969i, -8.7918274e-05+0.004462573313i, -8.8022729e-05+0.004462551051i, -8.8038222e-05+0.004462501868i, -8.8074091e-05+0.00446237567i, -8.8105049e-05+0.004462416986i, -8.8130427e-05+0.004462534552i, -8.8159331e-05+0.004462525072i, -8.8163401e-05+0.004462522718i, -8.8093834e-05+0.004462517694i, -8.8255636e-05+0.004462519523i, -8.8163163e-05+0.004462513887i, -8.8259543e-05+0.004462222421i, -8.8245363e-05+0.004462495068i, -8.8302304e-05+0.00446236815i, -8.834831e-05+0.004462488418i, -8.8413844e-05+0.004462590925i, -8.8414295e-05+0.00446255099i, -8.8499285e-05+0.004462451345i, -8.8473148e-05+0.004462460223i, -8.8498579e-05+0.004462450006i, -8.8557008e-05+0.004462260982i, -8.8603328e-05+0.004462407786i, -8.8593891e-05+0.004462584258i, -8.8699999e-05+0.004462506709i, -8.8609106e-05+0.004462474186i, -8.8700331e-05+0.004462389175i, -8.8631043e-05+0.004462471301i, -8.8701941e-05+0.004462424827i, -8.8702408e-05+0.004462396766i, -8.8797374e-05+0.004462449681i, -8.8787784e-05+0.004462406614i, -8.8848284e-05+0.004462379517i, -8.8894166e-05+0.004462512504i, -8.893825e-05+0.004462396757i, -8.8947519e-05+0.004462611075i, -8.8993665e-05+0.004462420204i, -8.8975933e-05+0.004462381615i, -8.9052745e-05+0.00446230793i, -8.9056674e-05+0.004462330918i, -8.9088656e-05+0.004462514128i, -8.913771e-05+0.004462436847i, -8.9242433e-05+0.004462543247i, -8.9185853e-05+0.004462482156i, -8.9234896e-05+0.004462357636i, -8.9282886e-05+0.004462533664i, -8.9286955e-05+0.004462584796i, -8.9379231e-05+0.004462362721i, -8.9334227e-05+0.004462595956i, -8.9451811e-05+0.004462456779i, -8.9448526e-05+0.004462426236i, -8.9455732e-05+0.004462511145i, -8.951135e-05+0.004462553169i, -8.9509307e-05+0.004462574502i, -8.9519389e-05+0.004462493196i, -8.9569649e-05+0.004462570159i, -8.9630496e-05+0.004462403571i, -8.9674733e-05+0.00446246745i, -8.9731118e-05+0.004462470382i, -8.973847e-05+0.004462336253i, -8.9765666e-05+0.004462407996i, -8.9786822e-05+0.004462467567i, -8.98466e-05+0.004462441816i, -8.982494099999999e-05+0.004462437403i, -8.9914327e-05+0.0044623929i, -8.9897018e-05+0.004462461742i, -8.993194e-05+0.004462432083i, -8.9975929e-05+0.004462402916i, -9.0016622e-05+0.004462463039i, -9.0037895e-05+0.004462562904i, -9.0097161e-05+0.004462510562i, -9.0104714e-05+0.004462304615i, -9.0130007e-05+0.004462302494i, -9.0127744e-05+0.004462492653i, -9.0145447e-05+0.004462433726i, -9.0162309e-05+0.004462596927i, -9.0220668e-05+0.00446230319i, -9.0268063e-05+0.004462327488i, -9.0219009e-05+0.004462444151i, -9.0405078e-05+0.004462181913i, -9.0335604e-05+0.004462292858i, -9.0529297e-05+0.004462233315i, -9.0477322e-05+0.004462304449i, -9.0480838e-05+0.004462283473i, -9.0463355e-05+0.0044622082i, -9.0488834e-05+0.00446222244i, -9.0513555e-05+0.00446226725i, -9.0530089e-05+0.004462183785i, -9.0565739e-05+0.004462169002i, -9.0639696e-05+0.004462256368i, -9.0646566e-05+0.004462274736i, -9.066038e-05+0.004462389774i, -9.0658797e-05+0.00446228655i, -9.0755777e-05+0.004462250715i, -9.0725351e-05+0.00446229402i, -9.0708873e-05+0.004462173224i, -9.0793863e-05+0.004462193128i, -9.0798477e-05+0.004462446776i, -9.0847642e-05+0.004462272171i, -9.0876983e-05+0.004462124198i, -9.0924609e-05+0.004462231092i, -9.0972653e-05+0.004461993408i, -9.0989446e-05+0.004462123051i, -9.1010613e-05+0.004462381542i, -9.0972646e-05+0.004462057472i, -9.1051313e-05+0.004462054885i, -9.1153572e-05+0.004462130265i, -9.1149073e-05+0.004462026205i, -9.1168483e-05+0.004462087938i, -9.109903e-05+0.004462277894i, -9.1175612e-05+0.004462136199i, -9.1204539e-05+0.004462011846i, -9.1226708e-05+0.004462008024i, -9.1322956e-05+0.004461864238i, -9.13925e-05+0.004462091444i, -9.1298726e-05+0.004462005617i, -9.1351287e-05+0.004462155245i, -9.1394706e-05+0.004461966285i, -9.1484121e-05+0.004462057796i, -9.1455182e-05+0.004462196217i, -9.1567759e-05+0.004462123801i, -9.1510914e-05+0.004462066219i, -9.1623335e-05+0.004461992958i, -9.1650733e-05+0.004462059474i, -9.1670122e-05+0.004462281246i, -9.1673703e-05+0.004462165295i, -9.1690561e-05+0.004462096562i, -9.1776747e-05+0.004462084788i, -9.1857859e-05+0.004462253019i, -9.1763167e-05+0.00446209479i, -9.1966733e-05+0.004462167055i, -9.1835703e-05+0.004462287602i, -9.1885801e-05+0.004462165183i, -9.2032059e-05+0.004462084997i, -9.2020131e-05+0.004462138022i, -9.2077319e-05+0.004462149236i, -9.2022733e-05+0.004462081773i, -9.2068858e-05+0.004461912003i, -9.2140237e-05+0.004462114644i, -9.2142053e-05+0.004461977037i, -9.21473e-05+0.004461930301i, -9.2214305e-05+0.004461981682i, -9.2223033e-05+0.004462089194i, -9.2275363e-05+0.004461787457i, -9.2284454e-05+0.004462075662i, -9.2201148e-05+0.004462096751i, -9.2343972e-05+0.004462189551i, -9.2322388e-05+0.004462076875i, -9.2433891e-05+0.004462093378i, -9.245855e-05+0.004462110017i, -9.2483459e-05+0.004462053566i, -9.2549398e-05+0.004462089174i, -9.2572465e-05+0.004461995862i, -9.2537429e-05+0.004462026919i, -9.2565492e-05+0.004462088854i, -9.2684038e-05+0.004462136287i, -9.2646325e-05+0.004462095875i, -9.2645978e-05+0.004462081787i, -9.2640807e-05+0.004462065617i, -9.2673858e-05+0.004461913373i, -9.2728555e-05+0.004462076649i, -9.2732521e-05+0.004461924996i, -9.2758249e-05+0.004461947528i, -9.2897782e-05+0.00446211527i, -9.2775299e-05+0.004461993219i, -9.2923017e-05+0.004461865869i, -9.2961585e-05+0.004461861873i, -9.2990647e-05+0.004462080354i, -9.2941756e-05+0.004461894789i, -9.3041948e-05+0.004461902703i, -9.307995e-05+0.004461793624i, -9.314637e-05+0.004461995602i, -9.3089273e-05+0.004461770352i, -9.3107814e-05+0.004461897376i, -9.3111728e-05+0.00446169024i, -9.3172052e-05+0.004461784914i, -9.3273698e-05+0.004461827856i, -9.3221885e-05+0.004461779428i, -9.3265833e-05+0.004461906313i, -9.3302282e-05+0.004461702574i, -9.3342182e-05+0.004461815461i, -9.3272578e-05+0.004461777852i, -9.3401516e-05+0.004461849088i, -9.3364449e-05+0.004461926102i, -9.3418443e-05+0.004461826996i, -9.3419499e-05+0.004461782514i, -9.3488167e-05+0.00446158155i, -9.3505839e-05+0.004461761247i, -9.359304e-05+0.004461554492i, -9.3563779e-05+0.004461607533i, -9.3616302e-05+0.004461801526i, -9.3673811e-05+0.004461740261i, -9.3765062e-05+0.004461740689i, -9.3661411e-05+0.004461619087i, -9.3742213e-05+0.004461831697i, -9.3793272e-05+0.004461521181i, -9.3802418e-05+0.004461773964i, -9.386802e-05+0.004461702309i, -9.3826003e-05+0.004461739023i, -9.3904245e-05+0.004461583344i, -9.3813795e-05+0.00446167767i, -9.3954269e-05+0.004461575988i, -9.3960211e-05+0.004461664135i, -9.4157212e-05+0.004461863056i, -9.4085605e-05+0.004461844737i, -9.4136215e-05+0.004461700625i, -9.4120969e-05+0.004461722038i, -9.4244708e-05+0.00446174485i, -9.4208662e-05+0.00446172534i, -9.4171595e-05+0.004461659757i, -9.4329769e-05+0.00446191732i, -9.427633e-05+0.004461887248i, -9.4270217e-05+0.004461746217i, -9.4350287e-05+0.004461641544i, -9.4389057e-05+0.004461764871i, -9.4401229e-05+0.004461541017i, -9.4437887e-05+0.004461701573i, -9.4437192e-05+0.004461644173i, -9.4560682e-05+0.004461703889i, -9.4580072e-05+0.00446180923i, -9.4631225e-05+0.004461539138i, -9.4583917e-05+0.004461556634i, -9.4637597e-05+0.00446190443i, -9.4641894e-05+0.004461554174i, -9.4694295e-05+0.004461734497i, -9.4750235e-05+0.00446175595i, -9.4837564e-05+0.004461760195i, -9.4783078e-05+0.004461610751i, -9.4844638e-05+0.004461666534i, -9.4950511e-05+0.004461649156i, -9.4894327e-05+0.004461827053i, -9.4951087e-05+0.004461726877i, -9.4948696e-05+0.004461743149i, -9.4952907e-05+0.004461385656i, -9.4968706e-05+0.004461495343i, -9.5059358e-05+0.004461620822i, -9.5064863e-05+0.004461492591i, -9.5003835e-05+0.004461531672i, -9.5129949e-05+0.004461683221i, -9.5111613e-05+0.004461648529i, -9.5157071e-05+0.004461691292i, -9.5104124e-05+0.004461732697i, -9.5184735e-05+0.004461589467i, -9.5234292e-05+0.004461534302i, -9.5237578e-05+0.004461616967i, -9.5303988e-05+0.004461690179i, -9.5284565e-05+0.004461614919i, -9.5317083e-05+0.004461682611i, -9.5450567e-05+0.00446150016i, -9.5452627e-05+0.004461649095i, -9.545805e-05+0.004461523774i, -9.5428048e-05+0.004461398423i, -9.55058e-05+0.004461482878i, -9.5552474e-05+0.004461513453i, -9.5540538e-05+0.004461472101i, -9.5609737e-05+0.004461450334i, -9.5664802e-05+0.004461502168i, -9.570917e-05+0.004461502667i, -9.5683283e-05+0.004461538066i, -9.5688642e-05+0.004461405306i, -9.5701016e-05+0.004461382797i, -9.5684445e-05+0.004461305342i, -9.5895022e-05+0.00446127272i, -9.5838367e-05+0.004461078439i, -9.5902272e-05+0.004461270442i, -9.5909147e-05+0.004461406631i, -9.5910415e-05+0.004461552229i, -9.5939464e-05+0.004461387326i, -9.5887128e-05+0.004461390494i, -9.6040514e-05+0.004461340211i, -9.6075853e-05+0.004461341511i, -9.6034489e-05+0.004461168414i, -9.6195929e-05+0.004461341929i, -9.6225438e-05+0.00446138877i, -9.6080307e-05+0.004461229728i, -9.6254725e-05+0.00446130274i, -9.6234101e-05+0.004461186363i, -9.6317887e-05+0.004461294553i, -9.6234791e-05+0.004461395628i, -9.633735e-05+0.004461481413i, -9.6308407e-05+0.004461367582i, -9.6341346e-05+0.004461495124i, -9.6410464e-05+0.004461290091i, -9.641617e-05+0.004461309644i, -9.649407e-05+0.004461287673i, -9.6510463e-05+0.004461360667i, -9.6573389e-05+0.004461268381i, -9.6563726e-05+0.004461384248i, -9.6646095e-05+0.004461527442i, -9.6667348e-05+0.004461286354i, -9.6706306e-05+0.004461288523i, -9.6724914e-05+0.004461467409i, -9.6708796e-05+0.004461457249i, -9.6816456e-05+0.004461501795i, -9.6842442e-05+0.004461557663i, -9.6780645e-05+0.004461453729i, -9.6837906e-05+0.004461380542i, -9.6940877e-05+0.004461526755i, -9.6920586e-05+0.004461375793i, -9.6962737e-05+0.004461413835i, -9.7001066e-05+0.004461430774i, -9.7014345e-05+0.004461401142i, -9.7039093e-05+0.004461441372i, -9.7097086e-05+0.004461448711i, -9.7120325e-05+0.004461580235i, -9.7171441e-05+0.004461491303i, -9.7161227e-05+0.004461465112i, -9.7215601e-05+0.00446145336i, -9.7202764e-05+0.004461573145i, -9.7173123e-05+0.004461370841i, -9.7203587e-05+0.004461552046i, -9.7291313e-05+0.004461473948i, -9.7351917e-05+0.004461485165i, -9.7410254e-05+0.004461383293i, -9.7328429e-05+0.004461440994i, -9.7395819e-05+0.004461269145i, -9.7431854e-05+0.004461125051i, -9.7478612e-05+0.004461449157i, -9.7529159e-05+0.004461381848i, -9.7550581e-05+0.004461230595i, -9.7602254e-05+0.004461303459i, -9.7630726e-05+0.004461431886i, -9.7567045e-05+0.0044613737i, -9.7699966e-05+0.00446108933i, -9.7626707e-05+0.00446114925i, -9.7580137e-05+0.004461177408i, -9.7754269e-05+0.004461176111i, -9.7694074e-05+0.004461257426i, -9.7741678e-05+0.004461124477i, -9.7752613e-05+0.004460897425i, -9.7868516e-05+0.004461066739i, -9.7894631e-05+0.004461339228i, -9.7858814e-05+0.004461268807i, -9.789773e-05+0.00446128325i, -9.7969687e-05+0.004461444974i, -9.8006919e-05+0.004461250226i, -9.8005752e-05+0.004461214883i, -9.8066888e-05+0.004461241892i, -9.8044817e-05+0.004461090062i, -9.8183879e-05+0.004461180684i, -9.8147854e-05+0.004461173671i, -9.8176086e-05+0.004461203315i, -9.8125594e-05+0.004461049276i, -9.8187264e-05+0.004461180255i, -9.8299909e-05+0.004460910728i, -9.8297683e-05+0.004460955934i, -9.8352884e-05+0.004461235843i, -9.8376186e-05+0.004461116906i, -9.8370755e-05+0.004461149368i, -9.8402662e-05+0.004460956706i, -9.8444201e-05+0.004461077734i, -9.8533616e-05+0.004461110147i, -9.8521398e-05+0.004461273138i, -9.8606229e-05+0.004461120373i, -9.8571299e-05+0.004461310276i, -9.8580201e-05+0.004461326361i, -9.8639722e-05+0.004461335134i, -9.8731335e-05+0.004461197754i, -9.867757e-05+0.004461249301i, -9.8762619e-05+0.004461148514i, -9.8800686e-05+0.004461156656i, -9.8765264e-05+0.004461136717i, -9.8880469e-05+0.004460952053i, -9.8895468e-05+0.00446106433i, -9.8971037e-05+0.004461216916i, -9.8969067e-05+0.004461024285i, -9.901559e-05+0.004461211315i, -9.9025353e-05+0.004460966881i, -9.9005475e-05+0.004461157127i, -9.9002247e-05+0.004461144201i, -9.9070083e-05+0.004461065291i, -9.9158342e-05+0.004461126661i, -9.9128034e-05+0.004461098729i, -9.9245586e-05+0.004461106934i, -9.9237157e-05+0.004461066385i, -9.9198839e-05+0.004461129974i, -9.9291511e-05+0.004461223837i, -9.9328824e-05+0.004461019736i, -9.93225e-05+0.004460868272i, -9.9413384e-05+0.004461271782i, -9.9409512e-05+0.004461089799i, -9.9438512e-05+0.004461032864i, -9.9516268e-05+0.004461120468i, -9.9506204e-05+0.004461049085i, -9.9523357e-05+0.004461059231i, -9.9619346e-05+0.00446100561i, -9.9563898e-05+0.004461078612i, -9.9587717e-05+0.004461116849i, -9.9718494e-05+0.004460973169i, -9.9559124e-05+0.004460967293i, -9.9748497e-05+0.004461022129i, -9.9702168e-05+0.004460989655i, -9.9679179e-05+0.004461045769i, -9.9734914e-05+0.004460944704i, -9.9787944e-05+0.004461019105i, -9.9850111e-05+0.004461141073i, -9.9813448e-05+0.00446094753i, -9.9840844e-05+0.004461089802i, -9.9819881e-05+0.004460905804i, -9.9970928e-05+0.004460990357i, -9.9951386e-05+0.004460986001i, -9.9999862e-05+0.004460882468i, -9.9937616e-05+0.004460811227i, -9.9996896e-05+0.004460813793i, -0.000100084118+0.004460908653i, -0.000100107777+0.004461025218i, -0.00010007143+0.004460902902i, -0.000100191858+0.004460878093i, -0.000100223329+0.004460888153i, -0.000100210284+0.004461052634i, -0.000100267844+0.004461007923i, -0.000100251441+0.004460902167i, -0.000100326298+0.004460770739i, -0.000100281083+0.004460825564i, -0.000100320261+0.004460790313i, -0.000100389801+0.004460853013i, -0.000100384735+0.004460899742i, -0.00010044281+0.004460854246i, -0.000100454277+0.004460813116i, -0.000100480021+0.004460944224i, -0.000100544429+0.004460790854i, -0.000100592226+0.004460666776i, -0.000100621191+0.004460715299i, -0.000100543186+0.004460799989i, -0.000100565254+0.004460686278i, -0.000100691376+0.00446072754i, -0.000100714322+0.004460822097i, -0.000100840968+0.004460637916i, -0.000100834398+0.004460840245i, -0.000100818773+0.004460771369i, -0.000100794632+0.004460737201i, -0.000100909687+0.004460778237i, -0.000100972865+0.00446075053i, -0.000100944919+0.00446066278i, -0.000101015216+0.004460533732i, -0.000100989176+0.004460588215i, -0.000101113837+0.004460752741i, -0.000101069407+0.004460754921i, -0.000101178666+0.004460763906i, -0.000101267548+0.004460558538i, -0.000101223084+0.004460741694i, -0.000101265234+0.004460833643i, -0.000101271458+0.004460777214i, -0.000101330837+0.004460984066i, -0.000101404952+0.0044609269869999996i, -0.000101418578+0.004460897529i, -0.000101453368+0.004460889055i, -0.000101427866+0.004460841907i, -0.000101435262+0.004460753286i, -0.000101420871+0.004460852581i, -0.000101461311+0.004460930324i, -0.000101532838+0.004460920661i, -0.000101606661+0.004460827447i, -0.00010157423+0.004460753721i, -0.000101666326+0.004460654565i, -0.000101673346+0.004460684832i, -0.000101650803+0.004460715899i, -0.000101747799+0.004460855898i, -0.000101738798+0.004460606286i, -0.000101784525+0.004460546578i, -0.000101800904+0.004460597008i, -0.000101857236+0.004460673822i, -0.000101894564+0.00446077783i, -0.000101833089+0.004460839785i, -0.000101882322+0.004460730345i, -0.000101955064+0.004460731291i, -0.000101980916+0.004460751528i, -0.000102001528+0.00446076643i, -0.000102089923+0.004460549133i, -0.000101977559+0.004460616928i, -0.000102075102+0.004460603789i, -0.000102014716+0.004460641166i, -0.000102033292+0.004460326225i, -0.000102082477+0.004460350747i, -0.00010224811+0.004460580412i, -0.00010222165+0.004460571569i, -0.000102316293+0.004460548664i, -0.000102280087+0.004460408379i, -0.000102237411+0.004460472722i, -0.000102328683+0.004460567547i, -0.000102320548+0.004460673485i, -0.000102321013+0.004460538229i, -0.000102363626+0.004460726363i, -0.000102485601+0.004460463258i, -0.000102462393+0.004460232625i, -0.000102415634+0.004460586198i, -0.000102445863+0.004460443316i, -0.000102517859+0.004460314967i, -0.000102537559+0.004460398597i, -0.000102580346+0.004460397937i, -0.000102534557+0.004460383224i, -0.000102650478+0.00446046192i, -0.000102670159+0.004460315112i, -0.000102724929+0.004460368474i, -0.000102706314+0.004460349587i, -0.000102767824+0.004460406047i, -0.000102847502+0.004460377199i, -0.000102840116+0.004460443293i, -0.000102915351+0.004460249881i, -0.000102882006+0.004460555197i, -0.000103009469+0.004460490191i, -0.000103039875+0.004460523787i, -0.000103075137+0.004460453928i, -0.00010307631+0.004460307404i, -0.000103084656+0.004460595841i, -0.000103176963+0.004460488605i, -0.000103125916+0.004460424316i, -0.000103219924+0.00446033514i, -0.000103279876+0.004460316469i, -0.000103119441+0.004460363039i, -0.000103332901+0.004460451584i, -0.000103347156+0.004460415634i, -0.000103402519+0.004460445173i, -0.000103398784+0.00446043167i, -0.000103396032+0.00446031904i, -0.000103519844+0.004460348336i, -0.00010352137+0.004460329476i, -0.000103572423+0.004460399412i, -0.000103612096+0.004460513732i, -0.000103663124+0.004460689953i, -0.000103709536+0.004460512315i, -0.000103716806+0.00446045012i, -0.000103831968+0.004460612357i, -0.000104225558+0.004460788965i, -0.000104360432+0.00446009963i, -0.000103880641+0.004459877534i, -0.000103865657+0.004460147524i, -0.000103907834+0.004460215876i, -0.000103812866+0.004460150365i, -0.000103852014+0.004460252963i, -0.000103911172+0.004460329799i, -0.000103994855+0.004460340211i, -0.000103981188+0.004460209503i, -0.000104028839+0.004460354602i, -0.000103993655+0.004460379999i, -0.000104016709+0.004460264448i, -0.000104039208+0.00446016218i, -0.000104152762+0.004460340558i, -0.00010416133+0.004460261896i, -0.000104192208+0.00446039814i, -0.00010422226+0.004460230039i, -0.000104289821+0.004460288052i, -0.000104318103+0.004460110672i, -0.000104297972+0.004460109579i, -0.000104342525+0.004460102107i, -0.000104284349+0.004460157565i, -0.000104308313+0.004460194559i, -0.00010437268+0.004460241331i, -0.000104362632+0.004460032318i, -0.000104409877+0.004459956099i, -0.000104468011+0.004460144646i, -0.000104517123+0.004459943098i, -0.000104493537+0.004459905329i, -0.000104440675+0.004459891853i, -0.000104597706+0.004460023374i, -0.000104575801+0.004460068448i, -0.000104550717+0.004460220426i, -0.000104616556+0.004460167505i, -0.000104718418+0.004460163011i, -0.000104725747+0.004460096146i, -0.00010467492+0.004460157237i, -0.000104769613+0.004460042781i, -0.000104798826+0.004460198871i, -0.00010473858+0.004460181124i, -0.000104869685+0.00446030527i, -0.000104875887+0.004460230977i, -0.000104908678+0.004460078364i, -0.00010492068+0.004460149675i, -0.00010495399+0.004460092712i, -0.000104981026+0.004460106318i, -0.000105010721+0.004459990857i, -0.000104995539+0.004460067807i, -0.00010513873+0.004460230877i, -0.000105093051+0.004460275455i, -0.000105213183+0.004460018086i, -0.000105233585+0.004460144508i, -0.000105242282+0.004460202097i, -0.000105275727+0.004460082997i, -0.000105360413+0.00446005295i, -0.00010538841+0.004460195409i, -0.000105355303+0.004460238437i, -0.000105444175+0.004460220189i, -0.000105389931+0.004459973805i, -0.000105403688+0.004460152882i, -0.000105510023+0.004460142255i, -0.000105497421+0.004460121835i, -0.000105548924+0.004460168038i, -0.00010556893+0.004460146548i, -0.000105604433+0.004459941095i, -0.000105601596+0.004459978932i, -0.000105664134+0.004460139191i, -0.000105738658+0.004460084706i, -0.000105734591+0.004460057543i, -0.000105858971+0.004460213089i, -0.000105875448+0.004460152723i, -0.000105932391+0.004460263644i, -0.000105934298+0.004460212372i, -0.000105931062+0.0044600547i, -0.000105965179+0.004460140264i, -0.000106023995+0.004460046738i, -0.000106043269+0.004460157889i, -0.000106088243+0.004459998568i, -0.000106092064+0.004460121693i, -0.000106139803+0.004460081751i, -0.000106187085+0.004459955552i, -0.000106195636+0.004460119906i, -0.000106199981+0.004459979358i, -0.000106222862+0.004460057096i, -0.000106233005+0.004459925015i, -0.000106322835+0.004459990052i, -0.000106293386+0.00445995604i, -0.000106275141+0.004460066193i, -0.000106335639+0.004459771438i, -0.000106441211+0.004459981155i, -0.000106438304+0.004460141509i, -0.000106363912+0.004460097013i, -0.000106471184+0.004459921552i, -0.000106555172+0.00445992023i, -0.000106642929+0.004459959496i, -0.00010650098+0.004459898864i, -0.000106549601+0.004460035758i, -0.000106589001+0.004459820353i, -0.000106598326+0.004459943134i, -0.000106655975+0.004459861422i, -0.00010668175+0.004459944547i, -0.000106662148+0.004459752425i, -0.000106730171+0.004459637695i, -0.000106605382+0.004459756278i, -0.000106780734+0.004459713411i, -0.000106735442+0.004459662773i, -0.000106794231+0.004459656912i, -0.000106893859+0.004459885567i, -0.0001069509+0.004459843077i, -0.000106993006+0.004459803884i, -0.000106940659+0.004459712393i, -0.00010703871+0.004459666082i, -0.000107030344+0.004459860366i, -0.00010704188+0.004459827945i, -0.000107107195+0.004459813024i, -0.00010705856+0.00445976061i, -0.000107147748+0.004459668897i, -0.000107061903+0.004459688287i, -0.000107149331+0.004459715729i, -0.000107143992+0.004459631684i, -0.000107294177+0.004459694247i, -0.000107241958+0.004459530355i, -0.000107247264+0.004459469017i, -0.000107339789+0.004459742945i, -0.000107329564+0.00445967201i, -0.000107414187+0.004459616607i, -0.00010751904+0.004459729678i, -0.000107510689+0.004459615497i, -0.000107541666+0.004459526866i, -0.000107527836+0.004459639437i, -0.000107598145+0.004459375828i, -0.000107625554+0.004459735426i, -0.000107704023+0.004459462737i, -0.000107733428+0.004459529928i, -0.000107727839+0.004459596928i, -0.000107706868+0.004459550543i, -0.000107739523+0.00445960246i, -0.000107788551+0.004459693267i, -0.000107854047+0.004459725358i, -0.000107897998+0.004459645151i, -0.000107958819+0.004459676775i, -0.000107991817+0.004459779996i, -0.000107996729+0.004459713079i, -0.00010797007+0.004459682502i, -0.000108094354+0.004459741696i, -0.000108077185+0.004459815177i, -0.000108062572+0.004459582701i, -0.000108099129+0.004459762396i, -0.000108155399+0.004459664773i, -0.000108272089+0.00445976564i, -0.000108311636+0.004459632693i, -0.000108327521+0.004459638584i, -0.000108324564+0.004459572353i, -0.00010831311+0.004459774997i, -0.000108311995+0.004459725754i, -0.000108350385+0.004459724478i, -0.000108428717+0.0044596322i, -0.000108429857+0.004459636626i, -0.000108423126+0.004459655452i, -0.00010850577+0.004459711378i, -0.000108570861+0.004459748404i, -0.000108510672+0.00445935589i, -0.000108526025+0.004459301618i, -0.000108608689+0.004459552659i, -0.000108615486+0.00445942612i, -0.000108701414+0.004459478426i, -0.000108675137+0.004459619875i, -0.000108712261+0.00445927603i, -0.000108682397+0.004459481247i, -0.00010872137+0.00445938387i, -0.000108745419+0.00445937139i, -0.000108777376+0.004459563901i, -0.000108806794+0.004459708027i, -0.000108827351+0.004459605103i, -0.00010883626+0.004459255684i, -0.00010887809+0.00445915523i, -0.000108885135+0.00445941035i, -0.000108926547+0.004459432845i, -0.000109020702+0.004459399286i, -0.000108996075+0.004459264456i, -0.000108937136+0.004459409088i, -0.000109058133+0.004459423571i, -0.000109094924+0.004459321935i, -0.000109107344+0.004459363481i, -0.000109269328+0.004459351709i, -0.000109102865+0.004459315152i, -0.000109234962+0.004459419544i, -0.00010919328+0.00445929508i, -0.000109250335+0.004459200264i, -0.000109250938+0.004459235905i, -0.000109295383+0.004459309423i, -0.000109413071+0.004459309893i, -0.000109412862+0.004459343943i, -0.000109388636+0.004459314042i, -0.000109460539+0.00445914097i, -0.000109511785+0.004459125046i, -0.000109458705+0.004459146057i, -0.000109552185+0.004459168236i, -0.00010961357+0.004459208353i, -0.000109620207+0.004459283282i, -0.000109668425+0.004459328985i, -0.000109701525+0.004459336273i, -0.000109712511+0.004459132032i, -0.000109773651+0.004459283643i, -0.000109883345+0.004459288118i, -0.000109779343+0.004459197241i, -0.000109830315+0.004459437888i, -0.000109829316+0.004459400711i, -0.000109966712+0.004459427786i, -0.00010998666+0.004459292413i, -0.000109927128+0.004459244373i, -0.000109986428+0.004459163913i, -0.00010999721+0.0044592906i, -0.000110085604+0.004459443972i, -0.000110200628+0.004459384501i, -0.000110160303+0.004459290422i, -0.000110197576+0.004459313938i, -0.000110247854+0.004459132415i, -0.00011027009+0.004459379492i, -0.000110232809+0.004459213476i, -0.000110359539+0.004459224827i, -0.000110356829+0.004459268906i, -0.00011036999+0.004459263271i, -0.000110433289+0.004459304098i, -0.000110442735+0.004459258678i, -0.000110529279+0.004459433155i, -0.000110539252+0.004459272989i, -0.000110525041+0.004459402945i, -0.000110612515+0.004459296776i, -0.000110583881+0.004459387793i, -0.000110653302+0.004459198785i, -0.000110629462+0.004459288594i, -0.000110661259+0.004459324906i, -0.000110711689+0.004459338806i, -0.000110802528+0.004459103224i, -0.000110784614+0.004459241622i, -0.000110825443+0.004459186547i, -0.000110817539+0.004459189134i, -0.0001108038+0.004459209559i, -0.000110879292+0.004459240535i, -0.000110934392+0.004459174628i, -0.000111001415+0.004459204554i, -0.000110968216+0.004459331595i, -0.000110966664+0.004459351729i, -0.000110952915+0.004459297962i, -0.000111022756+0.004459292989i, -0.000110987331+0.004459064685i, -0.000111020359+0.004459026105i, -0.000110997701+0.004459232308i, -0.000111093026+0.004459190094i, -0.000111191878+0.004459150401i, -0.000111146126+0.004459243361i, -0.00011126174+0.004459062552i, -0.000111304555+0.004459211081i, -0.000111169579+0.004459032962i, -0.000111341575+0.004459122937i, -0.000111203614+0.00445908606i, -0.00011135045+0.004459273745i, -0.000111281232+0.004459184065i, -0.000111361108+0.004459177915i, -0.000111414574+0.004459121104i, -0.000111417096+0.004459193837i, -0.00011146596+0.004458956017i, -0.000111427007+0.004459011913i, -0.000111524069+0.004458997206i, -0.000111490988+0.004459097924i, -0.000111577251+0.004459017011i, -0.00011162797+0.00445905501i, -0.000111659359+0.004459048126i, -0.000111565156+0.004458940913i, -0.000111600406+0.00445897255i, -0.000111675415+0.004459210377i, -0.000111728268+0.00445920608i, -0.00011175132+0.00445907224i, -0.000111925783+0.004459115427i, -0.000111825479+0.004459207328i, -0.000111889773+0.004459072662i, -0.000111952386+0.004458908109i, -0.000111968941+0.004459173977i, -0.000112025247+0.00445900599i, -0.000112082144+0.004459118423i, -0.000112105655+0.004459208274i, -0.000112165349+0.004459180661i, -0.00011216663+0.004459185313i, -0.000112200781+0.004459210835i, -0.000112249682+0.004459139774i, -0.000112186991+0.004459107982i, -0.000112368341+0.004459152169i, -0.000112285501+0.004459015632i, -0.000112391486+0.004459094248i, -0.000112484463+0.004459040877i, -0.000112473632+0.004459093077i, -0.000112487667+0.004459040387i, -0.000112610245+0.004459199559i, -0.000112566382+0.004459130889i, -0.00011264295+0.004459053346i, -0.000112578293+0.00445900893i, -0.00011271756+0.00445912549i, -0.000112762186+0.004459100269i, -0.000112742138+0.00445913886i, -0.000112804324+0.004459102291i, -0.000112736277+0.004459140265i, -0.000112925578+0.004459241615i, -0.000112789546+0.004459092814i, -0.000112899518+0.004459040289i, -0.000112919505+0.004459038191i, -0.000112951462+0.004459327233i, -0.00011291729+0.004459234908i, -0.000112961444+0.004459210761i, -0.000113024593+0.004459178607i, -0.00011302304+0.004459222064i, -0.000113060677+0.004459075416i, -0.000113099389+0.004459157006i, -0.0001130918+0.004458922082i, -0.000113112325+0.004458829559i, -0.000113188826+0.004458759156i, -0.000113224944+0.004458818431i, -0.000113182381+0.004458899716i, -0.000113081524+0.004458808639i, -0.000113181123+0.004458781875i, -0.000113135235+0.004458634678i, -0.000113205743+0.00445877963i, -0.00011330106399999999+0.00445884167i, -0.000113197714+0.004458684247i, -0.000113237973+0.00445884177i, -0.00011326865+0.004458846518i, -0.000113302317+0.004458844182i, -0.000113400902+0.0044587933i, -0.000113487744+0.004458749244i, -0.000113421006+0.004458879681i, -0.00011353638+0.004458733743i, -0.000113554038+0.004458772147i, -0.000113484955+0.004458753443i, -0.000113530443+0.004458669442i, -0.000113546348+0.00445866044i, -0.000113557573+0.00445871795i, -0.000113604396+0.004458666084i, -0.000113693333+0.004458730031i, -0.00011370289+0.004458786787i, -0.000113721655+0.004458606733i, -0.000113677232+0.004458798386i, -0.000113845364+0.004458853088i, -0.000113802006+0.00445880694i, -0.00011385273+0.004458781918i, -0.000113852244+0.004458804422i, -0.000113949005+0.004458706406i, -0.000113952351+0.00445870703i, -0.000113936357+0.004458772269i, -0.000114095036+0.00445881316i, -0.000114237175+0.004458843095i, -0.000114029463+0.004458764486i]
  out "Error Out":errorcluster
  in  "Error In":errorcluster
  in  "cursor bracket: fit boundaries":T8={"left"=991510.5808334925, "right "=1075639.2628144224, "center"=1033574.9218239575, "window"=84128.68198092999, "cursors"=[3, 4, 5], "relative"=0, "absolute"=0, "fixed vertical offset"=0.0, "vertical offset"=0.0, "skew"=0.0, "default window frac"=0.1, "kind"=enum."symmetric", "skew.left"=0.5, "skew.right"=0.5, "Plot ref"=refnum, "wing order"=enum."forw"}
  in  "scan monitor control":T9={"gamma acc. frac. - min "=0.3, "gamma acc frac.. - max"=3.0, "peak acc. fraction (af)"=5.0, "min peak acc. window (kHz)"=0.5, "use"=enum."fraction", "abs gamma min(kHz)"=0.005, "abs gamma max(kHz)"=5.0, "# points"=5, "gamma-factor (fa)"=3.0, "interpolate"=enum."line", "init"=TRUE, "Unique strike parameters"=TRUE, "max peak acc. window (kHz)"=10.0, "spacing factor"=1.5, "iterate #"=1, "overwrite ctl?"=FALSE, "write _m files?"=FALSE, "max slope (kHz/sweep)"=0.5, "funnel state"=enum."funnel open"}
  in  "Update system parameters":bool
  in  "parameters: complex fit":T10={"main VI path"=path "", "scale factor"=3.0, "# of grid points"=200, "parameters: wavepacket"={"R"=0.5, "wave number"=22.0, "delta k"=7.0, "radii vector"=[], "radial section"=[], "wave vector"=22.0, "wavepacket is"=TRUE}, "span"=0.27789, "interference ?"=enum."cp z center", "filter method"=enum."three"} {"span" min=0.0 max=0.5 step=1e-05 scale=0.0001..0.5 scale format="%#_5f"; "parameters: wavepacket"."delta k" format="%#_3f"; "parameters: wavepacket"."wave number" format="%#_3f"; "parameters: wavepacket"."R" format="%#_3f"}
  in  "cursor bracket: circle window":T8={"left"=1094842.7980648028, "right "=1109968.9974186728, "center"=1102405.8977417378, "window"=15126.199353870004, "cursors"=[0, 1, 2], "relative"=0, "absolute"=0, "fixed vertical offset"=0.0, "vertical offset"=0.0, "skew"=0.0, "default window frac"=0.1, "kind"=enum."symmetric", "skew.left"=0.5, "skew.right"=0.5, "Plot ref"=refnum, "wing order"=enum."forw"}
  in  "Tab : parameters":enum32{"Page 1"}(tab)
  out "VKey":T13=enum."Down"
  out "Char":i16
  # "three strikes"
  # "search window"
  # "linear extrapolation"
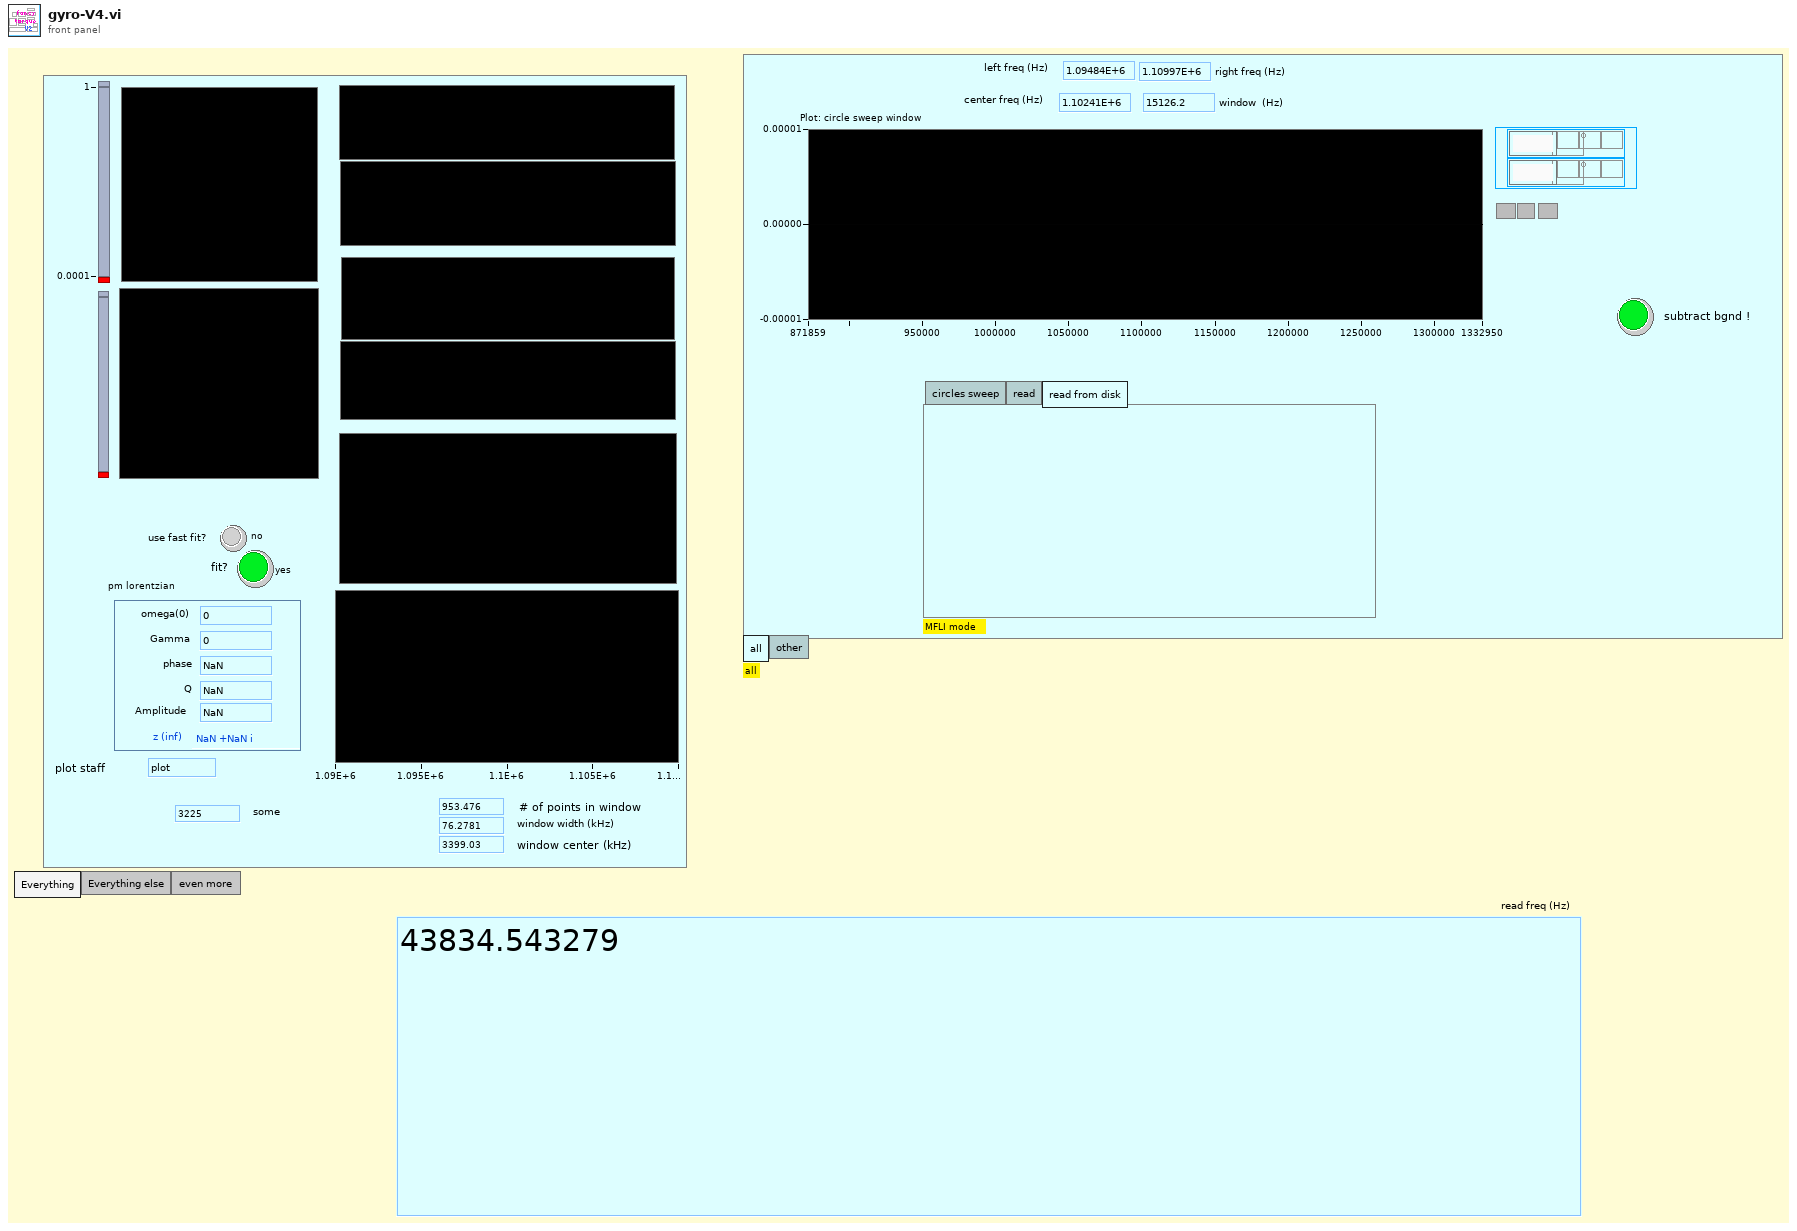
[diagram p1: front panel]
types:
  T1 = enum32{"circles sweep", "read", "read from disk", "circle PLL"}
  T2 = typedef "pid -- parameters.ctl" = cluster{"P (sec)":dbl, "I (sec)":dbl}
  T3 = typedef "agregator -- action.ctl" = enum16{"append", "interpolate", "empty!", "force", "init", "scale", "read last"}
  T4 = enum32{"Everything", "Everything else", "even more "}
  T5 = cluster{"omega out":dbl[], "win omega out":dbl[]}
  T6 = typedef "lorentzian.ctl" = cluster{"Amplitude":dbl, "omega(0)":dbl, "Gamma":dbl, "phase":dbl, "Q":dbl, "Norm  Ampl":dbl, "z (inf)":cdb, "4corners":T7}
  T7 = typedef "circle corners.ctl" = cluster{"z (-pi/2)":cdb, "z(inf)":cdb, "z (pi/2)":cdb, "z center":cdb, "z(0)":cdb, "radius":dbl}
  T8 = typedef "cursor winow.ctl" = cluster{"left":dbl, "right ":dbl, "center":dbl, "window":dbl, "cursors":i32[], "relative":i32, "absolute":i32, "fixed vertical offset":dbl, "vertical offset":dbl, "skew":dbl, "default window frac":dbl, "kind":enum16{"symmetric", "skewed", "fancy"}, "skew.left":dbl, "skew.right":dbl, "Plot ref":refnum<vi>, "wing order":enum16{"forw", "back"}}
  T9 = typedef "parameters -- scan monitor control.ctl" = cluster{"gamma acc. frac. - min ":dbl, "gamma acc frac.. - max":dbl, "peak acc. fraction (af)":dbl, "min peak acc. window (kHz)":dbl, "use":enum16{"window", "fraction"}, "abs gamma min(kHz)":dbl, "abs gamma max(kHz)":dbl, "# points":i32, "gamma-factor (fa)":dbl, "interpolate":enum16{"line", "last"}, "init":bool, "Unique strike parameters":bool, "max peak acc. window (kHz)":dbl, "spacing factor":dbl, "iterate #":i32, "overwrite ctl?":bool, "write _m files?":bool, "max slope (kHz/sweep)":dbl, "funnel state":enum16{"funnel open", "funnel closed"}}
  T10 = typedef "peak -- parameters -- complex fit.ctl" = cluster{"main VI path":path, "scale factor":dbl, "# of grid points":i32, "parameters: wavepacket":T11, "span":dbl, "interference ?":enum16{"cp z center", "pm zcenter", "fancy"}, "filter method":T12}
  T11 = typedef "wavepacket.ctl" = cluster{"R":dbl, "wave number":dbl, "delta k":dbl, "radii vector":dbl[], "radial section":cdb[], "wave vector":dbl, "wavepacket is":bool}
  T12 = typedef "filter method control.ctl" = enum16{"four", "five", "one", "two", "three", "zero", "minus one", "minus two"}
  T13 = typedef "eventvkey.ctl" = enum16{"ASCII", "Enter", "Return", "Shift", "Ctrl", "Alt", "Cmd", "Opt", "Caps", "NumLock", "Clear", "Break", "Up", "Down", "Left", "Right", "Insert", "Delete", "Home", "End", "PageUp", "PageDown", "Escape", "Help", "Pause", "ScrollLock", "F1", "F2", "F3", "F4", "F5", "F6", "F7", "F8", "F9", "F10", "F11", "F12", "F13", "F14", "F15", "F16", "F17", "F18", "F19", "F20", "F21", "F22", "F23", "F24", "Play", "VolumeUp", "VolumeDown", "Mute", "Two Byte Char"}
  T14 = typedef "MFLI controller action.ctl" = enum16{"Initialize", "Scan frequency", "open", "close", "read", "circle PLL"}
  T15 = typedef "cursor window action.ctl" = enum16{"balance", "h. offset change", "cursor moves", "change center", "change window", "init", "check", "reset", "set y to middle", "idle", "-write all Y", "-write left.X", "-write center.X", "-write right.X", "-write all X", "-change center", "-change window", "-change skew", "-read cursor 2", "-read cursor 1", "-read cursor 0", "-read all cursors", "-reset", "-read plot scale", "-set y to middle", "-Q: center.Y is visible", "-Q: window is visible", "-parse center.Y", "-right left from center", "-left move", "-right move", "-set center.Y", "-empty", "-set cursors to default", "-check", "-write center.Y", "-copy cursor 1", "-copy cursor 0", "-copy cursor 2", "move right", "move left", "shrink", "broaden", "skew up", "skew down", "-write plot scale", "zoom X", "change cen&win", "zoom to all data", "color--red", "color--green", "color--yellow", "read", "zoom out", "zoom in", "slide right", "slide left"}
  T16 = typedef "plot refs -- filter related.ctl" = cluster{"Plot: complex plane - filter":refnum<vi>, "Plot: dz/domega":refnum<vi>, "Plot: fragment filter":refnum<vi>, "Plot: win omega":refnum<vi>, "Plot: phase":refnum<vi>, "Plot: phase around center":refnum<vi>, "Plot: complex plane":refnum<vi>, "Plot: fragment":refnum<vi>}
  T17 = typedef "publisher action.ctl" = enum16{"set", "get"}
  T18 = typedef "file -- read-write control.ctl" = enum16{"read", "write all", "append one line"}
  T19 = typedef "sweep parameters.ctl" = cluster{"scan type":enum16{"linear", "arctan"}, "N":i64, "cursor window":T8}
  T20 = typedef "cursor action.ctl" = enum16{"range", "read", "write", "check", "zoom out", "smart zoom out"}
  T21 = typedef "KM_file -- read-write control.ctl" = enum16{"read", "write all", "append one line"}
  T22 = typedef "filename-action.ctl" = enum16{"rewrite", "parse"}
  T23 = typedef "four-corner circle transformation.ctl" = enum16{"z(c) z(inf)", "z(c) z(zero)", "fix phase", "calculate lorentzian", "z(0) z(+-pi/2)", "shift to zcenter", "to  canonical", "get canonical phase", "get4corners"}
  T24 = typedef "interpolation state - real.ctl" = cluster{"requested size":i32, "Array":dbl[], "actual number of elements":i32}
  T25 = typedef "interpolation state - complex.ctl" = cluster{"requested size":i32, "Array":cdb[], "actual number of elements":i32}
  T26 = enum16{"frequency", "gamma", "phase", "background"}
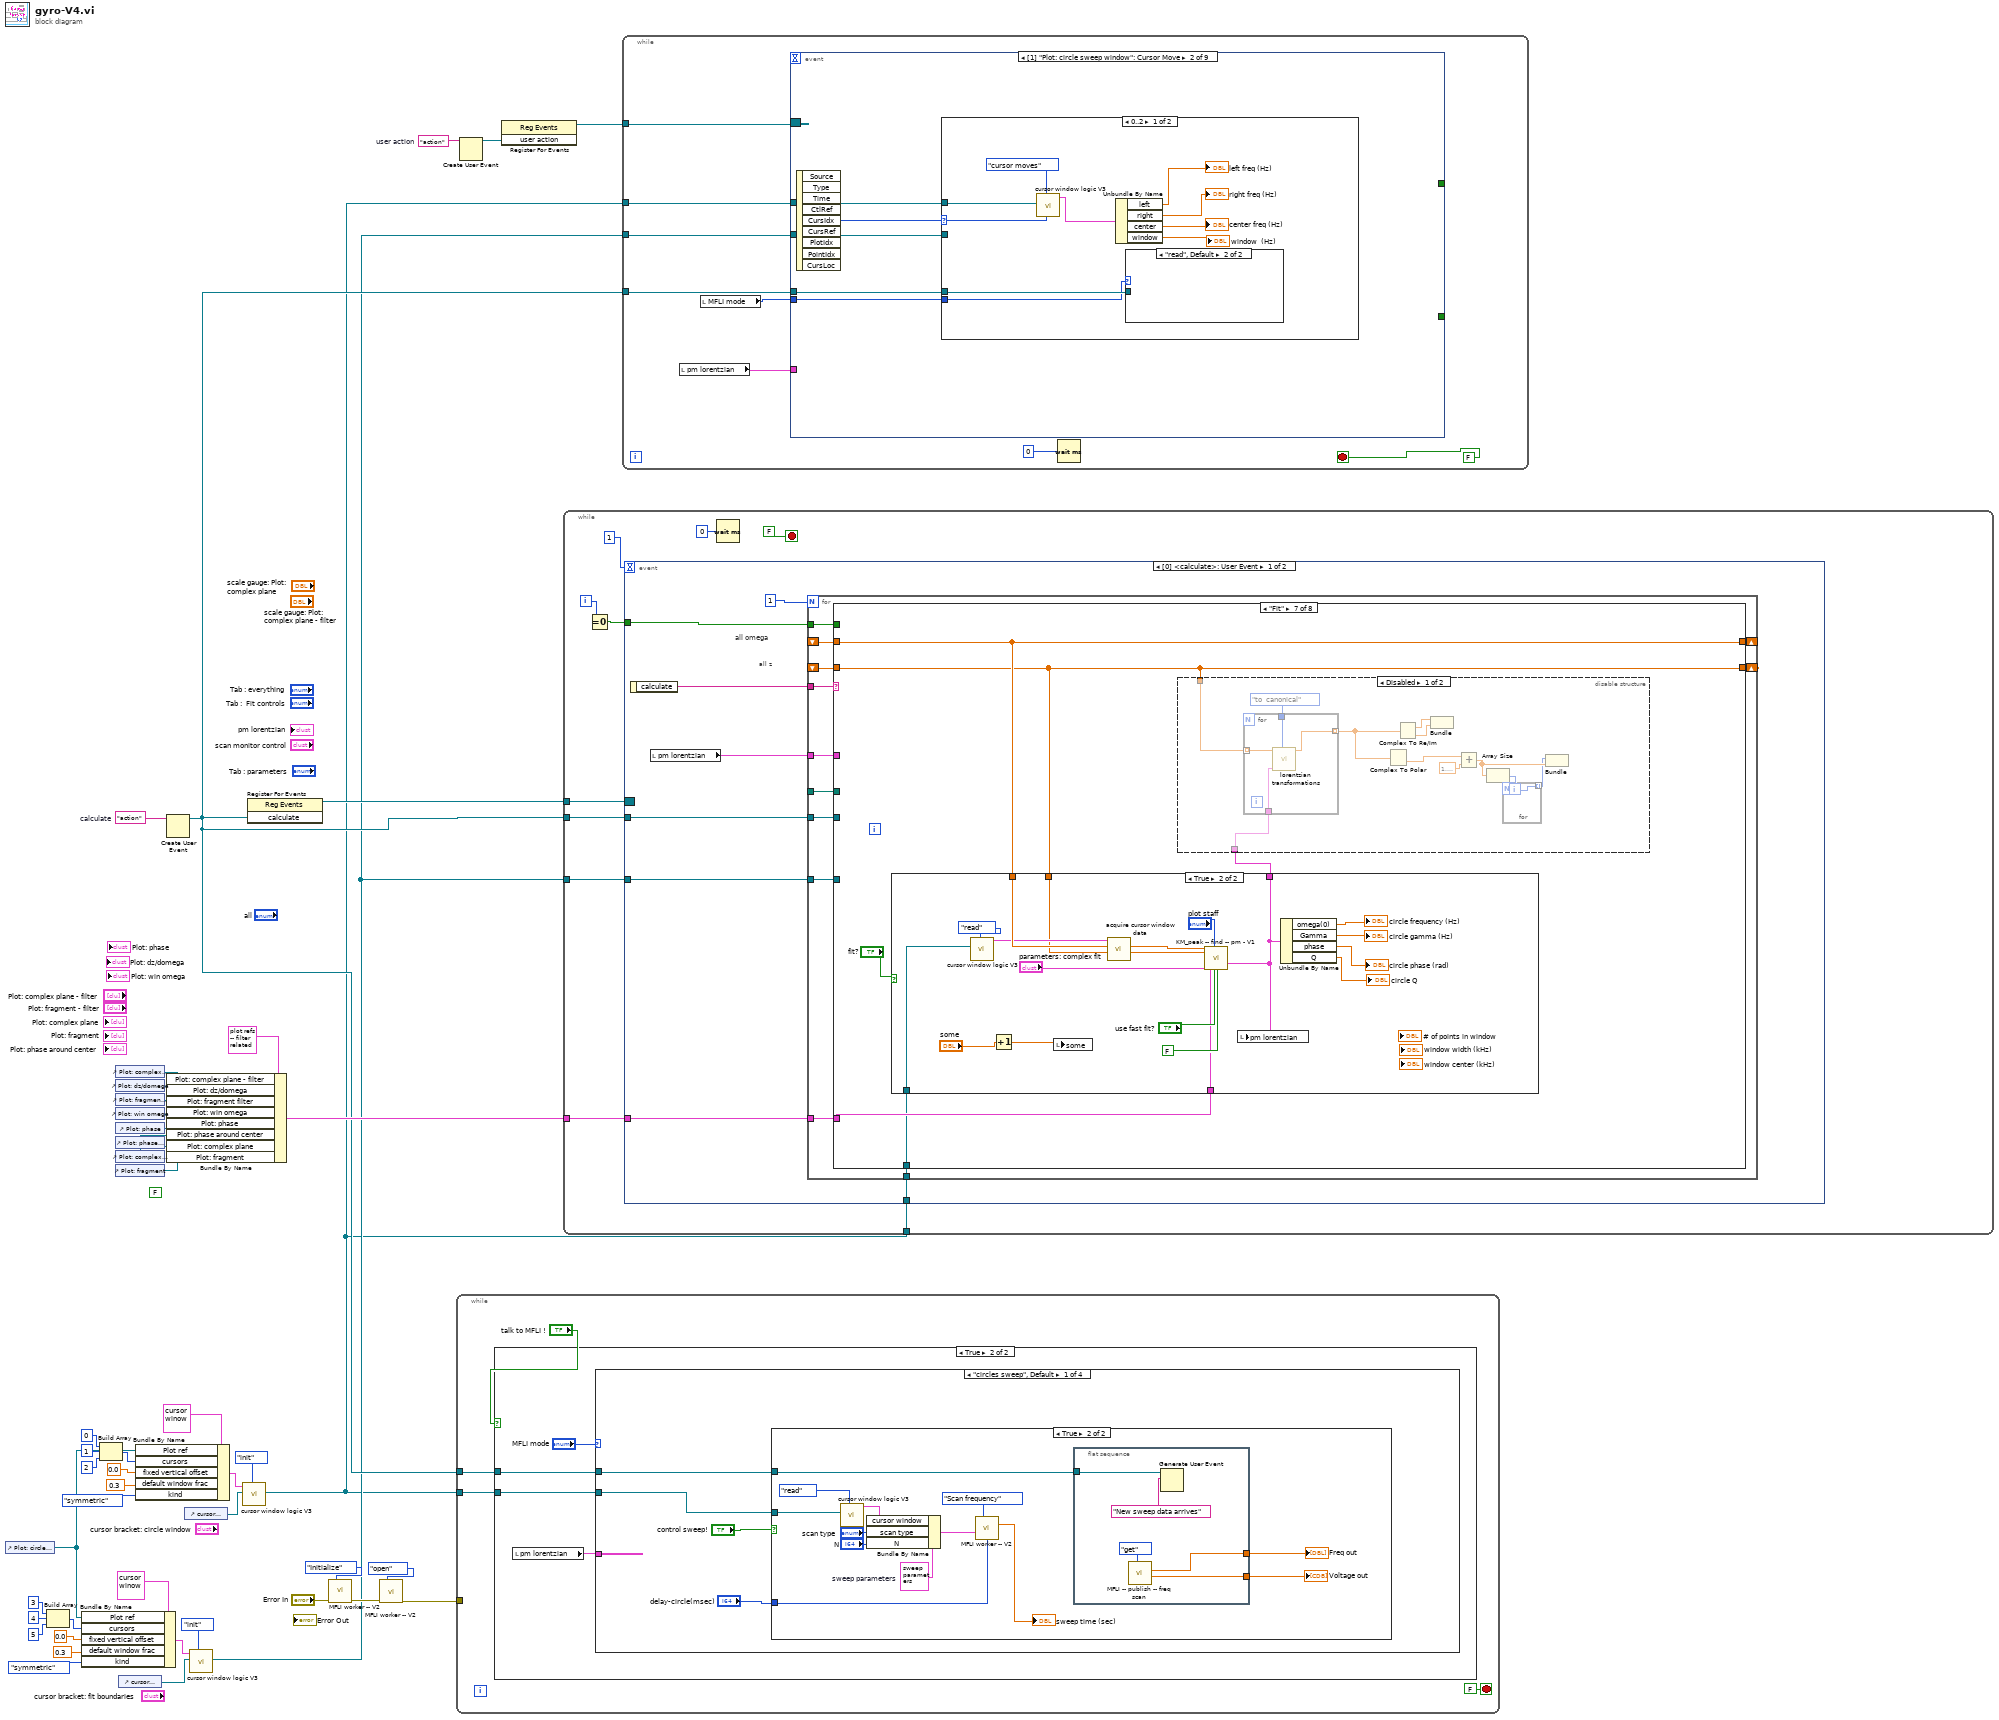
[diagram p0: block diagram]
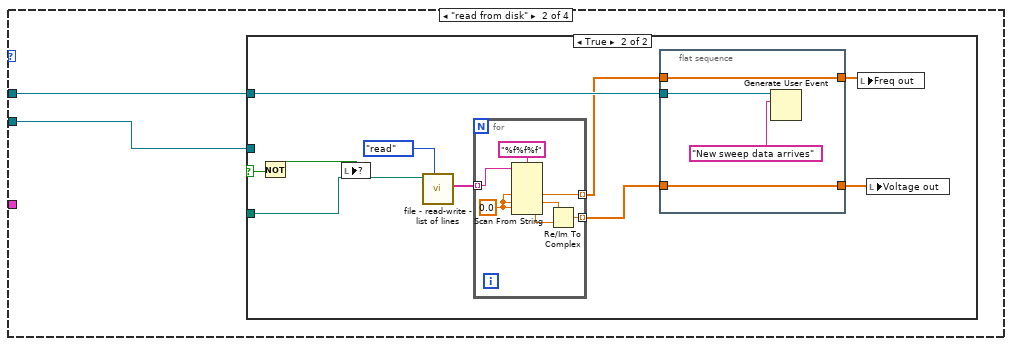
[diagram p4: hidden frame]
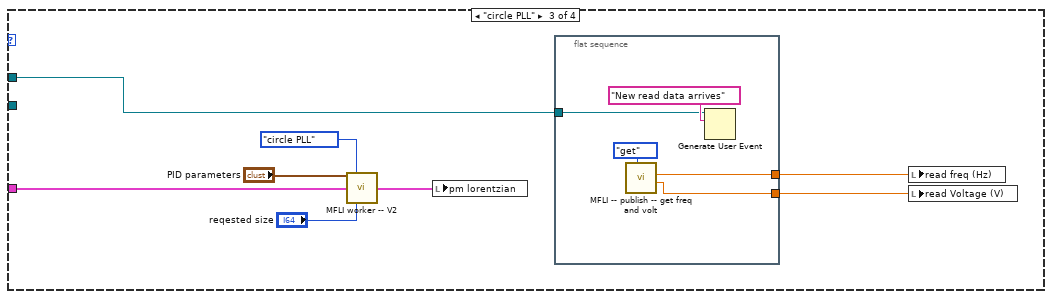
[diagram p6: hidden frame]
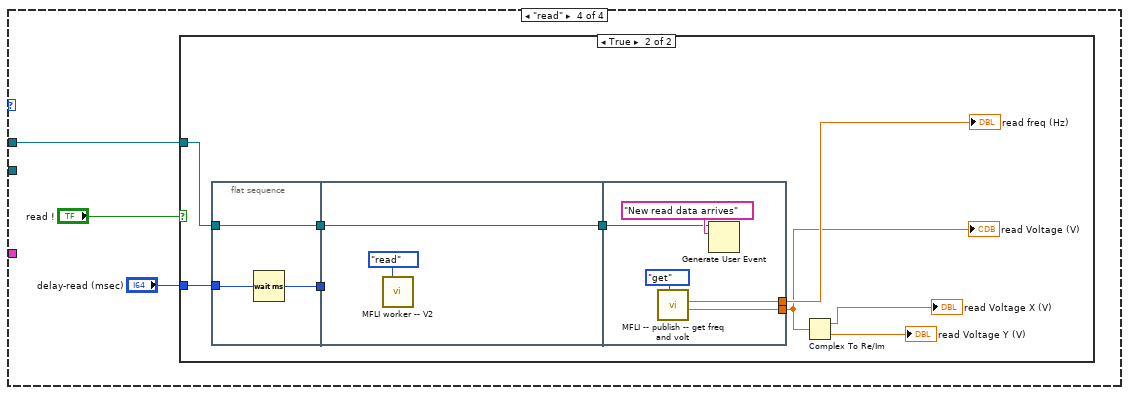
[diagram p7: hidden frame]
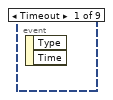
[diagram p9: hidden frame]
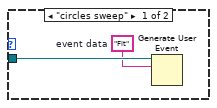
[diagram p10: hidden frame]
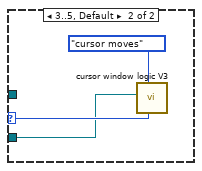
[diagram p11: hidden frame]
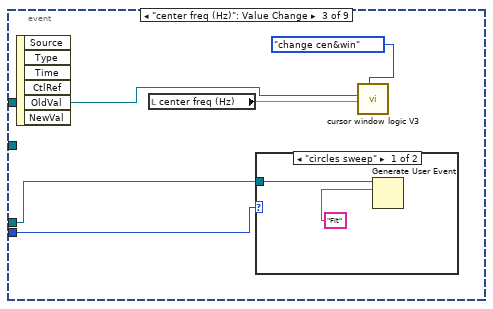
[diagram p12: hidden frame]
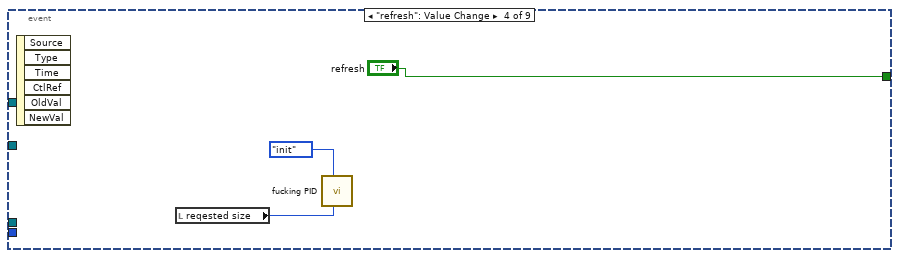
[diagram p14: hidden frame]
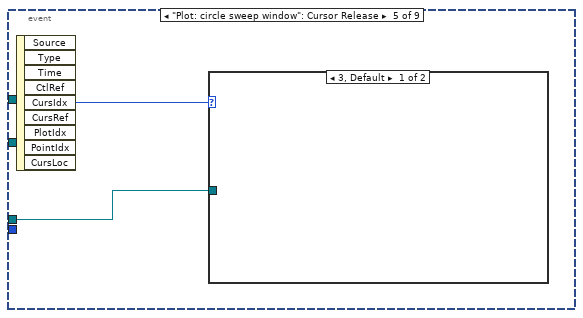
[diagram p15: hidden frame]
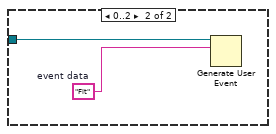
[diagram p16: hidden frame]
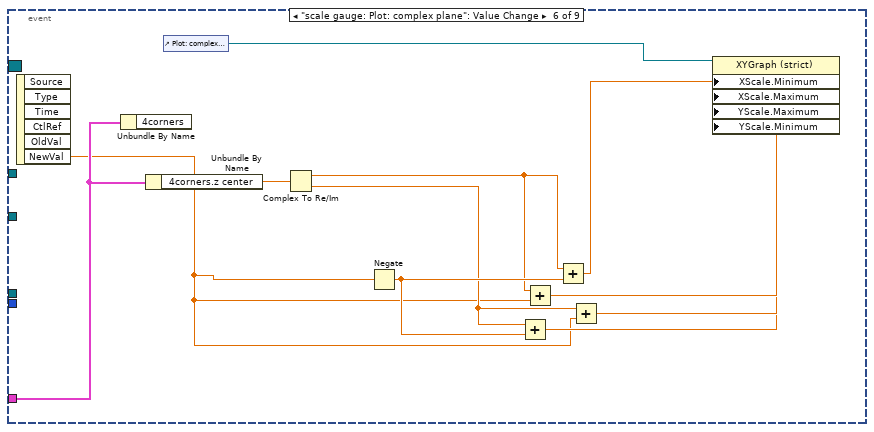
[diagram p17: hidden frame]
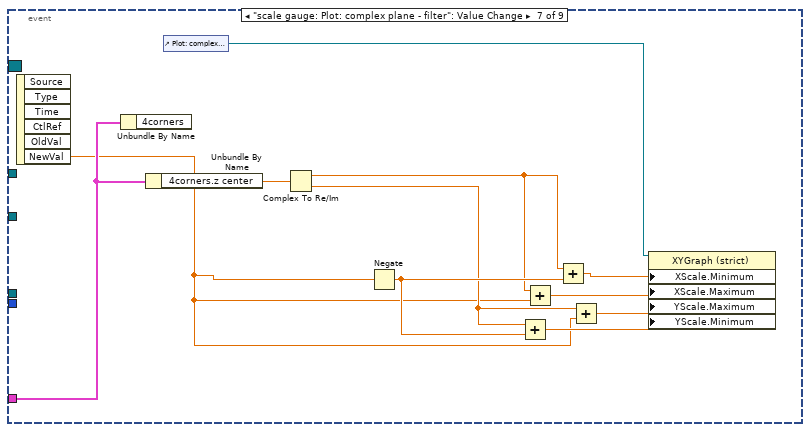
[diagram p18: hidden frame]
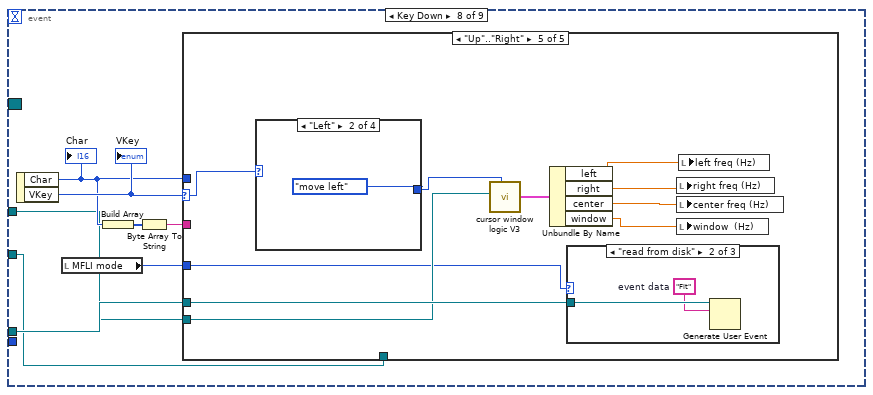
[diagram p19: hidden frame]
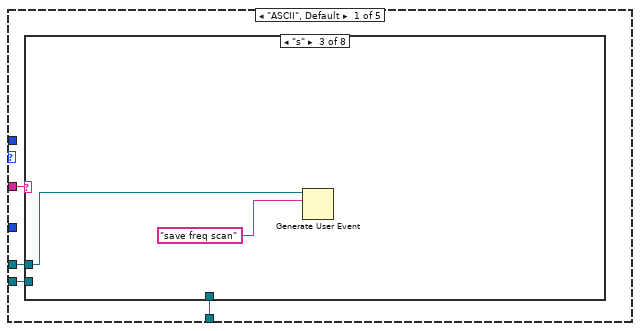
[diagram p20: hidden frame]
diagram:
  w43 = "action"  # user action
  w45 = "action"  # calculate
  (unwired) FALSE
  n1 = control-ref of="Plot: circle sweep window"() -> (w6:refnum<vi>)
  n2 = Build Array(3, 4, 5) -> (w17:i32[])
  n3 = Bundle By Name(cluster=T8 {"left"=0.0, "right "=0.0, "center"=0.0, "window"=0.0, "cursors"=[], "relative"=0, "absolute"=0, "fixed vertical offset"=0.0, "vertical offset"=0.0, "skew"=0.0, "default window frac"=0.0, "kind"=enum."symmetric", "skew.left"=0.0, "skew.right"=0.0, "Plot ref"=refnum, "wing order"=enum."forw"} ("cursor bracket: All, data window"), "Plot ref"=w6, "cursors"=w17, "fixed vertical offset"=0.0, "default window frac"=0.3 ("fixed vertical offset"), "kind"=enum16{"symmetric", "skewed", "fancy"}."symmetric") -> (w9:T8)
  n4 = Build Array(0, 1, 2) -> (w30:i32[])
  n5 = control-ref of="Plot: complex plane - filter"() -> (w40:refnum<vi>)
  n6 = control-ref of="Plot: dz/domega"() -> (w39:refnum<vi>)
  n7 = control-ref of="Plot: fragment - filter"() -> (w38:refnum<vi>)
  n8 = control-ref of="Plot: win omega"() -> (w37:refnum<vi>)
  n9 = control-ref of="Plot: phase"() -> (w36:refnum<vi>)
  n10 = control-ref of="Plot: phase around center"() -> (w34:refnum<vi>)
  n11 = control-ref of="Plot: complex plane"() -> (w33:refnum<vi>)
  n12 = control-ref of="Plot: fragment"() -> (w32:refnum<vi>)
  n13 = control-ref of="cursor bracket: fit boundaries"() -> (w7:refnum<vi>)
  n14 = Bundle By Name(cluster=T8 {"left"=0.0, "right "=0.0, "center"=0.0, "window"=0.0, "cursors"=[], "relative"=0, "absolute"=0, "fixed vertical offset"=0.0, "vertical offset"=0.0, "skew"=0.0, "default window frac"=0.0, "kind"=enum."symmetric", "skew.left"=0.0, "skew.right"=0.0, "Plot ref"=refnum, "wing order"=enum."forw"} ("cursor bracket: All, data window"), "Plot ref"=w6, "cursors"=w30, "fixed vertical offset"=0.0, "default window frac"=0.3 ("fixed vertical offset"), "kind"=enum16{"symmetric", "skewed", "fancy"}."symmetric") -> (w22:T8)
  n15 = Bundle By Name(cluster=T16 {"Plot: complex plane - filter"=refnum, "Plot: dz/domega"=refnum, "Plot: fragment filter"=refnum, "Plot: win omega"=refnum, "Plot: phase"=refnum, "Plot: phase around center"=refnum, "Plot: complex plane"=refnum, "Plot: fragment"=refnum} ("plots: filter related"), "Plot: complex plane - filter"=w40, "Plot: dz/domega"=w39, "Plot: fragment filter"=w38, "Plot: win omega"=w37, "Plot: phase"=w36, "Plot: phase around center"=w34, "Plot: complex plane"=w33, "Plot: fragment"=w32) -> (w35:T16)
  n16 = Create User Event(user event datatype=w45) -> (user event=w31:refnum<user-event>)  [unwired: 1 in, 1 out]
  n17 = control-ref of="cursor bracket: circle window"() -> (w21:refnum<vi>)
  n18 = call "cursor window logic V3.vi"("cursor window action"=cursor_window_action."init", "cursor window in"=w7, "cursor window init"=w9) -> ("cursor window out"=w2:refnum<vi>)  [unwired: 7 in, 1 out]
  n19 = call "cursor window logic V3.vi"("cursor window action"=cursor_window_action."init", "cursor window in"=w21, "cursor window init"=w22) -> ("cursor window out"=w1:refnum<vi>)  [unwired: 7 in, 1 out]
  n20 = register-events(w31) -> (reference out=w46:refnum<event-registration>)  [unwired: 2 in, 1 out]
  n21 = call "MFLI worker -- V2.vi"("MFLI controller action"=MFLI_controller_action."Initialize", "Error In"="Error In") -> ("Error Out"=w4:errorcluster)  [unwired: 11 in, 2 out]
  n22 = call "MFLI worker -- V2.vi"("MFLI controller action"=MFLI_controller_action."open", "Error In"=w4) -> ("Error Out"=w3:errorcluster)  [unwired: 11 in, 2 out]
  n23 = while {
    tunnel: w31 -> [w50]
    tunnel: w1 -> [w48]
    tunnel: w3 -> [_]
    stop <- FALSE stop-if-true
    n24 = case shown="True" "talk to MFLI !" {
      tunnel: w50 -> [_ w54]
      tunnel: w48 -> [_ w53]
      frame False {
      }
      frame True {
        n25 = local read "pm lorentzian"() -> (w51:T6)
        n26 = case shown="\"circles sweep\", Default" "MFLI mode" {
          tunnel: w54 -> [w58 w80 w106 w117]
          tunnel: w53 -> [w57 w79 _ _]
          tunnel: w51 -> [_ _ w108 _]
          frame "circles sweep", Default {
            n27 = case shown="True" "control sweep!" {
              tunnel: w58 -> [_ w71]
              tunnel: w57 -> [_ w70]
              tunnel: "delay-circle(msec)" -> [_ w62]
              frame False {
              }
              frame True {
                w67 = T19 {"scan type"=enum."linear", "N"=-1, "cursor window"={"left"=2378.60310421286, "right "=2421.6740576496672, "center"=2421.6740576496672, "window"=2421.6740576496672, "cursors"=[], "relative"=0, "absolute"=0, "fixed vertical offset"=2421.6740576496672, "vertical offset"=2421.6740576496672, "skew"=2421.6740576496672, "default window frac"=2421.6740576496672, "kind"=enum."skewed", "skew.left"=2421.6740576496672, "skew.right"=2421.6740576496672, "Plot ref"=refnum, "wing order"=enum."back"}}  # sweep parameters
                n28 = call "cursor window logic V3.vi"("cursor window action"=cursor_window_action."read", "cursor window in"=w70) -> ("cursor window out"=w65:T8)  [unwired: 8 in, 1 out]
                n29 = Bundle By Name(cluster=w67, "cursor window"=w65, "scan type"="scan type", "N"="N") -> (w63:T19)
                n30 = call "MFLI worker -- V2.vi"("MFLI controller action"=MFLI_controller_action."Scan frequency", "sweep parameters"=w63, "delay (msec)"=w62) -> ("sweep time"=→"sweep time (sec)":dbl)  [unwired: 10 in, 2 out]
                n31 = flat-sequence {
                  tunnel: w71 -> [w75]
                  tunnel: [w73] -> w61
                  tunnel: [w72] -> w60
                  frame #0 {
                    n32 = call "MFLI -- publish -- freq scan.vi"("publisher action"=publisher_action."get") -> ("Voltage out (V)"=w73:cdb[], "Freq out (Hz)"=w72:dbl[])  [unwired: 9 in]
                    n33 = Generate User Event(user event=w75, event data cluster="New sweep data arrives" ("event data")) -> ()  [unwired: 2 in, 2 out]
                  }
                }
                "Freq out" <- w60
                "Voltage out" <- w61
              }
            }
          }
          frame "read from disk" {
            n34 = case shown="True" w78 {
              selector: [_ w89] -> w78
              tunnel: w80 -> [_ w90]
              tunnel: w79 -> [_ _]
              tunnel: [_ w86] -> w77
              frame False {
              }
              frame True {
                n35 = Not(x=w89) -> (.not. x?=w88:bool)
                n36 = local write item#-1(w88) -> ()
                n37 = call "file - read-write - list of lines.vi"("read/write control"=file_--_read-write_control."read", "file path"=w86) -> ("list of lines OUT"=w85:string[])  [unwired: 8 in, 1 out]
                n38 = for {
                  tunnel: w85 -> [w97] mode=indexing
                  tunnel: [w95] -> w84 mode=indexing
                  tunnel: [w92] -> w81 mode=indexing
                  w91 = 0.0
                  n39 = Scan From String(format string="%f%f%f", input string=w97, default 1=w91, default 2=w91, default 3=w91) -> (output 1=w95:dbl, output 2=w94:dbl, output 3=w93:dbl)  [unwired: 2 in, 3 out]
                  n40 = Re/Im To Complex(1:w93, 2:w94) -> (0:w92:cdb)
                }
                n41 = flat-sequence {
                  tunnel: w84 -> [w101]
                  tunnel: [w101] -> w83
                  tunnel: w90 -> [w100]
                  tunnel: [w99] -> w82
                  tunnel: w81 -> [w99]
                  frame #0 {
                    n42 = Generate User Event(user event=w100, event data cluster="New sweep data arrives" ("event data")) -> ()  [unwired: 2 in, 2 out]
                  }
                }
                n43 = local write "Freq out"(w83) -> ()
                n44 = local write "Voltage out"(w82) -> ()
              }
            }
          }
          frame "circle PLL" {
            n45 = call "MFLI worker -- V2.vi"("PID parameters"="PID parameters", "MFLI controller action"=MFLI_controller_action."circle PLL", "lorentzian in"=w108, "reqested size"="reqested size") -> ("lorentzian out"=w103:T6)  [unwired: 9 in, 2 out]
            n46 = local write "pm lorentzian"(w103) -> ()
            n47 = flat-sequence {
              tunnel: w106 -> [w113]
              tunnel: [w110] -> w105
              tunnel: [w111] -> w104
              frame #0 {
                n48 = call "MFLI -- publish -- get freq and volt.vi"("publisher action"=publisher_action."get") -> ("Voltage out (V)"=w111:cdb, "freq out (Hz)"=w110:dbl)  [unwired: 9 in]
                n49 = Generate User Event(user event=w113, event data cluster="New read data arrives" ("event data")) -> ()  [unwired: 2 in, 2 out]
              }
            }
            n50 = local write "read freq (Hz)"(w105) -> ()
            n51 = local write "read Voltage (V)"(w104) -> ()
          }
          frame "read" {
            n52 = case shown="True" "read !" {
              tunnel: w117 -> [_ w126]
              tunnel: "delay-read (msec)" -> [_ w123]
              frame False {
              }
              frame True {
                n53 = flat-sequence {
                  tunnel: w126 -> [w129]
                  tunnel: [w129] -> w124
                  tunnel: w123 -> [w128]
                  tunnel: [w127] -> w122
                  tunnel: [w131] -> w125
                  tunnel: w124 -> [w131]
                  tunnel: w122 -> [_]
                  tunnel: w125 -> [w135]
                  tunnel: [w133] -> w119
                  tunnel: [w132] -> w118
                  frame #0 {
                    n54 = Wait (ms)(milliseconds to wait=w128) -> (millisecond timer value=w127:u32)
                  }
                  frame #1 {
                    n55 = call "MFLI worker -- V2.vi"("MFLI controller action"=MFLI_controller_action."read") -> ()  [unwired: 12 in, 3 out]
                  }
                  frame #2 {
                    n56 = call "MFLI -- publish -- get freq and volt.vi"("publisher action"=publisher_action."get") -> ("Voltage out (V)"=w132:cdb, "freq out (Hz)"=w133:dbl)  [unwired: 9 in]
                    n57 = Generate User Event(user event=w135, event data cluster="New read data arrives" ("event data")) -> ()  [unwired: 2 in, 2 out]
                  }
                }
                n58 = Complex To Re/Im(x + iy=w118) -> (x=→"read Voltage X (V)":dbl, y=→"read Voltage Y (V)":dbl)
                "read freq (Hz)" <- w119
                "read Voltage (V)" <- w118
              }
            }
          }
        }
      }
    }
  }
  n59 = Create User Event(user event datatype=w43) -> (user event=w42:refnum<user-event>)  [unwired: 1 in, 1 out]
  n60 = register-events(w42) -> (reference out=w44:refnum<event-registration>)  [unwired: 2 in, 1 out]
  n61 = while {
    tunnel: w46 -> [w146]
    tunnel: w31 -> [w144]
    tunnel: w35 -> [w140]
    tunnel: w1 -> [w138]
    tunnel: w2 -> [w137]
    i -> [w141]
    stop <- FALSE stop-if-true
    n62 = Equal To 0?(x=w141) -> (x = 0?=w139:bool)
    n63 = event shown="[0] <calculate>: User Event" {
      selector: w146 -> [_ _]
      dyn-events: _ -> [_ _]
      timeout: 1 -> [_ _]
      tunnel: w144 -> [w154 _]
      tunnel: w140 -> [w151 _]
      tunnel: w139 -> [w150 _]
      tunnel: w138 -> [w149 _]
      tunnel: w137 -> [w147 _]
      event User Event {
        # "all z"
        # "all omega"
        n64 = event-data() -> ("calculate"=w155:string)  [unwired: 1 in]
        n65 = local read "pm lorentzian"() -> (w148:T6)
        n66 = for {
          N: 1 -> [_]
          tunnel: w155 -> [w167]
          tunnel: w154 -> [w166]
          shift-right: [w160] -> _
          shift-left: _ -> [w165]
          shift-right: [w159] -> _
          shift-left: _ -> [w164]
          tunnel: [w163] -> w152
          tunnel: w151 -> [w162]
          tunnel: w150 -> [w161]
          tunnel: w149 -> [w158]
          tunnel: w148 -> [w157]
          tunnel: w147 -> [w156]
          n67 = case shown="\"Fit\"" w167 {
            tunnel: w166 -> [w181 w235 _ _ _ _ _ _]
            tunnel: w165 -> [_ w234 w293 w312 w318 w340 w362 w403]
            tunnel: w164 -> [_ w233 w292 w311 w317 w339 w361 w402]
            tunnel: w163 -> [_ _ _ w307 w319 w337 _ _]
            tunnel: w162 -> [_ _ _ _ _ _ w364 _]
            tunnel: w161 -> [_ _ _ _ _ _ _ _]
            tunnel: [w172 w234 w293 w312 w318 w340 w362 w403] -> w160
            tunnel: [w170 w233 w292 w311 w317 w339 w361 w402] -> w159
            tunnel: w158 -> [_ _ _ _ _ w338 w363 _]
            tunnel: w157 -> [_ _ w279 w306 _ w336 _ _]
            tunnel: w156 -> [_ w232 _ _ _ w329 _ _]
            frame "New sweep data arrives" {
              n68 = local read "Voltage out"() -> (w171:cdb[])
              n69 = local read "Freq out"() -> (w173:dbl[])
              n70 = case shown="False" "subtract bgnd !" {
                tunnel: w173 -> [w193 w201]
                tunnel: [w187 w201] -> w172
                tunnel: w171 -> [w189 w200]
                tunnel: [w194 w200] -> w170
                frame True {
                  w186 = 10 ("length")
                  n71 = Delete From Array(array=w189, length=w186, index=0) -> (array with subset deleted=w188:cdb[])  [unwired: 1 out]
                  n72 = Delete From Array(array=w193, length=w186, index=0) -> (array with subset deleted=w192:dbl[])  [unwired: 1 out]
                  n73 = call "linear interp iiii- complex - z-omega.vi"("z"=w188, "omega"=w192) -> ("z out"=w195:cdb[], "omega out"=w187:dbl[], "intercept"=w197:cdb, "slope"=w198:cdb)  [unwired: 5 in, 5 out]
                  n74 = Multiply(x=w187, y=w198) -> (x*y=w199:cdb[])
                  n75 = Add(x=w199, y=w197) -> (x+y=w196:cdb[])
                  n76 = Subtract(x=w195, y=w196) -> (x-y=w194:cdb[])
                }
                frame False {
                }
              }
              n77 = Generate User Event(user event=w181, event data cluster="Fit" ("event data")) -> (user event out=w179:refnum<user-event>)  [unwired: 2 in, 1 out]
              n78 = case shown="True" "Auto-update sweep window!" {
                tunnel: w179 -> [w204 w206]
                tunnel: [w204 w205] -> w178
                frame False {
                }
                frame True {
                  n79 = Generate User Event(user event=w206, event data cluster="Update range" ("event data")) -> (user event out=w205:refnum<user-event>)  [unwired: 2 in, 1 out]
                }
              }
              n80 = Complex To Re/Im(x + iy=w170) -> (x=w184:dbl[], y=w183:dbl[])
              n81 = case shown="True" w180 {
                tunnel: w178 -> [w208 w210]
                tunnel: [w208 w209] -> w175
                frame False {
                }
                frame True {
                  n82 = Generate User Event(user event=w210, event data cluster="Plot frequency shift" ("event data")) -> (user event out=w209:refnum<user-event>)  [unwired: 2 in, 1 out]
                }
              }
              n83 = Bundle("Freq out"=w172, w184) -> (w185:cluster{"Freq out":dbl[], dbl[]})  [unwired: 1 in]
              n84 = Bundle("Freq out"=w172, w183) -> (w182:cluster{"Freq out":dbl[], dbl[]})  [unwired: 1 in]
              n85 = case shown="True" w176 {
                tunnel: w175 -> [_ w202]
                frame False {
                }
                frame True {
                  n86 = Generate User Event(user event=w202, event data cluster="save data" ("event data")) -> ()  [unwired: 2 in, 2 out]
                }
              }
              n87 = Build Array(w185, w182) -> (→"Plot: circle sweep window":cluster{"Freq out":dbl[], dbl[]}[])
            }
            frame "New read data arrives" {
              n88 = local read "read freq (Hz)"() -> (w212:dbl)
              n89 = local read "read Voltage (V)"() -> (w217:cdb)
              n90 = call "cursor window logic V3.vi"("cursor window action"=cursor_window_action."read", "cursor window in"=w232) -> ("cursor window out"=w230:T8)  [unwired: 8 in, 1 out]
              n91 = local read "pm lorentzian"() -> (w215:T6)
              n92 = Unbundle By Name(w230) -> ("Plot ref"=w229:refnum<vi>)
              n93 = Bundle By Name(cluster=w215, "omega(0)"=w212) -> (w214:T6)
              n94 = call "replace cursor - plot ref - V2.vi"("Plot ref in"=w229, "new X"=w212, "cursor index"=6, "cursor action"=cursor_action."write") -> ()  [unwired: 13 in, 3 out]
              n95 = local read item#-1() -> (w236)
              n96 = for {
                N: 1 -> [_]
                shift-right: [w252] -> w226
                shift-left: _ -> [w251]
                tunnel: w217 -> [w250]
                tunnel: w212 -> [w249]
                shift-right: [w247] -> w224
                shift-left: _ -> [w248]
                tunnel: "aggregator action" -> [w245]
                w246 = 10000
                n97 = call "aggregator - vii - real - atomic.vi"("aggregator action"=w245, "requested size"=w246, "number"=w249, "state IN"=w248) -> ("state OUT"=w247:T24)  [unwired: 4 in, 3 out]
                n98 = call "aggregator - vii - complex - atomic.vi"("aggregator action"=w245, "requested size"=w246, "number"=w250, "state IN"=w251) -> ("state OUT"=w252:T25)  [unwired: 4 in, 3 out]
              }
              n99 = case shown="True" w236 {
                tunnel: w235 -> [w255 w257]
                tunnel: [w255 w256] -> w238
                frame False {
                }
                frame True {
                  n100 = Generate User Event(user event=w257, event data cluster="Plot frequency shift" ("event data")) -> (user event out=w256:refnum<user-event>)  [unwired: 2 in, 1 out]
                }
              }
              n101 = local write "pm lorentzian"(w214) -> ()
              n102 = Unbundle By Name(w224) -> ("Array"=w222:dbl[])
              n103 = Unbundle By Name(w226) -> ("Array"=w220:cdb[])
              n104 = local read item#-1() -> (w237)
              n105 = Complex To Re/Im(x + iy=w220) -> (x=w219:dbl[], y=w218:dbl[])
              n106 = Bundle(w219, w218) -> ()  [unwired: 1 in, 1 out]
              n107 = Array Size(array=w222) -> (size(s)=w223:i32)
              n108 = case shown="True" w237 {
                tunnel: w238 -> [_ w253]
                frame False {
                }
                frame True {
                  n109 = Generate User Event(user event=w253, event data cluster="save data" ("event data")) -> ()  [unwired: 2 in, 2 out]
                }
              }
              n110 = for {
                N: w223 -> [_]
                tunnel: [w244] -> w221 mode=indexing
                i -> [w244]
              }
              n111 = Bundle(w221, "Array"=w222) -> ()  [unwired: 1 in, 1 out]
              n112 = case shown="\"save\", Default" w213 {
                tunnel: w212 -> [w243 _]
                frame "save", Default {
                  n113 = call "KM_appendline --readfreq.vi"("freq"=w243, "append to file? (new file:F)"=FALSE, "read/write control"=KM_file_--_read-write_control."append one line") -> ("Save frequency scan"=w240:path, "name or relative path"=w241:string)  [unwired: 15 in]
                }
                frame "do not save" {
                }
              }
            }
            frame "Plot frequency shift" {
              (unwired) T26."background"
              (unwired) enum16{"Time", "temperature", "field", "angle"}."angle"
              w261 = 1000000 ("requested size")
              # "omega (Hz)"
              # "time (min)"
              n114 = Unbundle By Name(w279) -> ("omega(0)"=w283:dbl, "Gamma"=w282:dbl, "phase"=w265:dbl, "z (inf)"=w263:cdb)
              n115 = call <vilib>:"High Resolution Relative Seconds.vi"() -> ("relative seconds"=w284:dbl)
              n116 = Divide(x=w284, y=60) -> (x/y=w286:dbl)
              n117 = Complex To Polar(r * e^(i*theta)=w263) -> (r=w262:dbl)  [unwired: 1 out]
              n118 = Multiply(y=60) -> (x=w281:i32, x*y=w288:i32)
              n119 = call "fancy torque read T .vi"() -> ("angle"=w271:dbl, "field"=w272:dbl, "temperature"=w278:dbl)  [unwired: 8 in, 1 out]
              n120 = Divide(x=w288) -> (y=w280:i32, x/y=w287:dbl)
              n121 = Round Toward +Infinity(x=w287) -> (ceil(x): smallest int >= x=w290:dbl)
              n122 = call "switch - C.vi"("switch"=TRUE) -> ("result"=w259:bool)  [unwired: 10 in]
              n123 = To Long Integer(number=w290) -> ()  [unwired: 1 out]
              n124 = call "aggregator - v - real.vi"("number"=w262, "init?"=w259, "requested size"=w261) -> ("Array"=w260:dbl[])  [unwired: 6 in, 2 out]
              n125 = call "aggregator - v - real.vi"("number"=w265, "init?"=w259, "requested size"=w261) -> ("Array"=w264:dbl[])  [unwired: 6 in, 2 out]
              n126 = call "aggregator - v - real.vi"("number"=w286, "init?"=w259, "requested size"=w261) -> ("Array"=w274:dbl[])  [unwired: 6 in, 2 out]
              n127 = call "aggregator - v - real.vi"("number"=w283, "init?"=w259, "requested size"=w261) -> ("Array"=w267:dbl[])  [unwired: 6 in, 2 out]
              n128 = call "aggregator - v - real.vi"("number"=w282, "init?"=w259, "requested size"=w261) -> ("Array"=w266:dbl[])  [unwired: 6 in, 2 out]
              n129 = call "aggregator - v - real.vi"("number"=w278, "init?"=w259, "requested size"=w261) -> ("Array"=w276:dbl[])  [unwired: 6 in, 2 out]
              n130 = call "aggregator - v - real.vi"("number"=w272, "init?"=w259, "requested size"=w261) -> ("Array"=w273:dbl[])  [unwired: 6 in, 2 out]
              n131 = call "aggregator - v - real.vi"("number"=w271, "init?"=w259, "requested size"=w261) -> ("Array"=w270:dbl[])  [unwired: 6 in, 2 out]
              n132 = case shown="\"angle\"" w277 {
                tunnel: w276 -> [_ w299 _ _]
                tunnel: [w298 w299 w300 w301] -> w275
                tunnel: w274 -> [w298 _ _ _]
                tunnel: w273 -> [_ _ w300 _]
                tunnel: w270 -> [_ _ _ w301]
                frame "Time", Default {
                }
                frame "temperature" {
                }
                frame "field" {
                }
                frame "angle" {
                }
              }
              n133 = case shown="\"gamma\"" w269 {
                tunnel: w266 -> [_ w295 _ _]
                tunnel: [w294 w295 w296 w297] -> w268
                tunnel: w267 -> [w294 _ _ _]
                tunnel: w264 -> [_ _ w296 _]
                tunnel: w260 -> [_ _ _ w297]
                frame "frequency", Default {
                }
                frame "gamma" {
                }
                frame "phase" {
                }
                frame "background" {
                }
              }
              n134 = Bundle("Array"=w275, "Array"=w268) -> ()  [unwired: 1 in, 1 out]
            }
            frame "save data" {
              n135 = call <vilib>:"High Resolution Relative Seconds.vi"() -> ("relative seconds"=w305:dbl)
              n136 = call "fancy torque read T .vi"() -> ("angle"=w302:dbl, "field"=w304:dbl, "temperature"=w303:dbl)  [unwired: 8 in, 1 out]
              n137 = call "switch - C.vi"("switch"=TRUE) -> ()  [unwired: 10 in, 1 out]
              n138 = call "KM_appendline.vi"("Time (s)"=w305, "temperature"=w303, "Field"=w304, "angle (deg)"=w302, "pm lorentzian"=w306, "Save frequency scan"=w307, "read/write control"=KM_file_--_read-write_control."append one line") -> ("name or relative path"=w308:string)  [unwired: 12 in]
            }
            frame "save freq scan" {
              n139 = local read item#-1() -> (w314)
              n140 = call "filename-manage.vi"("filename pattern"=w314, "filename-action"=filename-action."parse") -> ("filename OUT"=w313:string, "file name"=w315:string)  [unwired: 8 in]
              n141 = local write item#-1(w313) -> ()
              n142 = call "KM_appendline -- freq sweep.vi"("freq"=w318, "Vout(V)"=w317, "Save frequency scan"=w319, "read/write control"=KM_file_--_read-write_control."append one line", "name or relative path"=w313) -> ()  [unwired: 15 in]
            }
            frame "Update range" {
              n143 = Unbundle By Name(w336) -> ("omega(0)"=w327:dbl, "Gamma"=w334:dbl)
              n144 = call "cursor window logic V3.vi"("cursor window action"=cursor_window_action."read", "cursor window in"=w329) -> ("cursor window out"=w332:T8)  [unwired: 8 in, 1 out]
              n145 = Unbundle By Name(w332) -> ("left"=w331:dbl, "right"=w330:dbl, "window"=w324:dbl)
              n146 = Multiply(x=w324, y=3.0 ("lower")) -> (x*y=w325:dbl)
              n147 = Multiply(x=w324, y=0.0003 ("lower")) -> (x*y=w322:dbl)
              n148 = call "Q -- check range -- i -- real.vi"("upper"=w330, "lower"=w331, "number"=w327) -> ("in range?"=w335:bool)  [unwired: 6 in, 2 out]
              n149 = call "Q -- check range -- i -- real.vi"("upper"=w325, "lower"=w322, "number"=w334) -> ("in range?"=w333:bool)  [unwired: 6 in, 2 out]
              n150 = And(x=w335, y=w333) -> (x .and. y?=w328:bool)
              "fit is fine" <- w328
              n151 = case shown="True" w328 {
                tunnel: w334 -> [_ w348]
                tunnel: w327 -> [_ w342]
                tunnel: w338 -> [_ w349]
                tunnel: w337 -> [_ _]
                frame False {
                }
                frame True {
                  (unwired) agregator_--_action."append" ("aggregator action")
                  n152 = Compound Arithmetic op=MULTIPLY("gamma factor", w348, 2.0 ("value")) -> (w346:dbl)
                  n153 = for {
                    N: 1 -> [_]
                    tunnel: "history length" -> [w353]
                    tunnel: w342 -> [w358]
                    shift-right: [w354] -> _
                    shift-left: _ -> [w357]
                    tunnel: [w351] -> w341
                    n154 = call "aggregator - vii - real - atomic.vi"("aggregator action"=agregator_--_action."append", "requested size"=w353, "number"=w358, "state IN"=w357) -> ("state OUT"=w355:T24)  [unwired: 4 in, 3 out]
                    n155 = call "aggregator - vii - real - atomic.vi"("aggregator action"=agregator_--_action."interpolate", "requested size"=w353, "state IN"=w355) -> ("interp average"=w351:dbl, "state OUT"=w354:T24)  [unwired: 5 in, 2 out]
                  }
                  n156 = call "cursor window logic V3.vi"("cursor window action"=cursor_window_action."change cen&win", "window"=w346, "center"=w341, "cursor window in"=w349) -> ()  [unwired: 6 in, 2 out]
                }
              }
            }
            frame "Fit" {
              n157 = case shown="True" "fit?" {
                tunnel: w364 -> [_ w380]
                tunnel: w363 -> [_ w378]
                tunnel: w362 -> [_ w376]
                tunnel: w361 -> [_ w373]
                tunnel: [T6 {"Amplitude"=-1.0311345636926572, "omega(0)"=-1.0311345636926572, "Gamma"=-1.0311345636926572, "phase"=-1.0311345636926572, "Q"=-1.0311345636926572, "Norm  Ampl"=-1.0311345636926572, "z (inf)"=-1.0311345636926572+0.0i, "4corners"={"z (-pi/2)"=-1.0311345636926572+0.5736824521422934i, "z(inf)"=-0.5200164984937075+1.0975277942502903i, "z (pi/2)"=-1.0311345636926572+0.5736824521422934i, "z center"=-0.5136528600391839+0.580046090596817i, "z(0)"=-0.5200164984937075+1.0975277942502903i, "radius"=-1.0311345636926572}} ("pm lorentzian") w372] -> w360
                frame False {
                }
                frame True {
                  n158 = call "cursor window logic V3.vi"("cursor window action"=cursor_window_action."read", "cursor window in"=w378) -> ("cursor window out"=w374:T8)  [unwired: 8 in, 1 out]
                  n159 = Increment(x="some") -> (x+1=w366:dbl)
                  n160 = local write "some"(w366) -> ()
                  n161 = call "acquire cursor window data.vi"("z in"=w373, "omega in"=w376, "cursor window"=w374) -> ("z out"=w375:cdb[], "omega  out"=w377:dbl[])  [unwired: 4 in, 3 out]
                  n162 = call "KM_peak -- find -- pm - V1.vi"("omega in"=w377, "z in"=w375, "parameters: complex fit"="parameters: complex fit", "plots: filter related"=w380, "plot staff ?"="plot staff", "just guess?"="use fast fit?", "subtract linear BG"=FALSE) -> ("pm lorentzian"=w372:T6)  [unwired: 10 in, 2 out]
                  n163 = local write "pm lorentzian"(w372) -> ()
                  n164 = Unbundle By Name(w372) -> ("omega(0)"=→"circle frequency (Hz)":dbl, "Gamma"=→"circle gamma (Hz)":dbl, "phase"=→"circle phase (rad)":dbl, "Q"=→"circle Q":dbl)
                }
              }
              n165 = disable-structure shown="Disabled" {
                disable-tunnel: w360 -> [w393 _]
                disable-tunnel: w361 -> [w392 _]
                frame Disabled {
                  n166 = for {
                    tunnel: four-corner_circle_transformation."to  canonical" ("4 corner circle transformation") -> [w401]
                    tunnel: w393 -> [w400]
                    tunnel: w392 -> [w399] mode=indexing
                    tunnel: [w398] -> w391 mode=indexing
                    n167 = call "lorentzian transformations.vi"("4 corner circle transformation"=w401, "lorentzian in"=w400, "voltage in"=w399) -> ("voltage out"=w398:cdb)  [unwired: 6 in, 2 out]
                  }
                  n168 = Complex To Polar(r * e^(i*theta)=w391) -> (theta=w389:dbl[])  [unwired: 1 out]
                  n169 = Complex To Re/Im(x + iy=w391) -> (x=w395:dbl[], y=w396:dbl[])
                  n170 = Bundle(w395, w396) -> ()  [unwired: 1 in, 1 out]
                  n171 = Add(x=w389, y=1.5707963267948966) -> (x+y=w387:dbl[])
                  n172 = Array Size(array=w387) -> (size(s)=w388:i32)
                  n173 = for {
                    N: w388 -> [_]
                    tunnel: [w397] -> w386 mode=indexing
                    i -> [w397]
                  }
                  n174 = Bundle(w386, w387) -> (w385:cluster{i32[], dbl[]})  [unwired: 1 in]
                }
                frame Enabled {
                }
              }
            }
            frame "Void", Default {
            }
          }
        }
      }
      event Timeout {
        n175 = event-data() -> ()  [unwired: 1 in, 2 out]
      }
    }
    n176 = Wait (ms)(milliseconds to wait=u32 0) -> ()  [unwired: 1 out]
  }
  n177 = while {
    tunnel: w44 -> [w411]
    tunnel: w31 -> [w409]
    tunnel: w1 -> [w408]
    tunnel: w2 -> [w405]
    stop <- FALSE stop-if-true
    n178 = local read "pm lorentzian"() -> (w407:T6)
    n179 = local read "MFLI mode"() -> (w404:T1)
    n180 = event shown="[1] \"Plot: circle sweep window\": Cursor Move" {
      selector: w411 -> [_ _ _ _ _ _ _ _ _]
      dyn-events: _ -> [_ _ _ _ _ _ _ _ _]
      timeout: _ -> [_ _ _ _ _ _ _ _ _]
      tunnel: w409 -> [_ w413 w434 _ w443 _ _ w474 w532]
      tunnel: [_ _ _ _ _ _ _ _ "Update system parameters"] -> _
      tunnel: w408 -> [_ w416 w433 _ _ _ _ w470 _]
      tunnel: w407 -> [_ _ _ _ _ w448 w459 _ _]
      tunnel: w405 -> [_ w414 _ _ _ _ _ w469 _]
      tunnel: [_ _ _ "refresh" _ _ _ _ _] -> _
      tunnel: w404 -> [_ w412 w432 _ _ _ _ _ _]
      event Timeout {
        n181 = event-data() -> ()  [unwired: 1 in, 2 out]
      }
      event "Plot: circle sweep window": Cursor Move {
        n182 = event-data() -> ("CursIdx"=w415:i32)  [unwired: 1 in, 8 out]
        n183 = case shown="0..2" w415 {
          selector: w415 -> [w424 w430]
          tunnel: w416 -> [w426 _]
          tunnel: w414 -> [_ w429]
          tunnel: w413 -> [w418 _]
          tunnel: w412 -> [w417 _]
          frame 0..2 {
            n184 = call "cursor window logic V3.vi"("CursIdx"=w424, "cursor window action"=cursor_window_action."cursor moves", "cursor window in"=w426) -> ("cursor window out"=w423:T8)  [unwired: 7 in, 1 out]
            n185 = Unbundle By Name(w423) -> ("left"=→"left freq (Hz)":dbl, "right"=→"right freq (Hz)":dbl, "center"=→"center freq (Hz)":dbl, "window"=→"window  (Hz)":dbl)
            n186 = case shown="\"read\", Default" w417 {
              tunnel: w418 -> [w428 _]
              frame "circles sweep" {
                w427 = "Fit"  # event data
                n187 = Generate User Event(user event=w428, event data cluster=w427) -> ()  [unwired: 2 in, 2 out]
              }
              frame "read", Default {
              }
            }
          }
          frame 3..5, Default {
            n188 = call "cursor window logic V3.vi"("CursIdx"=w430, "cursor window action"=cursor_window_action."cursor moves", "cursor window in"=w429) -> ()  [unwired: 7 in, 2 out]
          }
        }
      }
      event "center freq (Hz)": Value Change {
        n189 = event-data() -> ()  [unwired: 1 in, 6 out]
        n190 = local read "center freq (Hz)"() -> (w435:dbl)
        n191 = case shown="\"circles sweep\"" w432 {
          tunnel: w434 -> [w438 _]
          frame "circles sweep" {
            n192 = Generate User Event(user event=w438, event data cluster="Fit" ("event data")) -> ()  [unwired: 2 in, 2 out]
          }
          frame "read", Default {
          }
        }
        n193 = call "cursor window logic V3.vi"("cursor window action"=cursor_window_action."change cen&win", "center"=w435, "cursor window in"=w433) -> ()  [unwired: 7 in, 2 out]
      }
      event "refresh": Value Change {
        n194 = event-data() -> ()  [unwired: 1 in, 6 out]
        n195 = local read "reqested size"() -> (w439:i64)
        n196 = call "fucking PID.vi"("requested size"=w439, "PID action"=agregator_--_action."init") -> ()  [unwired: 6 in, 4 out]
      }
      event "Plot: circle sweep window": Cursor Release {
        n197 = event-data() -> ("CursIdx"=w442:i32)  [unwired: 1 in, 8 out]
        n198 = case shown="3, Default" w442 {
          tunnel: w443 -> [_ w444]
          frame 3, Default {
          }
          frame 0..2 {
            w445 = "Fit"  # event data
            n199 = Generate User Event(user event=w444, event data cluster=w445) -> ()  [unwired: 2 in, 2 out]
          }
        }
      }
      event "scale gauge: Plot: complex plane": Value Change {
        n200 = event-data() -> ("NewVal"=w447:dbl)  [unwired: 1 in, 5 out]
        n201 = Unbundle By Name(w448) -> ()  [unwired: 1 out]
        n202 = Unbundle By Name(w448) -> ("4corners.z center"=w449:cdb)
        n203 = control-ref of="Plot: complex plane"() -> (w446:refnum<vi>)
        n204 = Complex To Re/Im(x + iy=w449) -> (x=w450:dbl, y=w451:dbl)
        n205 = Negate(x=w447) -> (-x=w456:dbl)
        n206 = Add(x=w451, y=w456) -> (x+y=w452:dbl)
        n207 = Add(x=w450, y=w447) -> (x+y=w454:dbl)
        n208 = Add(x=w450, y=w456) -> (x+y=w455:dbl)
        n209 = Add(x=w451, y=w447) -> (x+y=w453:dbl)
        n210 = property on="Property Node" class="XYGraph (strict)"(reference=w446, "XScale.Minimum"=w455, "XScale.Maximum"=w454, "YScale.Maximum"=w453, "YScale.Minimum"=w452) -> ()  [unwired: 1 in, 2 out]
      }
      event "scale gauge: Plot: complex plane - filter": Value Change {
        n211 = event-data() -> ("NewVal"=w458:dbl)  [unwired: 1 in, 5 out]
        n212 = Unbundle By Name(w459) -> ()  [unwired: 1 out]
        n213 = Unbundle By Name(w459) -> ("4corners.z center"=w460:cdb)
        n214 = control-ref of="Plot: complex plane - filter"() -> (w457:refnum<vi>)
        n215 = Complex To Re/Im(x + iy=w460) -> (x=w461:dbl, y=w462:dbl)
        n216 = Negate(x=w458) -> (-x=w467:dbl)
        n217 = Add(x=w462, y=w467) -> (x+y=w463:dbl)
        n218 = Add(x=w461, y=w458) -> (x+y=w465:dbl)
        n219 = Add(x=w461, y=w467) -> (x+y=w466:dbl)
        n220 = Add(x=w462, y=w458) -> (x+y=w464:dbl)
        n221 = property on="Property Node" class="XYGraph (strict)"(reference=w457, "XScale.Minimum"=w466, "XScale.Maximum"=w465, "YScale.Maximum"=w464, "YScale.Minimum"=w463) -> ()  [unwired: 1 in, 2 out]
      }
      event Key Down {
        n222 = event-data() -> ("Char"=w472:i16, "VKey"=w475:T13)  [unwired: 1 in]
        "Char" <- w472
        "VKey" <- w475
        n223 = local read "MFLI mode"() -> (w468:T1)
        n224 = Build Array(w472) -> (w473:i16[])
        n225 = Byte Array To String(unsigned byte array=w473) -> (string=w471:string)
        n226 = case shown="\"Up\"..\"Right\"" w475 {
          selector: w475 -> [_ _ _ _ w523]
          tunnel: w472 -> [_ _ _ _ _]
          tunnel: w474 -> [w479 _ _ _ w522]
          tunnel: w471 -> [w478 _ _ _ _]
          tunnel: w470 -> [w477 _ _ _ w515]
          tunnel: w469 -> [w476 _ _ _ _]
          tunnel: w468 -> [_ _ _ _ w514]
          frame "ASCII", Default {
            n227 = case shown="\"s\"" w478 {
              selector: w478 -> [_ _ _ _ w487 _ _ _]
              tunnel: w479 -> [_ _ w482 _ _ _ _ _]
              tunnel: w477 -> [_ w480 _ w484 w488 w495 w498 w513]
              tunnel: w476 -> [_ _ _ _ _ w493 _ _]
              frame "0", Default {
              }
              frame "a" {
                n228 = call "cursor window logic V3.vi"("cursor window action"=cursor_window_action."zoom to all data", "cursor window in"=w480) -> ()  [unwired: 8 in, 2 out]
              }
              frame "s" {
                n229 = Generate User Event(user event=w482, event data cluster="save freq scan" ("event data")) -> ()  [unwired: 2 in, 2 out]
              }
              frame "?" {
                # "?"
                n230 = call "cursor window logic V3.vi"("cursor window action"=cursor_window_action."zoom X", "cursor window in"=w484) -> ()  [unwired: 8 in, 2 out]
              }
              frame "+", "-", "<", ">" {
                # "?"
                n231 = case shown="\"+\", Default" w487 {
                  tunnel: [cursor_window_action."slide right" ("cursor window action") cursor_window_action."slide left" ("cursor window action") cursor_window_action."zoom in" ("cursor window action") cursor_window_action."zoom out" ("cursor window action")] -> w486
                  frame ">" {
                  }
                  frame "<" {
                  }
                  frame "+", Default {
                  }
                  frame "-" {
                  }
                }
                n232 = call "cursor window logic V3.vi"("cursor window action"=w486, "cursor window in"=w488) -> ()  [unwired: 8 in, 2 out]
              }
              frame "c" {
                n233 = call "cursor window logic V3.vi"("cursor window action"=cursor_window_action."check", "cursor window in"=w495) -> ()  [unwired: 8 in, 2 out]
                n234 = call "cursor window logic V3.vi"("cursor window action"=cursor_window_action."check", "cursor window in"=w493) -> ()  [unwired: 8 in, 2 out]
              }
              frame "t" {
                n235 = local read "talk to MFLI !"() -> (w497:bool)
                n236 = case shown="True" w497 {
                  tunnel: w498 -> [_ w504]
                  frame False {
                  }
                  frame True {
                    n237 = local read "Auto-update sweep window!"() -> (w503:bool)
                    n238 = Not(x=w503) -> (.not. x?=w502:bool)
                    n239 = local write "Auto-update sweep window!"(w502) -> ()
                    n240 = Select(t=cursor_window_action."color--green" ("cursor window action"), s=w502, f=cursor_window_action."color--red" ("cursor window action")) -> (s? t:f=w499:T15)
                    n241 = call "cursor window logic V3.vi"("cursor window action"=w499, "cursor window in"=w504) -> ()  [unwired: 8 in, 2 out]
                  }
                }
              }
              frame "r" {
                n242 = local read "Auto-update sweep window!"() -> (w508:bool)
                n243 = local read "talk to MFLI !"() -> (w509:bool)
                n244 = Not(x=w509) -> (.not. x?=w512:bool)
                n245 = Select(t=cursor_window_action."color--green" ("cursor window action"), s=w508, f=cursor_window_action."color--red" ("cursor window action")) -> (s? t:f=w505:T15)
                n246 = Select(t=w505, s=w512, f=cursor_window_action."color--yellow" ("cursor window action")) -> (s? t:f=w510:T15)
                n247 = local write "talk to MFLI !"(w512) -> ()
                n248 = call "cursor window logic V3.vi"("cursor window action"=w510, "cursor window in"=w513) -> ()  [unwired: 8 in, 2 out]
              }
            }
          }
          frame "Escape" {
          }
          frame "PageUp" {
          }
          frame "PageDown" {
          }
          frame "Up".."Right" {
            n249 = case shown="\"Left\"" w523 {
              tunnel: [cursor_window_action."move right" ("cursor window action") cursor_window_action."move left" ("cursor window action") cursor_window_action."broaden" ("cursor window action") cursor_window_action."shrink" ("cursor window action")] -> w517
              frame "Right", Default {
              }
              frame "Left" {
              }
              frame "Up" {
              }
              frame "Down" {
              }
            }
            n250 = call "cursor window logic V3.vi"("cursor window action"=w517, "cursor window in"=w515) -> ("cursor window out"=w516:T8)  [unwired: 8 in, 1 out]
            n251 = Unbundle By Name(w516) -> ("left"=w521:dbl, "right"=w520:dbl, "center"=w519:dbl, "window"=w518:dbl)
            n252 = case shown="\"read from disk\"" w514 {
              tunnel: w522 -> [w525 w527 _]
              frame "circles sweep" {
                w524 = "Fit"  # event data
                n253 = Generate User Event(user event=w525, event data cluster=w524) -> ()  [unwired: 2 in, 2 out]
              }
              frame "read from disk" {
                w526 = "Fit"  # event data
                n254 = Generate User Event(user event=w527, event data cluster=w526) -> ()  [unwired: 2 in, 2 out]
              }
              frame "read", Default {
              }
            }
            n255 = local write "right freq (Hz)"(w520) -> ()
            n256 = local write "center freq (Hz)"(w519) -> ()
            n257 = local write "window  (Hz)"(w518) -> ()
            n258 = local write "left freq (Hz)"(w521) -> ()
          }
        }
      }
      event "Update system parameters": Value Change {
        n259 = event-data() -> ()  [unwired: 1 in, 6 out]
        n260 = Generate User Event(user event=w532, event data cluster="Update system parameters" ("event data")) -> ()  [unwired: 2 in, 2 out]
      }
    }
    n261 = Wait (ms)(milliseconds to wait=u32 0) -> ()  [unwired: 1 out]
  }
